vi "MainInterface.vi"() -> ()   [LabVIEW 2016]
uses:
  CurrentSwitchValues_GlobalVariable.vi
  TCPRead_Write_GlobalVariables.vi
panel:
  out "Progress #":i32
  in  "Refresh Fraction [%]":dbl=30.0 min=0.0 max=100.0 step=1.0
  in  "DNA  High RR":dbl=0.25 min=0.0 max=1.0 step=0.001
  in  "Number of Dilution Cycles":dbl=120.0
  in  "Number of Mixing Cycles Initialisation":dbl=4.0
  in  "Time between Mixing Cycles Initialisation":dbl
  in  "FB RR":dbl=0.75 min=0.0 max=1.0 step=0.001
  in  "FB":dbl=8.0 min=1.0 max=9.0 step=1.0
  in  "DNA Channel":dbl=5.0 min=1.0 max=9.0 step=1.0
  in  "Fluorophore RR":dbl min=0.0 max=1.0 step=0.001
  in  "Elution Buffer RR":dbl=0.25 min=0.0 max=1.0 step=0.001
  in  "Fluorophore":dbl=1.0 min=1.0 max=9.0 step=1.0
  in  "Elution Buffer":dbl=2.0 min=1.0 max=9.0 step=1.0
  out "Running Experiments":bool
  in  "Number of Inflow Steps":dbl=15.0
  out "Chamber 7":dbl
  out "Chamber 6":dbl
  out "Chamber 5":dbl
  out "Chamber 4":dbl
  out "Chamber 3":dbl
  out "Chamber 2":dbl
  out "Chamber 1":dbl
  out "Chamber 8":dbl
  out "Running Calibration":bool=TRUE
  out "Duration (min)":i32
  out "Refresh Ratio":dbl format="%#_13g"
  in  "Number of Mixing Cycles":dbl=4.0
  in  "Fluorophore Channel":dbl=1.0 min=1.0 max=9.0 step=1.0
  in  "Elution Buffer Channel":dbl=2.0 min=1.0 max=9.0 step=1.0
  in  "Number of Dilution Steps":dbl=10.0
  in  "Time between Mixing Cycles":dbl
  in  "Perform Initial Calibration":bool
  out "Time since \nstart (sec)":dbl format="%#_4g"
  in  "Perform \nExperiments":bool
  out "Progress":i32(slide) max=6 scale=0.0..200.0
  out "Progress":i32(slide) max=25 scale=0.0..200.0
  in  "Ring 8":bool
  in  "Ring 7":bool
  in  "Ring 6":bool
  in  "Ring 5":bool
  in  "Ring 4":bool
  in  "Ring 3":bool
  in  "Ring 2":bool
  in  "Ring 1":bool
  in  "Load 20%":bool
  in  "Fully Load Chambers":bool
  in  "Load \nChannel":dbl=1.0 min=1.0 max=9.0
  out "Time Stamp":timestamp
  out "TCP Error Out":errorcluster
  out "TCP Output":string
  in  "Flush Slow":bool
  in  "Flush \nChannel":dbl=1.0 min=1.0 max=9.0
  in  "Flush Fast":bool
  out "Time since start (sec)":dbl format="%#_4g"
  out "Cycles completed":i32(slide) max=6 scale=0.0..1.0
  in  "Interval (min)":dbl=1.0
  in  "Number Of \nMix Cycles":dbl=1.0
  in  "Mix Chambers":bool
  out "Units 7/8":u8 format="%x"
  out "Units 5/6":u8 format="%x"
  out "Units 3/4":u8 format="%x"
  out "Units 1/2":u8 format="%x"
  out "Bytes Written (Total)":i32
  out "Bytes Written (Per Command)":i32
  in  "stop":bool
  in  "30":bool
  in  "24":bool
  in  "18":bool
  in  "12":bool
  in  "29":bool
  in  "23":bool
  in  "17":bool
  in  "10":bool
  in  "27":bool
  in  "20":bool
  in  "15":bool
  in  "25":bool
  in  "19":bool
  in  "13":bool
  in  "28":bool
  in  "22":bool
  in  "16":bool
  in  "11":bool
  in  "26":bool
  in  "21":bool
  in  "14":bool
  in  "9":bool
  in  "8":bool
  in  "6":bool
  in  "4":bool
  in  "2":bool
  in  "7":bool
  in  "5":bool
  in  "3":bool
  in  "1":bool
  in  "Timeout (ms)":u16=25
  in  "Port":u16=502
  in  "Address":string="192.168.1.100"
  # "Experimental Sequence"
  # "Air Filled Control Lines"
  # "Multiplexer"
  # "Inflow Speed Regulators"
  # "Ring Control"
  # "Misc."
  # "Channel Selection"
  # "Set Desired RR"
  # "Low Pressure Control \nchalles 4-8 Should Remain \nUnused. If Additional Air \nLines Are Required, The \nValves Can Be Found Under \nThis Tile."
  # "A Total Of 30 Valves (And \nThus Switches) Exist.\nCurrent Microfluidic Devices\nOnly Require 24 Control \nLines. As Such Valve 30 Has \nBeen Relegated."
  # "RRs for Multiple DNA Concentrations"
  # "Hexadceimal Values for WAGO Units 1-2, 3-4, 5-6, 7-8"
  # "Mixing Processes"
  # "Flushing"
  # "Loading"
  # "Perform Initial Calibration"
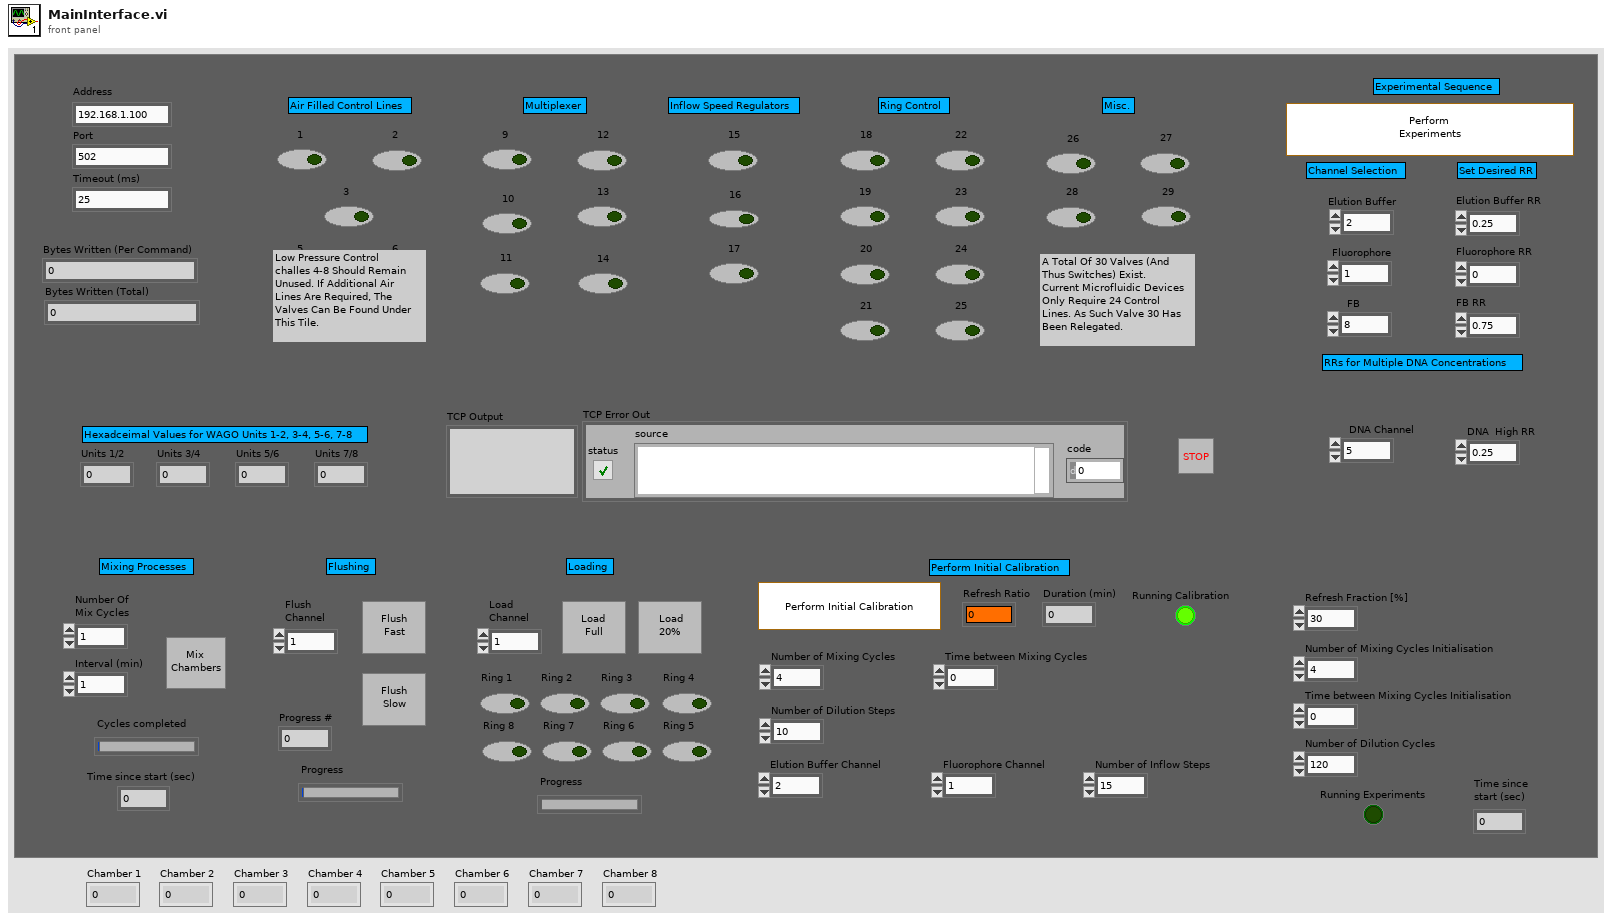
[diagram p1: front panel]
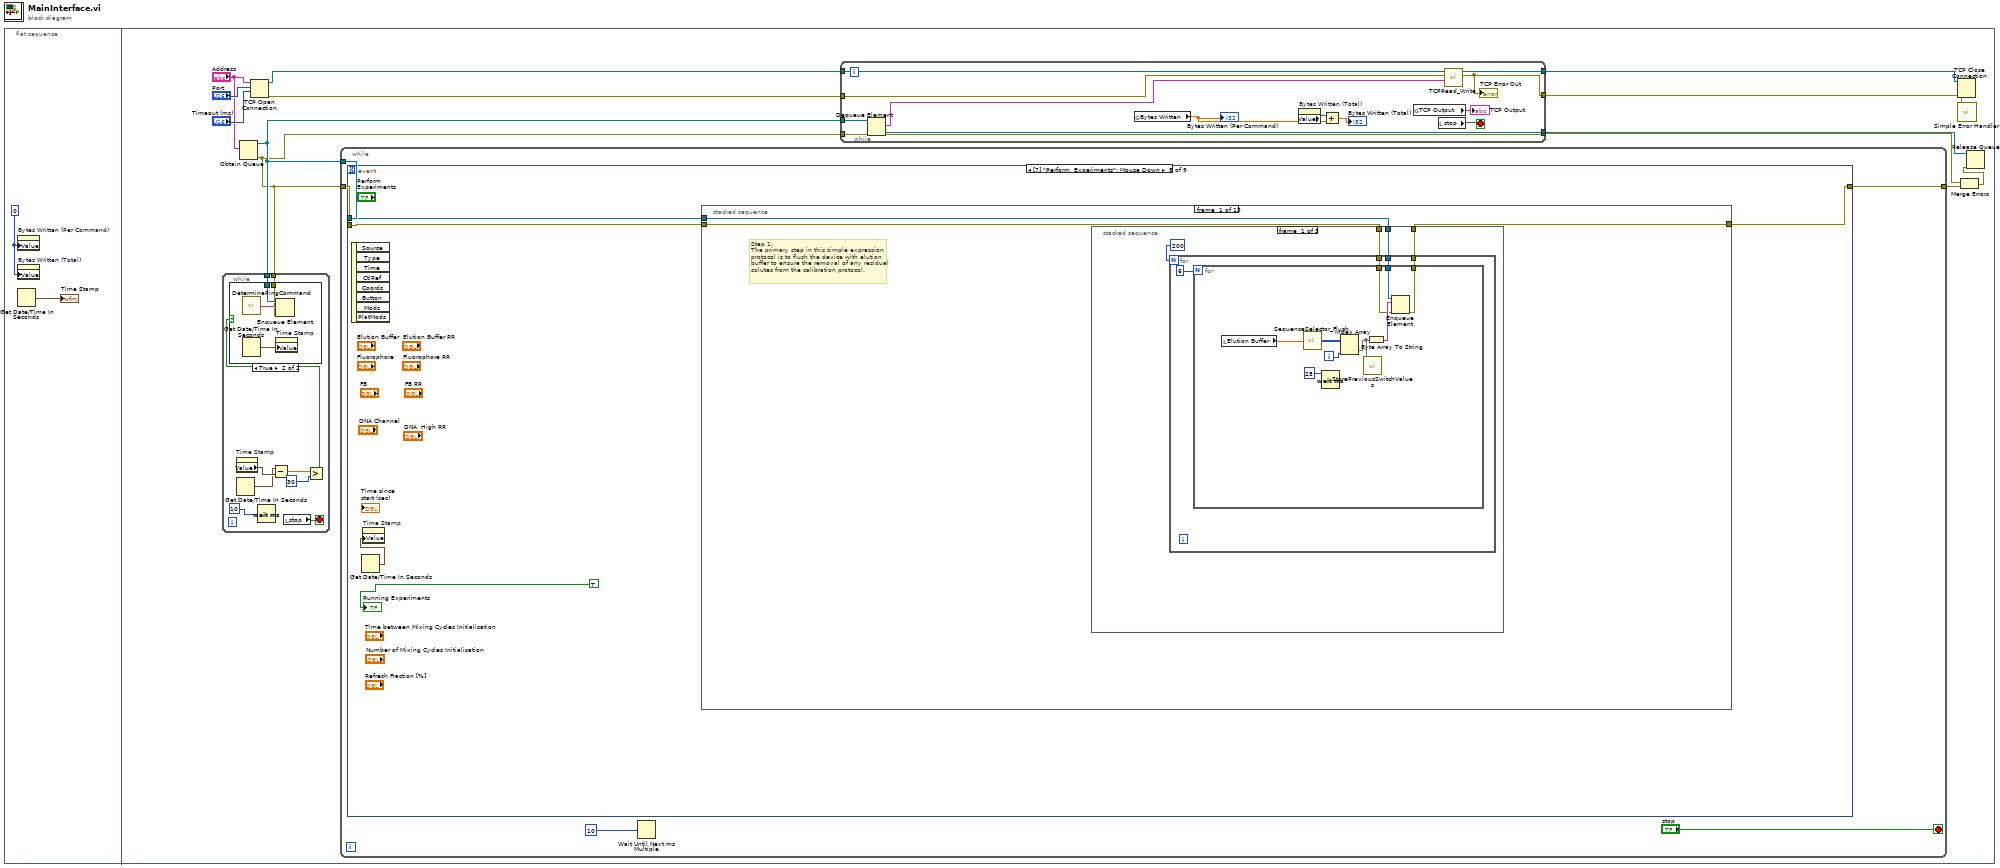
[diagram p0: block diagram]
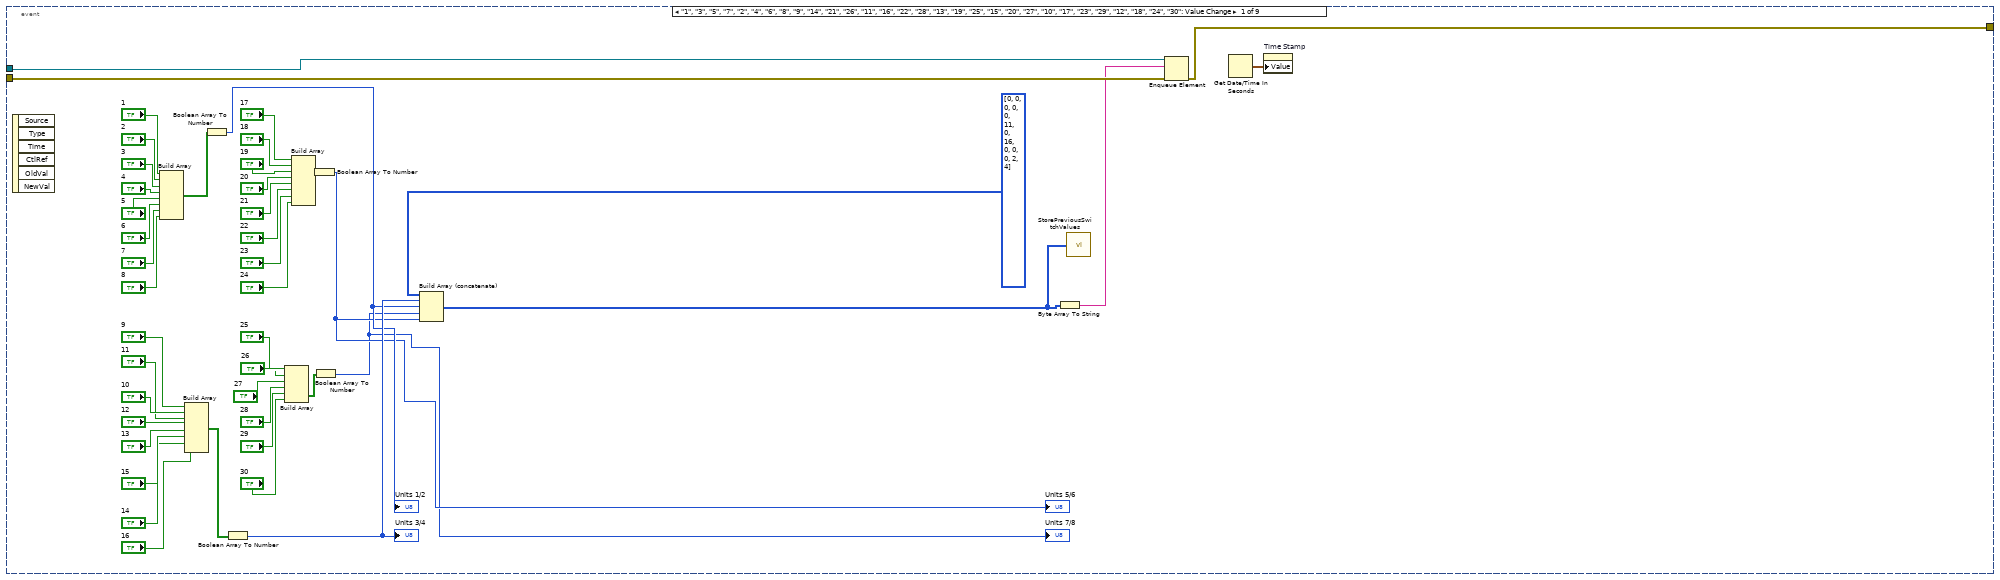
[diagram p3: hidden frame]
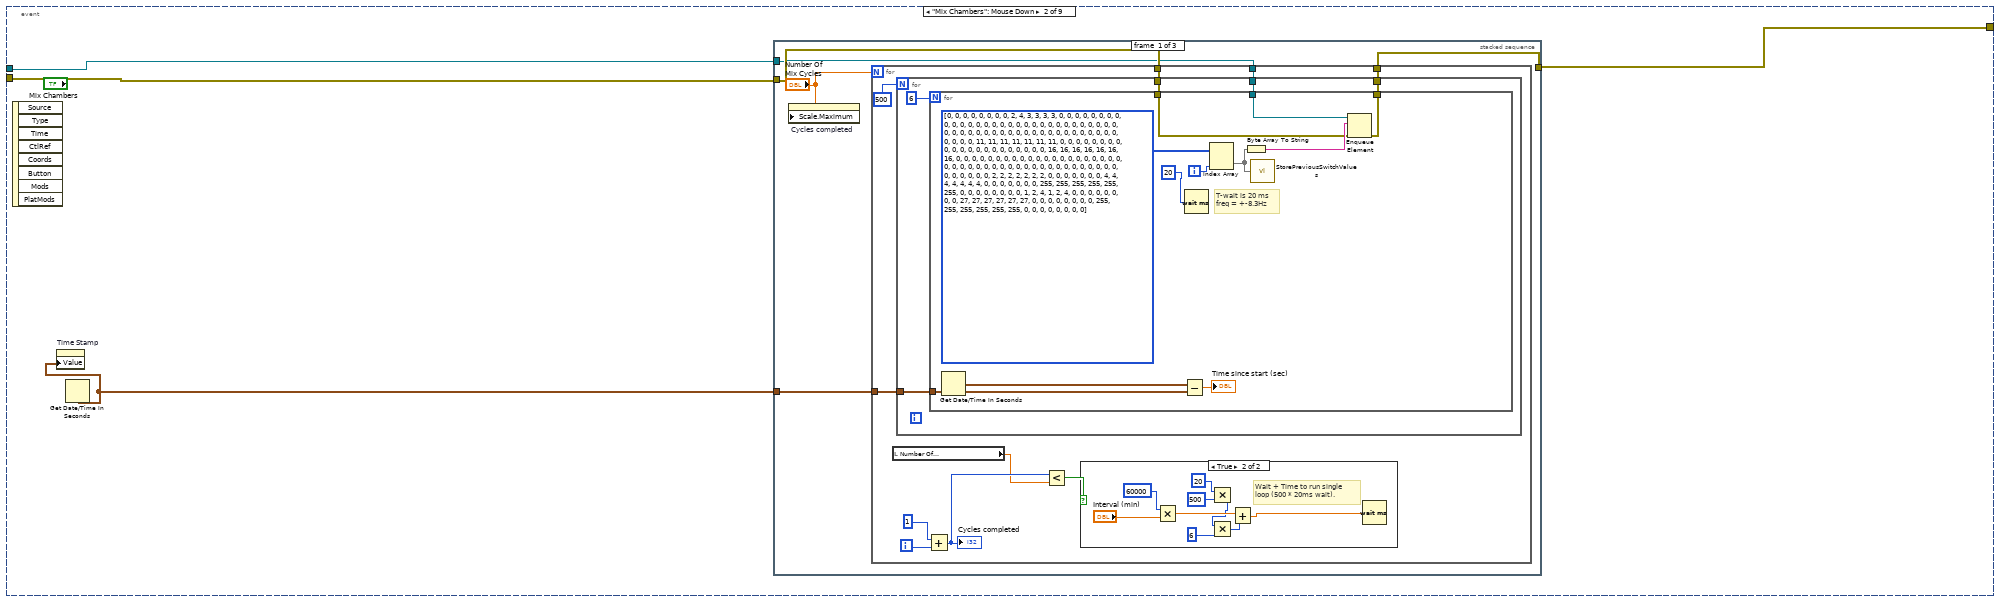
[diagram p4: hidden frame]
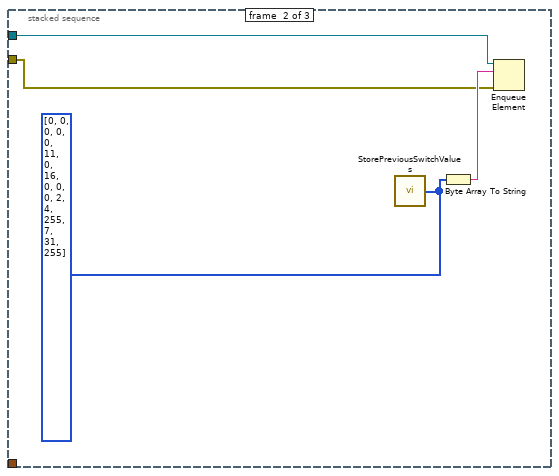
[diagram p6: hidden frame]
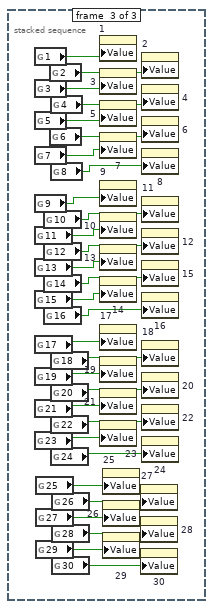
[diagram p7: hidden frame]
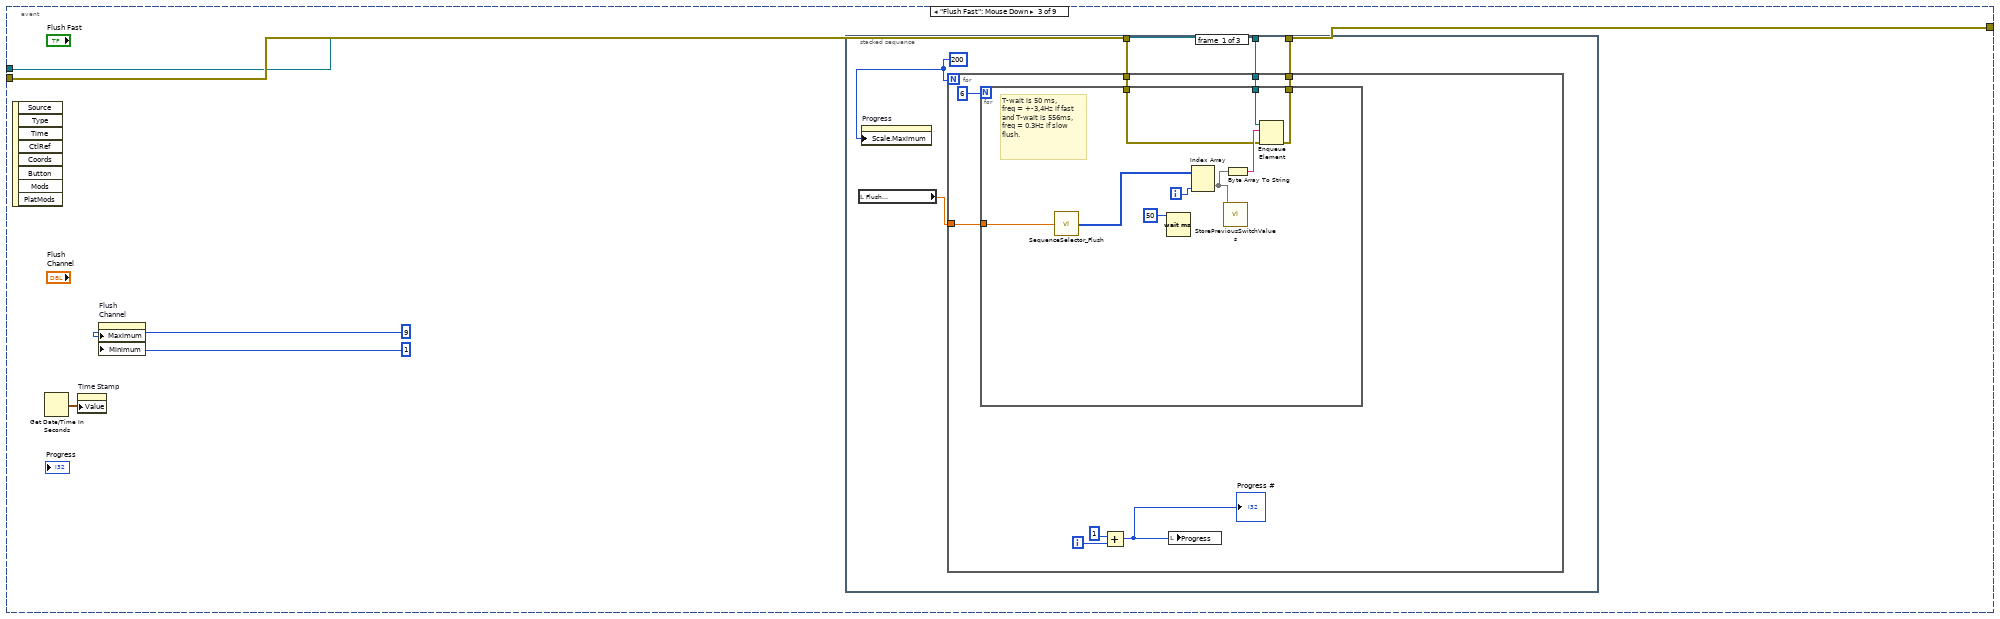
[diagram p8: hidden frame]
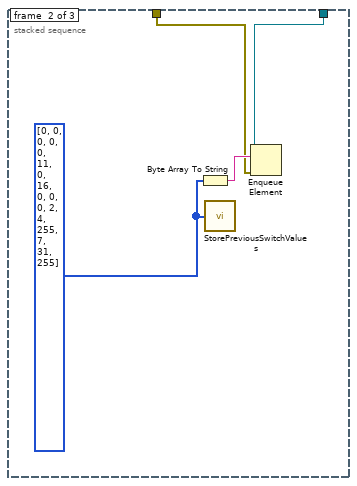
[diagram p9: hidden frame]
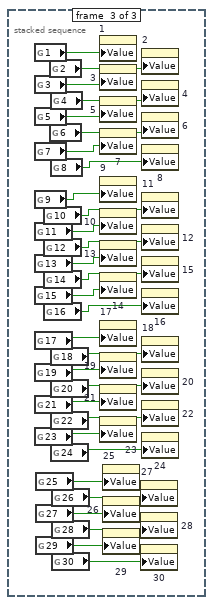
[diagram p10: hidden frame]
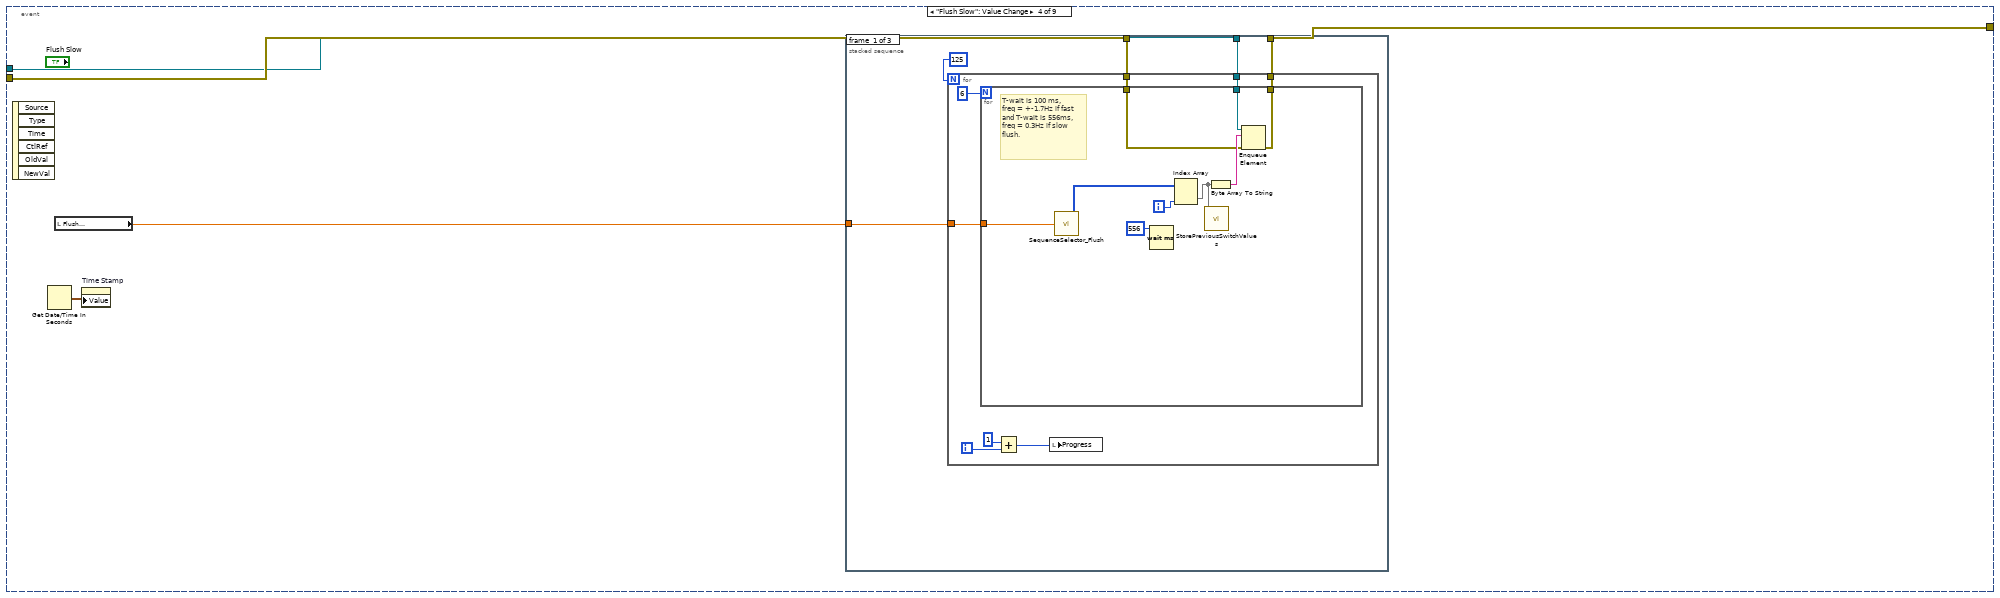
[diagram p11: hidden frame]
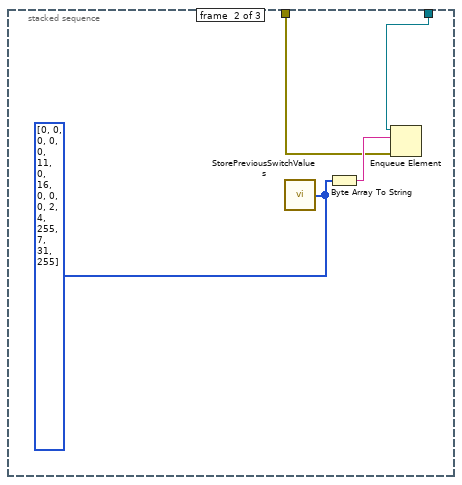
[diagram p12: hidden frame]
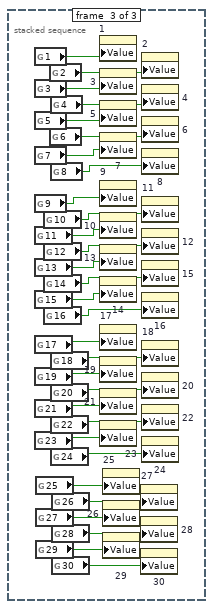
[diagram p13: hidden frame]
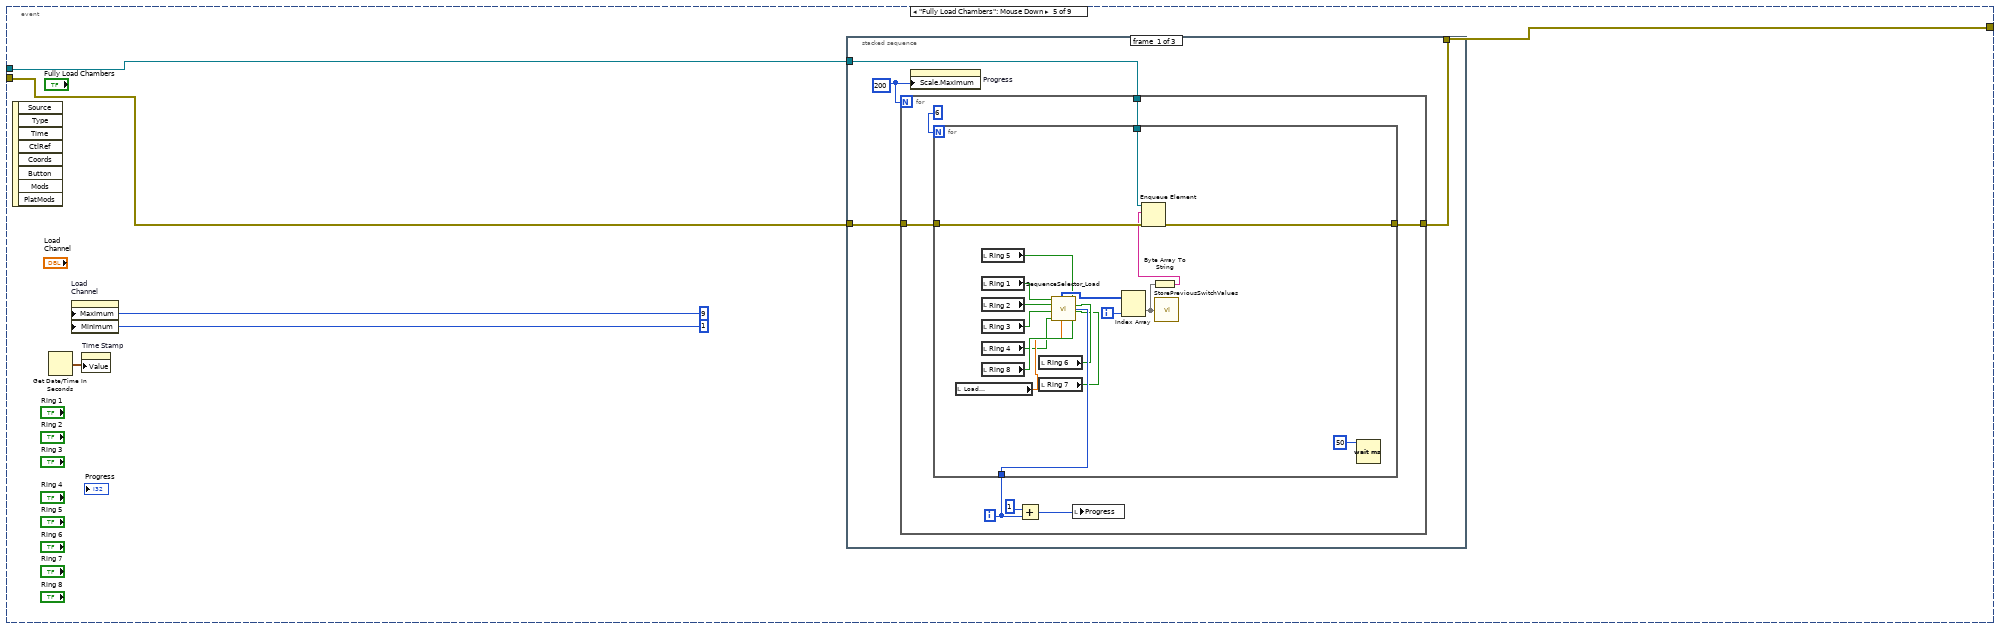
[diagram p14: hidden frame]
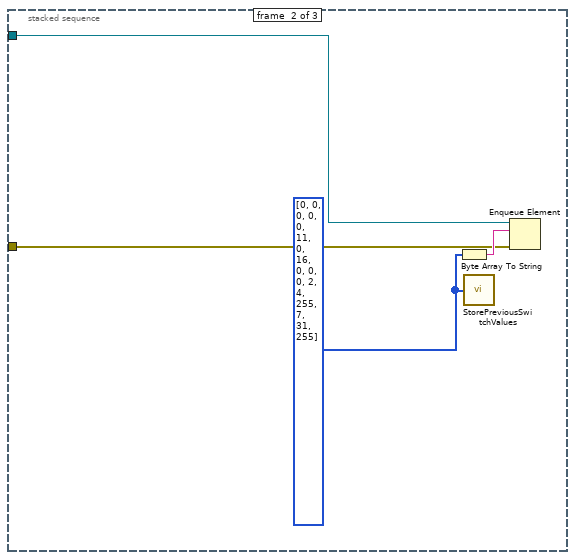
[diagram p15: hidden frame]
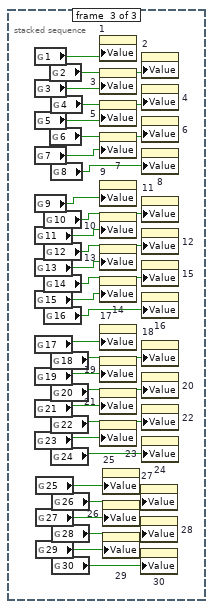
[diagram p16: hidden frame]
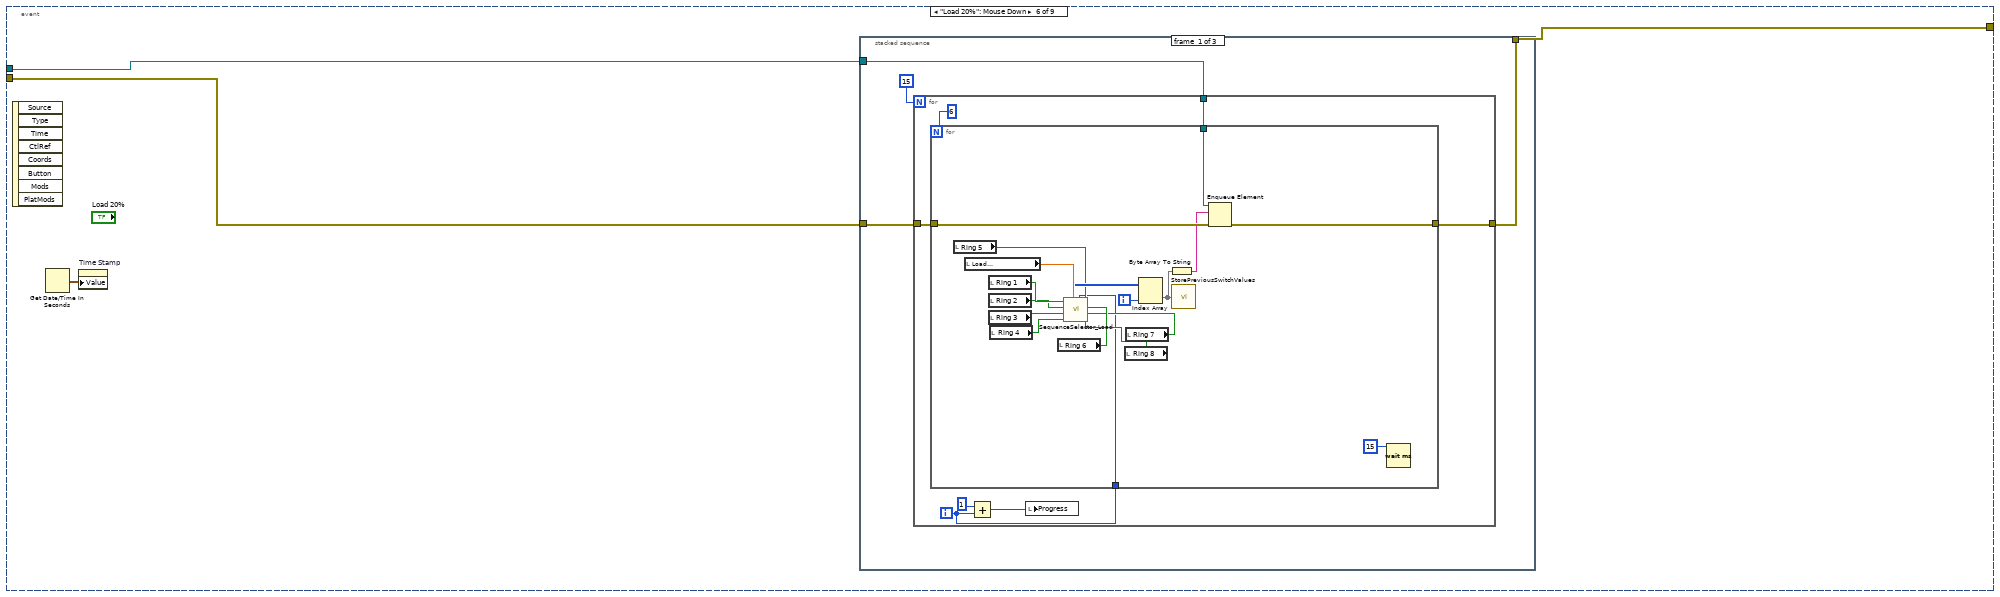
[diagram p17: hidden frame]
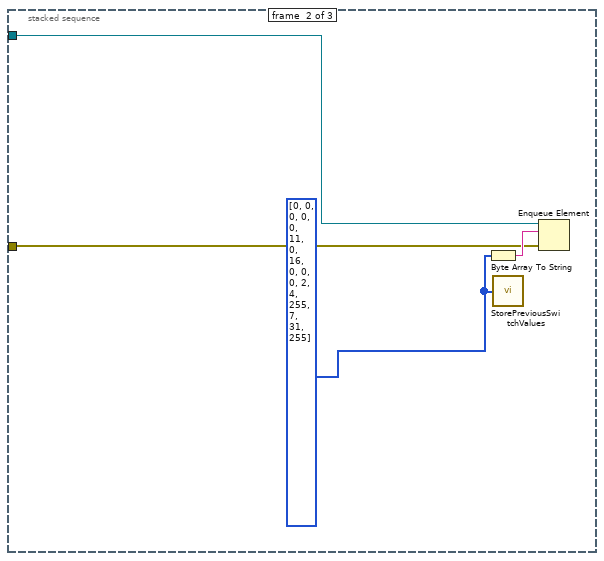
[diagram p18: hidden frame]
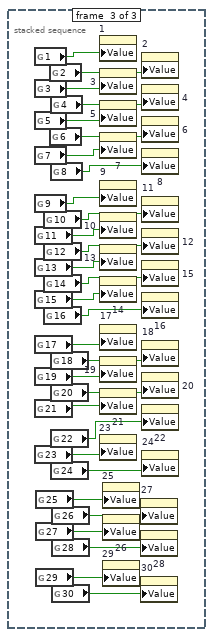
[diagram p19: hidden frame]
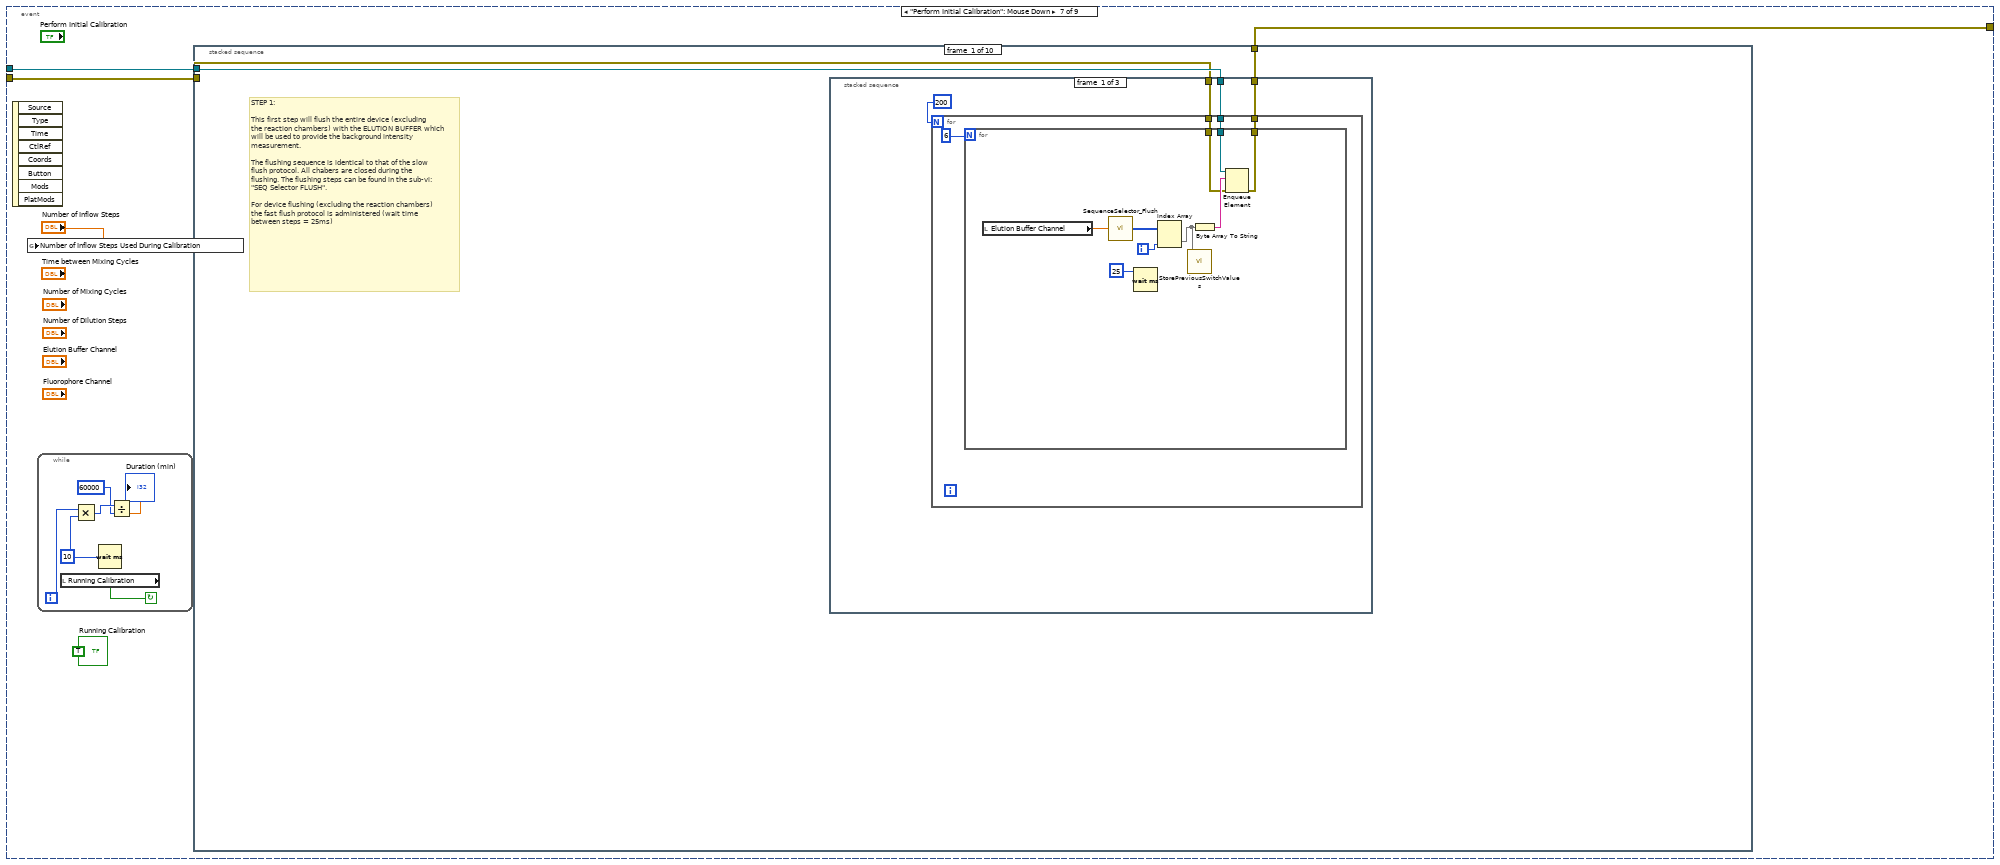
[diagram p20: hidden frame]
diagram:
  n1 = flat-sequence {
    frame #0 {
      w2 = 0
      n2 = property on="Bytes Written (Per Command)" class="DigNum (strict)"("Value"=w2) -> ()  [unwired: 2 in, 2 out]
      n3 = property on="Bytes Written (Total)" class="DigNum (strict)"("Value"=w2) -> ()  [unwired: 2 in, 2 out]
      n4 = Get Date/Time In Seconds() -> (seconds since 1Jan1904=→"Time Stamp":timestamp)
    }
    frame #1 {
      n5 = Obtain Queue(element data type="Address") -> (queue out=w4:refnum<queue>, error out=w3:errorcluster)  [unwired: 4 in, 1 out]
      n6 = while {
        tunnel: w4 -> [w22]
        tunnel: w3 -> [w21]
        stop <- w20 stop-if-true
        n7 = property on="Time Stamp" class="AbsTime (strict)"() -> ("Value"=w25:timestamp)  [unwired: 2 in, 2 out]
        n8 = Get Date/Time In Seconds() -> (seconds since 1Jan1904=w17:timestamp)
        n9 = Wait (ms)(milliseconds to wait=10) -> ()  [unwired: 1 out]
        n10 = Subtract(x=w17, y=w25) -> (x-y=w18:dbl)
        n11 = local read "stop"() -> (w20:bool)
        n12 = Greater?(x=w18, y=30) -> (0:w23:bool)
        n13 = case shown="True" w23 {
          tunnel: w22 -> [_ w28]
          tunnel: w21 -> [_ w27]
          frame False {
          }
          frame True {
            n14 = call "DeterminePingCommand.vi"() -> ("String"=w29:string)
            n15 = Get Date/Time In Seconds() -> (seconds since 1Jan1904=w26:timestamp)
            n16 = Enqueue Element(queue=w28, element=w29, error in (no error)=w27) -> ()  [unwired: 1 in, 3 out]
            n17 = property on="Time Stamp" class="AbsTime (strict)"("Value"=w26) -> ()  [unwired: 2 in, 2 out]
          }
        }
      }
      n18 = TCP Open Connection(address="Address", remote port or service name="Port", timeout ms (60000)="Timeout (ms)") -> (connection ID=w10:refnum<k5>, error out=w9:errorcluster)  [unwired: 2 in]
      n19 = while {
        tunnel: w4 -> [w47]
        tunnel: w3 -> [w46]
        tunnel: [w45] -> w13
        stop <- "stop" stop-if-true
        n20 = event shown="[7] \"Perform  Experiments\": Mouse Down" {
          selector: _ -> [_ _ _ _ _ _ _ _ _]
          dyn-events: _ -> [_ _ _ _ _ _ _ _ _]
          timeout: _ -> [_ _ _ _ _ _ _ _ _]
          tunnel: w47 -> [w57 w96 w174 w236 w298 w366 w434 w923 w2194]
          tunnel: w46 -> [w58 w97 w175 w237 w297 w365 w435 w924 w2192]
          tunnel: [w59 w95 w173 w235 w296 w364 w433 w922 w2191] -> w45
          event "1", "3", "5", "7", "2", "4", "6", "8", "9", "14", "21", "26", "11", "16", "22", "28", "13", "19", "25", "15", "20", "27", "10", "17", "23", "29", "12", "18", "24", "30": Value Change {
            n21 = event-data() -> ()  [unwired: 1 in, 6 out]
            n22 = Build Array "Build Array"("1", "2", "3", "4", "5", "6", "7", "8") -> (w92:bool[])
            n23 = Build Array "Build Array"("9", "10", "11", "12", "13", "14", "15", "16") -> (w93:bool[])
            n24 = Boolean Array To Number(Boolean array=w92) -> (number=w63:u32)
            "Units 1/2" <- w63
            n25 = Boolean Array To Number(Boolean array=w93) -> (number=w64:u32)
            "Units 3/4" <- w64
            n26 = Build Array "Build Array"("25", "26", "27", "28", "29", "30") -> (w90:bool[])
            n27 = Build Array "Build Array"("17", "18", "19", "20", "21", "22", "23", "24") -> (w91:bool[])
            n28 = Boolean Array To Number(Boolean array=w91) -> (number=w62:u32)
            "Units 5/6" <- w62
            n29 = Boolean Array To Number(Boolean array=w90) -> (number=w61:u32)
            "Units 7/8" <- w61
            n30 = Build Array (concatenate)(u8[] [0, 0, 0, 0, 0, 11, 0, 16, 0, 0, 0, 2, 4], w64, w63, w61, w62) -> (w65:u32[])
            n31 = Byte Array To String(unsigned byte array=w65) -> (string=w56:string)
            n32 = call "StorePreviousSwitchValues.vi"("Array"=w65) -> ()  [unwired: 3 in]
            n33 = Enqueue Element(queue=w57, element=w56, error in (no error)=w58) -> (error out=w59:errorcluster)  [unwired: 1 in, 2 out]
            n34 = Get Date/Time In Seconds() -> (seconds since 1Jan1904=w55:timestamp)
            n35 = property on="Time Stamp" class="AbsTime (strict)"("Value"=w55) -> ()  [unwired: 2 in, 2 out]
          }
          event "Mix Chambers": Mouse Down {
            n36 = event-data() -> ()  [unwired: 1 in, 8 out]
            n37 = Get Date/Time In Seconds() -> (seconds since 1Jan1904=w94:timestamp)
            n38 = property on="Time Stamp" class="AbsTime (strict)"("Value"=w94) -> ()  [unwired: 2 in, 2 out]
            n39 = stacked-sequence {
              tunnel: w94 -> [w101 _ _]
              tunnel: w97 -> [w100 w139 _]
              tunnel: w96 -> [w99 w138 _]
              tunnel: [w98 _ _] -> w95
              frame #0 {
                n40 = property on="Cycles completed" class="Slide (strict)"("Scale.Maximum"="Number Of \nMix Cycles") -> ()  [unwired: 2 in, 2 out]
                n41 = for {
                  N: "Number Of \nMix Cycles" -> [_]
                  tunnel: w101 -> [w109]
                  tunnel: w100 -> [w105]
                  tunnel: w99 -> [w104]
                  tunnel: [w103] -> w98
                  i -> [w112]
                  n42 = local read "Number Of \nMix Cycles"() -> (w106:dbl)
                  n43 = for {
                    N: 500 -> [_]
                    tunnel: w109 -> [w125]
                    tunnel: w105 -> [w124]
                    tunnel: w104 -> [w123]
                    tunnel: [w122] -> w103
                    n44 = for {
                      N: 6 -> [_]
                      tunnel: w125 -> [w132]
                      tunnel: w124 -> [w130]
                      tunnel: w123 -> [w129]
                      tunnel: [w128] -> w122
                      i -> [w135]
                      # "T-wait is 20 ms\nfreq = +-8.3Hz"
                      n45 = Get Date/Time In Seconds() -> (seconds since 1Jan1904=w133:timestamp)
                      n46 = Subtract(x=w133, y=w132) -> (x-y=→"Time since start (sec)":dbl)
                      n47 = Wait (ms)(milliseconds to wait=20) -> ()  [unwired: 1 out]
                      n48 = Index Array(array=u8[][] [[0, 0, 0, 0, 0, 0, 0, 0, 2, 4, 3, 3, 3, 3], [0, 0, 0, 0, 0, 0, 0, 0, 0, 0, 0, 0, 0, 0], [0, 0, 0, 0, 0, 0, 0, 0, 0, 0, 0, 0, 0, 0], [0, 0, 0, 0, 0, 0, 0, 0, 0, 0, 0, 0, 0, 0], [0, 0, 0, 0, 0, 0, 0, 0, 0, 0, 0, 0, 0, 0], [11, 11, 11, 11, 11, 11, 11, 0, 0, 0, 0, 0, 0, 0], [0, 0, 0, 0, 0, 0, 0, 0, 0, 0, 0, 0, 0, 0], [16, 16, 16, 16, 16, 16, 16, 0, 0, 0, 0, 0, 0, 0], [0, 0, 0, 0, 0, 0, 0, 0, 0, 0, 0, 0, 0, 0], [0, 0, 0, 0, 0, 0, 0, 0, 0, 0, 0, 0, 0, 0], [0, 0, 0, 0, 0, 0, 0, 0, 0, 0, 0, 0, 0, 0], [2, 2, 2, 2, 2, 2, 2, 0, 0, 0, 0, 0, 0, 0], [4, 4, 4, 4, 4, 4, 4, 0, 0, 0, 0, 0, 0, 0], [255, 255, 255, 255, 255, 255, 0, 0, 0, 0, 0, 0, 0, 0], [1, 2, 4, 1, 2, 4, 0, 0, 0, 0, 0, 0, 0, 0], [27, 27, 27, 27, 27, 27, 0, 0, 0, 0, 0, 0, 0, 0], [255, 255, 255, 255, 255, 255, 0, 0, 0, 0, 0, 0, 0, 0]], index (col)=w135) -> (element=w136:u8[])  [unwired: 1 in]
                      n49 = Byte Array To String(unsigned byte array=w136) -> (string=w131:string)
                      n50 = call "StorePreviousSwitchValues.vi"("Array"=w136) -> ()  [unwired: 3 in]
                      n51 = Enqueue Element(queue=w129, element=w131, error in (no error)=w130) -> (error out=w128:errorcluster)  [unwired: 1 in, 2 out]
                    }
                  }
                  n52 = Add(x=1, y=w112) -> (x+y=w107:i32)
                  "Cycles completed" <- w107
                  n53 = Less?(x=w107, y=w106) -> (x < y?=w108:bool)
                  n54 = case shown="True" w108 {
                    frame False {
                    }
                    frame True {
                      # "Wait + Time to run single\nloop (500 * 20ms wait)."
                      n55 = Multiply(x=60000, y="Interval (min)") -> (x*y=w119:dbl)
                      n56 = Multiply(x=20, y=500) -> (x*y=w115:i32)
                      n57 = Multiply(x=w115, y=6) -> (x*y=w114:i32)
                      n58 = Add(x=w119, y=w114) -> (x+y=w118:dbl)
                      n59 = Wait (ms)(milliseconds to wait=w118) -> ()  [unwired: 1 out]
                    }
                  }
                }
              }
              frame #1 {
                w141 = u8[] [0, 0, 0, 0, 0, 11, 0, 16, 0, 0, 0, 2, 4, 255, 7, 31, 255]
                n60 = call "StorePreviousSwitchValues.vi"("Array"=w141) -> ()  [unwired: 3 in]
                n61 = Byte Array To String(unsigned byte array=w141) -> (string=w140:string)
                n62 = Enqueue Element(queue=w138, element=w140, error in (no error)=w139) -> ()  [unwired: 1 in, 3 out]
              }
              frame #2 {
                n63 = global read "CurrentSwitchValues_GlobalVariable.vi" "1"() -> (w171:bool)
                n64 = global read "CurrentSwitchValues_GlobalVariable.vi" "3"() -> (w164:bool)
                n65 = global read "CurrentSwitchValues_GlobalVariable.vi" "5"() -> (w166:bool)
                n66 = global read "CurrentSwitchValues_GlobalVariable.vi" "7"() -> (w168:bool)
                n67 = global read "CurrentSwitchValues_GlobalVariable.vi" "9"() -> (w156:bool)
                n68 = global read "CurrentSwitchValues_GlobalVariable.vi" "11"() -> (w158:bool)
                n69 = global read "CurrentSwitchValues_GlobalVariable.vi" "13"() -> (w160:bool)
                n70 = global read "CurrentSwitchValues_GlobalVariable.vi" "15"() -> (w162:bool)
                n71 = global read "CurrentSwitchValues_GlobalVariable.vi" "17"() -> (w148:bool)
                n72 = global read "CurrentSwitchValues_GlobalVariable.vi" "19"() -> (w150:bool)
                n73 = global read "CurrentSwitchValues_GlobalVariable.vi" "21"() -> (w152:bool)
                n74 = global read "CurrentSwitchValues_GlobalVariable.vi" "23"() -> (w154:bool)
                n75 = global read "CurrentSwitchValues_GlobalVariable.vi" "25"() -> (w147:bool)
                n76 = global read "CurrentSwitchValues_GlobalVariable.vi" "27"() -> (w145:bool)
                n77 = global read "CurrentSwitchValues_GlobalVariable.vi" "29"() -> (w143:bool)
                n78 = global read "CurrentSwitchValues_GlobalVariable.vi" "10"() -> (w157:bool)
                n79 = global read "CurrentSwitchValues_GlobalVariable.vi" "12"() -> (w159:bool)
                n80 = global read "CurrentSwitchValues_GlobalVariable.vi" "14"() -> (w161:bool)
                n81 = global read "CurrentSwitchValues_GlobalVariable.vi" "16"() -> (w163:bool)
                n82 = global read "CurrentSwitchValues_GlobalVariable.vi" "2"() -> (w170:bool)
                n83 = global read "CurrentSwitchValues_GlobalVariable.vi" "6"() -> (w167:bool)
                n84 = global read "CurrentSwitchValues_GlobalVariable.vi" "4"() -> (w165:bool)
                n85 = global read "CurrentSwitchValues_GlobalVariable.vi" "8"() -> (w169:bool)
                n86 = global read "CurrentSwitchValues_GlobalVariable.vi" "18"() -> (w149:bool)
                n87 = global read "CurrentSwitchValues_GlobalVariable.vi" "20"() -> (w151:bool)
                n88 = global read "CurrentSwitchValues_GlobalVariable.vi" "22"() -> (w153:bool)
                n89 = global read "CurrentSwitchValues_GlobalVariable.vi" "24"() -> (w155:bool)
                n90 = global read "CurrentSwitchValues_GlobalVariable.vi" "26"() -> (w146:bool)
                n91 = global read "CurrentSwitchValues_GlobalVariable.vi" "28"() -> (w144:bool)
                n92 = global read "CurrentSwitchValues_GlobalVariable.vi" "30"() -> (w142:bool)
                n93 = property on="1" class="Bool (strict)"("Value"=w171) -> ()  [unwired: 2 in, 2 out]
                n94 = property on="3" class="Bool (strict)"("Value"=w164) -> ()  [unwired: 2 in, 2 out]
                n95 = property on="5" class="Bool (strict)"("Value"=w166) -> ()  [unwired: 2 in, 2 out]
                n96 = property on="7" class="Bool (strict)"("Value"=w168) -> ()  [unwired: 2 in, 2 out]
                n97 = property on="9" class="Bool (strict)"("Value"=w156) -> ()  [unwired: 2 in, 2 out]
                n98 = property on="10" class="Bool (strict)"("Value"=w158) -> ()  [unwired: 2 in, 2 out]
                n99 = property on="13" class="Bool (strict)"("Value"=w160) -> ()  [unwired: 2 in, 2 out]
                n100 = property on="14" class="Bool (strict)"("Value"=w162) -> ()  [unwired: 2 in, 2 out]
                n101 = property on="17" class="Bool (strict)"("Value"=w148) -> ()  [unwired: 2 in, 2 out]
                n102 = property on="19" class="Bool (strict)"("Value"=w150) -> ()  [unwired: 2 in, 2 out]
                n103 = property on="21" class="Bool (strict)"("Value"=w152) -> ()  [unwired: 2 in, 2 out]
                n104 = property on="23" class="Bool (strict)"("Value"=w154) -> ()  [unwired: 2 in, 2 out]
                n105 = property on="25" class="Bool (strict)"("Value"=w147) -> ()  [unwired: 2 in, 2 out]
                n106 = property on="26" class="Bool (strict)"("Value"=w145) -> ()  [unwired: 2 in, 2 out]
                n107 = property on="29" class="Bool (strict)"("Value"=w143) -> ()  [unwired: 2 in, 2 out]
                n108 = property on="27" class="Bool (strict)"("Value"=w146) -> ()  [unwired: 2 in, 2 out]
                n109 = property on="28" class="Bool (strict)"("Value"=w144) -> ()  [unwired: 2 in, 2 out]
                n110 = property on="30" class="Bool (strict)"("Value"=w142) -> ()  [unwired: 2 in, 2 out]
                n111 = property on="2" class="Bool (strict)"("Value"=w170) -> ()  [unwired: 2 in, 2 out]
                n112 = property on="4" class="Bool (strict)"("Value"=w165) -> ()  [unwired: 2 in, 2 out]
                n113 = property on="6" class="Bool (strict)"("Value"=w167) -> ()  [unwired: 2 in, 2 out]
                n114 = property on="8" class="Bool (strict)"("Value"=w169) -> ()  [unwired: 2 in, 2 out]
                n115 = property on="11" class="Bool (strict)"("Value"=w157) -> ()  [unwired: 2 in, 2 out]
                n116 = property on="12" class="Bool (strict)"("Value"=w159) -> ()  [unwired: 2 in, 2 out]
                n117 = property on="15" class="Bool (strict)"("Value"=w161) -> ()  [unwired: 2 in, 2 out]
                n118 = property on="16" class="Bool (strict)"("Value"=w163) -> ()  [unwired: 2 in, 2 out]
                n119 = property on="18" class="Bool (strict)"("Value"=w149) -> ()  [unwired: 2 in, 2 out]
                n120 = property on="20" class="Bool (strict)"("Value"=w151) -> ()  [unwired: 2 in, 2 out]
                n121 = property on="22" class="Bool (strict)"("Value"=w153) -> ()  [unwired: 2 in, 2 out]
                n122 = property on="24" class="Bool (strict)"("Value"=w155) -> ()  [unwired: 2 in, 2 out]
              }
            }
          }
          event "Flush Fast": Mouse Down {
            n123 = event-data() -> ()  [unwired: 1 in, 8 out]
            n124 = Get Date/Time In Seconds() -> (seconds since 1Jan1904=w172:timestamp)
            n125 = property on="Time Stamp" class="AbsTime (strict)"("Value"=w172) -> ()  [unwired: 2 in, 2 out]
            n126 = property on="Flush \nChannel" class="DigNum (strict)"("Maximum"=9, "Minimum"=1) -> ()  [unwired: 2 in, 2 out]
            n127 = stacked-sequence {
              tunnel: w175 -> [w181 w201 _]
              tunnel: w174 -> [w180 w200 _]
              tunnel: [w179 _ _] -> w173
              frame #0 {
                w178 = 200
                n128 = local read "Flush \nChannel"() -> (w182:dbl)
                n129 = property on="Progress" class="Slide (strict)"("Scale.Maximum"=w178) -> ()  [unwired: 2 in, 2 out]
                n130 = for {
                  N: w178 -> [_]
                  tunnel: w182 -> [w189]
                  tunnel: w181 -> [w188]
                  tunnel: w180 -> [w187]
                  tunnel: [w186] -> w179
                  i -> [w184]
                  n131 = for {
                    N: 6 -> [_]
                    tunnel: w189 -> [w197]
                    tunnel: w188 -> [w193]
                    tunnel: w187 -> [w192]
                    tunnel: [w191] -> w186
                    i -> [w198]
                    # "T-wait is 50 ms,\nfreq = +-3,4Hz if fast and T-wait is 556ms, freq = 0.3Hz if slow flush."
                    n132 = call "SequenceSelector_Flush.vi"("Inflow Channel Selector"=w197) -> ("Array"=w196:u8[][])
                    n133 = Wait (ms)(milliseconds to wait=50) -> ()  [unwired: 1 out]
                    n134 = Index Array(array=w196, index (col)=w198) -> (element=w199:u8[])  [unwired: 1 in]
                    n135 = call "StorePreviousSwitchValues.vi"("Array"=w199) -> ()  [unwired: 3 in]
                    n136 = Byte Array To String(unsigned byte array=w199) -> (string=w194:string)
                    n137 = Enqueue Element(queue=w192, element=w194, error in (no error)=w193) -> (error out=w191:errorcluster)  [unwired: 1 in, 2 out]
                  }
                  n138 = Add(x=1, y=w184) -> (x+y=w183:i32)
                  "Progress #" <- w183
                  n139 = local write "Progress"(w183) -> ()
                }
              }
              frame #1 {
                w203 = u8[] [0, 0, 0, 0, 0, 11, 0, 16, 0, 0, 0, 2, 4, 255, 7, 31, 255]
                n140 = Byte Array To String(unsigned byte array=w203) -> (string=w202:string)
                n141 = call "StorePreviousSwitchValues.vi"("Array"=w203) -> ()  [unwired: 3 in]
                n142 = Enqueue Element(queue=w200, element=w202, error in (no error)=w201) -> ()  [unwired: 1 in, 3 out]
              }
              frame #2 {
                n143 = global read "CurrentSwitchValues_GlobalVariable.vi" "1"() -> (w233:bool)
                n144 = global read "CurrentSwitchValues_GlobalVariable.vi" "3"() -> (w226:bool)
                n145 = global read "CurrentSwitchValues_GlobalVariable.vi" "5"() -> (w228:bool)
                n146 = global read "CurrentSwitchValues_GlobalVariable.vi" "7"() -> (w230:bool)
                n147 = global read "CurrentSwitchValues_GlobalVariable.vi" "9"() -> (w218:bool)
                n148 = global read "CurrentSwitchValues_GlobalVariable.vi" "11"() -> (w220:bool)
                n149 = global read "CurrentSwitchValues_GlobalVariable.vi" "13"() -> (w222:bool)
                n150 = global read "CurrentSwitchValues_GlobalVariable.vi" "15"() -> (w224:bool)
                n151 = global read "CurrentSwitchValues_GlobalVariable.vi" "17"() -> (w210:bool)
                n152 = global read "CurrentSwitchValues_GlobalVariable.vi" "19"() -> (w212:bool)
                n153 = global read "CurrentSwitchValues_GlobalVariable.vi" "21"() -> (w214:bool)
                n154 = global read "CurrentSwitchValues_GlobalVariable.vi" "23"() -> (w216:bool)
                n155 = global read "CurrentSwitchValues_GlobalVariable.vi" "25"() -> (w209:bool)
                n156 = global read "CurrentSwitchValues_GlobalVariable.vi" "27"() -> (w207:bool)
                n157 = global read "CurrentSwitchValues_GlobalVariable.vi" "29"() -> (w205:bool)
                n158 = global read "CurrentSwitchValues_GlobalVariable.vi" "10"() -> (w219:bool)
                n159 = global read "CurrentSwitchValues_GlobalVariable.vi" "12"() -> (w221:bool)
                n160 = global read "CurrentSwitchValues_GlobalVariable.vi" "14"() -> (w223:bool)
                n161 = global read "CurrentSwitchValues_GlobalVariable.vi" "16"() -> (w225:bool)
                n162 = global read "CurrentSwitchValues_GlobalVariable.vi" "2"() -> (w232:bool)
                n163 = global read "CurrentSwitchValues_GlobalVariable.vi" "6"() -> (w229:bool)
                n164 = global read "CurrentSwitchValues_GlobalVariable.vi" "4"() -> (w227:bool)
                n165 = global read "CurrentSwitchValues_GlobalVariable.vi" "8"() -> (w231:bool)
                n166 = global read "CurrentSwitchValues_GlobalVariable.vi" "18"() -> (w211:bool)
                n167 = global read "CurrentSwitchValues_GlobalVariable.vi" "20"() -> (w213:bool)
                n168 = global read "CurrentSwitchValues_GlobalVariable.vi" "22"() -> (w215:bool)
                n169 = global read "CurrentSwitchValues_GlobalVariable.vi" "24"() -> (w217:bool)
                n170 = global read "CurrentSwitchValues_GlobalVariable.vi" "26"() -> (w208:bool)
                n171 = global read "CurrentSwitchValues_GlobalVariable.vi" "28"() -> (w206:bool)
                n172 = global read "CurrentSwitchValues_GlobalVariable.vi" "30"() -> (w204:bool)
                n173 = property on="1" class="Bool (strict)"("Value"=w233) -> ()  [unwired: 2 in, 2 out]
                n174 = property on="3" class="Bool (strict)"("Value"=w226) -> ()  [unwired: 2 in, 2 out]
                n175 = property on="5" class="Bool (strict)"("Value"=w228) -> ()  [unwired: 2 in, 2 out]
                n176 = property on="7" class="Bool (strict)"("Value"=w230) -> ()  [unwired: 2 in, 2 out]
                n177 = property on="9" class="Bool (strict)"("Value"=w218) -> ()  [unwired: 2 in, 2 out]
                n178 = property on="10" class="Bool (strict)"("Value"=w220) -> ()  [unwired: 2 in, 2 out]
                n179 = property on="13" class="Bool (strict)"("Value"=w222) -> ()  [unwired: 2 in, 2 out]
                n180 = property on="14" class="Bool (strict)"("Value"=w224) -> ()  [unwired: 2 in, 2 out]
                n181 = property on="17" class="Bool (strict)"("Value"=w210) -> ()  [unwired: 2 in, 2 out]
                n182 = property on="19" class="Bool (strict)"("Value"=w212) -> ()  [unwired: 2 in, 2 out]
                n183 = property on="21" class="Bool (strict)"("Value"=w214) -> ()  [unwired: 2 in, 2 out]
                n184 = property on="23" class="Bool (strict)"("Value"=w216) -> ()  [unwired: 2 in, 2 out]
                n185 = property on="25" class="Bool (strict)"("Value"=w209) -> ()  [unwired: 2 in, 2 out]
                n186 = property on="26" class="Bool (strict)"("Value"=w207) -> ()  [unwired: 2 in, 2 out]
                n187 = property on="29" class="Bool (strict)"("Value"=w205) -> ()  [unwired: 2 in, 2 out]
                n188 = property on="27" class="Bool (strict)"("Value"=w208) -> ()  [unwired: 2 in, 2 out]
                n189 = property on="28" class="Bool (strict)"("Value"=w206) -> ()  [unwired: 2 in, 2 out]
                n190 = property on="30" class="Bool (strict)"("Value"=w204) -> ()  [unwired: 2 in, 2 out]
                n191 = property on="2" class="Bool (strict)"("Value"=w232) -> ()  [unwired: 2 in, 2 out]
                n192 = property on="4" class="Bool (strict)"("Value"=w227) -> ()  [unwired: 2 in, 2 out]
                n193 = property on="6" class="Bool (strict)"("Value"=w229) -> ()  [unwired: 2 in, 2 out]
                n194 = property on="8" class="Bool (strict)"("Value"=w231) -> ()  [unwired: 2 in, 2 out]
                n195 = property on="11" class="Bool (strict)"("Value"=w219) -> ()  [unwired: 2 in, 2 out]
                n196 = property on="12" class="Bool (strict)"("Value"=w221) -> ()  [unwired: 2 in, 2 out]
                n197 = property on="15" class="Bool (strict)"("Value"=w223) -> ()  [unwired: 2 in, 2 out]
                n198 = property on="16" class="Bool (strict)"("Value"=w225) -> ()  [unwired: 2 in, 2 out]
                n199 = property on="18" class="Bool (strict)"("Value"=w211) -> ()  [unwired: 2 in, 2 out]
                n200 = property on="20" class="Bool (strict)"("Value"=w213) -> ()  [unwired: 2 in, 2 out]
                n201 = property on="22" class="Bool (strict)"("Value"=w215) -> ()  [unwired: 2 in, 2 out]
                n202 = property on="24" class="Bool (strict)"("Value"=w217) -> ()  [unwired: 2 in, 2 out]
              }
            }
          }
          event "Flush Slow": Value Change {
            n203 = event-data() -> ()  [unwired: 1 in, 6 out]
            n204 = Get Date/Time In Seconds() -> (seconds since 1Jan1904=w234:timestamp)
            n205 = local read "Flush \nChannel"() -> (w238:dbl)
            n206 = property on="Time Stamp" class="AbsTime (strict)"("Value"=w234) -> ()  [unwired: 2 in, 2 out]
            n207 = stacked-sequence {
              tunnel: w238 -> [w242 _ _]
              tunnel: w237 -> [w241 w261 _]
              tunnel: w236 -> [w240 w262 _]
              tunnel: [w239 _ _] -> w235
              frame #0 {
                n208 = for {
                  N: 125 -> [_]
                  tunnel: w242 -> [w250]
                  tunnel: w241 -> [w249]
                  tunnel: w240 -> [w248]
                  tunnel: [w247] -> w239
                  i -> [w245]
                  n209 = for {
                    N: 6 -> [_]
                    tunnel: w250 -> [w256]
                    tunnel: w249 -> [w254]
                    tunnel: w248 -> [w253]
                    tunnel: [w252] -> w247
                    i -> [w259]
                    # "T-wait is 100 ms,\nfreq = +-1.7Hz if fast and T-wait is 556ms, freq = 0.3Hz if slow flush."
                    n210 = call "SequenceSelector_Flush.vi"("Inflow Channel Selector"=w256) -> ("Array"=w258:u8[][])
                    n211 = Wait (ms)(milliseconds to wait=556) -> ()  [unwired: 1 out]
                    n212 = Index Array(array=w258, index (col)=w259) -> (element=w260:u8[])  [unwired: 1 in]
                    n213 = call "StorePreviousSwitchValues.vi"("Array"=w260) -> ()  [unwired: 3 in]
                    n214 = Byte Array To String(unsigned byte array=w260) -> (string=w255:string)
                    n215 = Enqueue Element(queue=w253, element=w255, error in (no error)=w254) -> (error out=w252:errorcluster)  [unwired: 1 in, 2 out]
                  }
                  n216 = Add(x=1, y=w245) -> (x+y=w244:i32)
                  n217 = local write "Progress"(w244) -> ()
                }
              }
              frame #1 {
                w264 = u8[] [0, 0, 0, 0, 0, 11, 0, 16, 0, 0, 0, 2, 4, 255, 7, 31, 255]
                n218 = call "StorePreviousSwitchValues.vi"("Array"=w264) -> ()  [unwired: 3 in]
                n219 = Byte Array To String(unsigned byte array=w264) -> (string=w263:string)
                n220 = Enqueue Element(queue=w262, element=w263, error in (no error)=w261) -> ()  [unwired: 1 in, 3 out]
              }
              frame #2 {
                n221 = global read "CurrentSwitchValues_GlobalVariable.vi" "1"() -> (w294:bool)
                n222 = global read "CurrentSwitchValues_GlobalVariable.vi" "3"() -> (w287:bool)
                n223 = global read "CurrentSwitchValues_GlobalVariable.vi" "5"() -> (w289:bool)
                n224 = global read "CurrentSwitchValues_GlobalVariable.vi" "7"() -> (w291:bool)
                n225 = global read "CurrentSwitchValues_GlobalVariable.vi" "9"() -> (w279:bool)
                n226 = global read "CurrentSwitchValues_GlobalVariable.vi" "11"() -> (w281:bool)
                n227 = global read "CurrentSwitchValues_GlobalVariable.vi" "13"() -> (w283:bool)
                n228 = global read "CurrentSwitchValues_GlobalVariable.vi" "15"() -> (w285:bool)
                n229 = global read "CurrentSwitchValues_GlobalVariable.vi" "17"() -> (w271:bool)
                n230 = global read "CurrentSwitchValues_GlobalVariable.vi" "19"() -> (w273:bool)
                n231 = global read "CurrentSwitchValues_GlobalVariable.vi" "21"() -> (w275:bool)
                n232 = global read "CurrentSwitchValues_GlobalVariable.vi" "23"() -> (w277:bool)
                n233 = global read "CurrentSwitchValues_GlobalVariable.vi" "25"() -> (w270:bool)
                n234 = global read "CurrentSwitchValues_GlobalVariable.vi" "27"() -> (w268:bool)
                n235 = global read "CurrentSwitchValues_GlobalVariable.vi" "29"() -> (w266:bool)
                n236 = global read "CurrentSwitchValues_GlobalVariable.vi" "10"() -> (w280:bool)
                n237 = global read "CurrentSwitchValues_GlobalVariable.vi" "12"() -> (w282:bool)
                n238 = global read "CurrentSwitchValues_GlobalVariable.vi" "14"() -> (w284:bool)
                n239 = global read "CurrentSwitchValues_GlobalVariable.vi" "16"() -> (w286:bool)
                n240 = global read "CurrentSwitchValues_GlobalVariable.vi" "2"() -> (w293:bool)
                n241 = global read "CurrentSwitchValues_GlobalVariable.vi" "6"() -> (w290:bool)
                n242 = global read "CurrentSwitchValues_GlobalVariable.vi" "4"() -> (w288:bool)
                n243 = global read "CurrentSwitchValues_GlobalVariable.vi" "8"() -> (w292:bool)
                n244 = global read "CurrentSwitchValues_GlobalVariable.vi" "18"() -> (w272:bool)
                n245 = global read "CurrentSwitchValues_GlobalVariable.vi" "20"() -> (w274:bool)
                n246 = global read "CurrentSwitchValues_GlobalVariable.vi" "22"() -> (w276:bool)
                n247 = global read "CurrentSwitchValues_GlobalVariable.vi" "24"() -> (w278:bool)
                n248 = global read "CurrentSwitchValues_GlobalVariable.vi" "26"() -> (w269:bool)
                n249 = global read "CurrentSwitchValues_GlobalVariable.vi" "28"() -> (w267:bool)
                n250 = global read "CurrentSwitchValues_GlobalVariable.vi" "30"() -> (w265:bool)
                n251 = property on="1" class="Bool (strict)"("Value"=w294) -> ()  [unwired: 2 in, 2 out]
                n252 = property on="3" class="Bool (strict)"("Value"=w287) -> ()  [unwired: 2 in, 2 out]
                n253 = property on="5" class="Bool (strict)"("Value"=w289) -> ()  [unwired: 2 in, 2 out]
                n254 = property on="7" class="Bool (strict)"("Value"=w291) -> ()  [unwired: 2 in, 2 out]
                n255 = property on="9" class="Bool (strict)"("Value"=w279) -> ()  [unwired: 2 in, 2 out]
                n256 = property on="10" class="Bool (strict)"("Value"=w281) -> ()  [unwired: 2 in, 2 out]
                n257 = property on="13" class="Bool (strict)"("Value"=w283) -> ()  [unwired: 2 in, 2 out]
                n258 = property on="14" class="Bool (strict)"("Value"=w285) -> ()  [unwired: 2 in, 2 out]
                n259 = property on="17" class="Bool (strict)"("Value"=w271) -> ()  [unwired: 2 in, 2 out]
                n260 = property on="19" class="Bool (strict)"("Value"=w273) -> ()  [unwired: 2 in, 2 out]
                n261 = property on="21" class="Bool (strict)"("Value"=w275) -> ()  [unwired: 2 in, 2 out]
                n262 = property on="23" class="Bool (strict)"("Value"=w277) -> ()  [unwired: 2 in, 2 out]
                n263 = property on="25" class="Bool (strict)"("Value"=w270) -> ()  [unwired: 2 in, 2 out]
                n264 = property on="26" class="Bool (strict)"("Value"=w268) -> ()  [unwired: 2 in, 2 out]
                n265 = property on="29" class="Bool (strict)"("Value"=w266) -> ()  [unwired: 2 in, 2 out]
                n266 = property on="27" class="Bool (strict)"("Value"=w269) -> ()  [unwired: 2 in, 2 out]
                n267 = property on="28" class="Bool (strict)"("Value"=w267) -> ()  [unwired: 2 in, 2 out]
                n268 = property on="30" class="Bool (strict)"("Value"=w265) -> ()  [unwired: 2 in, 2 out]
                n269 = property on="2" class="Bool (strict)"("Value"=w293) -> ()  [unwired: 2 in, 2 out]
                n270 = property on="4" class="Bool (strict)"("Value"=w288) -> ()  [unwired: 2 in, 2 out]
                n271 = property on="6" class="Bool (strict)"("Value"=w290) -> ()  [unwired: 2 in, 2 out]
                n272 = property on="8" class="Bool (strict)"("Value"=w292) -> ()  [unwired: 2 in, 2 out]
                n273 = property on="11" class="Bool (strict)"("Value"=w280) -> ()  [unwired: 2 in, 2 out]
                n274 = property on="12" class="Bool (strict)"("Value"=w282) -> ()  [unwired: 2 in, 2 out]
                n275 = property on="15" class="Bool (strict)"("Value"=w284) -> ()  [unwired: 2 in, 2 out]
                n276 = property on="16" class="Bool (strict)"("Value"=w286) -> ()  [unwired: 2 in, 2 out]
                n277 = property on="18" class="Bool (strict)"("Value"=w272) -> ()  [unwired: 2 in, 2 out]
                n278 = property on="20" class="Bool (strict)"("Value"=w274) -> ()  [unwired: 2 in, 2 out]
                n279 = property on="22" class="Bool (strict)"("Value"=w276) -> ()  [unwired: 2 in, 2 out]
                n280 = property on="24" class="Bool (strict)"("Value"=w278) -> ()  [unwired: 2 in, 2 out]
              }
            }
          }
          event "Fully Load Chambers": Mouse Down {
            n281 = event-data() -> ()  [unwired: 1 in, 8 out]
            n282 = Get Date/Time In Seconds() -> (seconds since 1Jan1904=w295:timestamp)
            n283 = property on="Load \nChannel" class="DigNum (strict)"("Maximum"=9, "Minimum"=1) -> ()  [unwired: 2 in, 2 out]
            n284 = property on="Time Stamp" class="AbsTime (strict)"("Value"=w295) -> ()  [unwired: 2 in, 2 out]
            n285 = stacked-sequence {
              tunnel: w298 -> [w304 w330 _]
              tunnel: w297 -> [w303 w331 _]
              tunnel: [w302 _ _] -> w296
              frame #0 {
                w301 = 200
                n286 = for {
                  N: w301 -> [_]
                  tunnel: w304 -> [w311]
                  tunnel: w303 -> [w310]
                  tunnel: [w309] -> w302
                  i -> [w305]
                  n287 = for {
                    N: 6 -> [_]
                    tunnel: w311 -> [w329]
                    tunnel: w310 -> [w328]
                    tunnel: [w327] -> w309
                    tunnel: w305 -> [w321]
                    i -> [w324]
                    n288 = local read "Load \nChannel"() -> (w316:dbl)
                    n289 = local read "Ring 5"() -> (w320:bool)
                    n290 = local read "Ring 1"() -> (w312:bool)
                    n291 = local read "Ring 2"() -> (w313:bool)
                    n292 = local read "Ring 3"() -> (w314:bool)
                    n293 = local read "Ring 4"() -> (w315:bool)
                    n294 = local read "Ring 8"() -> (w317:bool)
                    n295 = local read "Ring 6"() -> (w319:bool)
                    n296 = local read "Ring 7"() -> (w318:bool)
                    n297 = call "SequenceSelector_Load.vi"("Ring 8"=w317, "Ring 7"=w318, "Ring 6"=w319, "Ring 5"=w320, "Loop Iteration"=w321, "Inflow Channel Selector"=w316, "Ring 4"=w315, "Ring 3"=w314, "Ring 2"=w313, "Ring 1"=w312) -> ("Array"=w322:u8[][])
                    n298 = Index Array(array=w322, index (col)=w324) -> (element=w323:u8[])  [unwired: 1 in]
                    n299 = Byte Array To String(unsigned byte array=w323) -> (string=w325:string)
                    n300 = Enqueue Element(queue=w329, element=w325, error in (no error)=w328) -> (error out=w327:errorcluster)  [unwired: 1 in, 2 out]
                    n301 = call "StorePreviousSwitchValues.vi"("Array"=w323) -> ()  [unwired: 3 in]
                    n302 = Wait (ms)(milliseconds to wait=50) -> ()  [unwired: 1 out]
                  }
                  n303 = Add(x=1, y=w305) -> (x+y=w306:i32)
                  n304 = local write "Progress"(w306) -> ()
                }
                n305 = property on="Progress" class="Slide (strict)"("Scale.Maximum"=w301) -> ()  [unwired: 2 in, 2 out]
              }
              frame #1 {
                w333 = u8[] [0, 0, 0, 0, 0, 11, 0, 16, 0, 0, 0, 2, 4, 255, 7, 31, 255]
                n306 = Byte Array To String(unsigned byte array=w333) -> (string=w332:string)
                n307 = call "StorePreviousSwitchValues.vi"("Array"=w333) -> ()  [unwired: 3 in]
                n308 = Enqueue Element(queue=w330, element=w332, error in (no error)=w331) -> ()  [unwired: 1 in, 3 out]
              }
              frame #2 {
                n309 = global read "CurrentSwitchValues_GlobalVariable.vi" "1"() -> (w363:bool)
                n310 = global read "CurrentSwitchValues_GlobalVariable.vi" "3"() -> (w356:bool)
                n311 = global read "CurrentSwitchValues_GlobalVariable.vi" "5"() -> (w358:bool)
                n312 = global read "CurrentSwitchValues_GlobalVariable.vi" "7"() -> (w360:bool)
                n313 = global read "CurrentSwitchValues_GlobalVariable.vi" "9"() -> (w348:bool)
                n314 = global read "CurrentSwitchValues_GlobalVariable.vi" "11"() -> (w350:bool)
                n315 = global read "CurrentSwitchValues_GlobalVariable.vi" "13"() -> (w352:bool)
                n316 = global read "CurrentSwitchValues_GlobalVariable.vi" "15"() -> (w354:bool)
                n317 = global read "CurrentSwitchValues_GlobalVariable.vi" "17"() -> (w340:bool)
                n318 = global read "CurrentSwitchValues_GlobalVariable.vi" "19"() -> (w342:bool)
                n319 = global read "CurrentSwitchValues_GlobalVariable.vi" "21"() -> (w344:bool)
                n320 = global read "CurrentSwitchValues_GlobalVariable.vi" "23"() -> (w346:bool)
                n321 = global read "CurrentSwitchValues_GlobalVariable.vi" "25"() -> (w339:bool)
                n322 = global read "CurrentSwitchValues_GlobalVariable.vi" "27"() -> (w337:bool)
                n323 = global read "CurrentSwitchValues_GlobalVariable.vi" "29"() -> (w335:bool)
                n324 = global read "CurrentSwitchValues_GlobalVariable.vi" "10"() -> (w349:bool)
                n325 = global read "CurrentSwitchValues_GlobalVariable.vi" "12"() -> (w351:bool)
                n326 = global read "CurrentSwitchValues_GlobalVariable.vi" "14"() -> (w353:bool)
                n327 = global read "CurrentSwitchValues_GlobalVariable.vi" "16"() -> (w355:bool)
                n328 = global read "CurrentSwitchValues_GlobalVariable.vi" "2"() -> (w362:bool)
                n329 = global read "CurrentSwitchValues_GlobalVariable.vi" "6"() -> (w359:bool)
                n330 = global read "CurrentSwitchValues_GlobalVariable.vi" "4"() -> (w357:bool)
                n331 = global read "CurrentSwitchValues_GlobalVariable.vi" "8"() -> (w361:bool)
                n332 = global read "CurrentSwitchValues_GlobalVariable.vi" "18"() -> (w341:bool)
                n333 = global read "CurrentSwitchValues_GlobalVariable.vi" "20"() -> (w343:bool)
                n334 = global read "CurrentSwitchValues_GlobalVariable.vi" "22"() -> (w345:bool)
                n335 = global read "CurrentSwitchValues_GlobalVariable.vi" "24"() -> (w347:bool)
                n336 = global read "CurrentSwitchValues_GlobalVariable.vi" "26"() -> (w338:bool)
                n337 = global read "CurrentSwitchValues_GlobalVariable.vi" "28"() -> (w336:bool)
                n338 = global read "CurrentSwitchValues_GlobalVariable.vi" "30"() -> (w334:bool)
                n339 = property on="1" class="Bool (strict)"("Value"=w363) -> ()  [unwired: 2 in, 2 out]
                n340 = property on="3" class="Bool (strict)"("Value"=w356) -> ()  [unwired: 2 in, 2 out]
                n341 = property on="5" class="Bool (strict)"("Value"=w358) -> ()  [unwired: 2 in, 2 out]
                n342 = property on="7" class="Bool (strict)"("Value"=w360) -> ()  [unwired: 2 in, 2 out]
                n343 = property on="9" class="Bool (strict)"("Value"=w348) -> ()  [unwired: 2 in, 2 out]
                n344 = property on="10" class="Bool (strict)"("Value"=w350) -> ()  [unwired: 2 in, 2 out]
                n345 = property on="13" class="Bool (strict)"("Value"=w352) -> ()  [unwired: 2 in, 2 out]
                n346 = property on="14" class="Bool (strict)"("Value"=w354) -> ()  [unwired: 2 in, 2 out]
                n347 = property on="17" class="Bool (strict)"("Value"=w340) -> ()  [unwired: 2 in, 2 out]
                n348 = property on="19" class="Bool (strict)"("Value"=w342) -> ()  [unwired: 2 in, 2 out]
                n349 = property on="21" class="Bool (strict)"("Value"=w344) -> ()  [unwired: 2 in, 2 out]
                n350 = property on="23" class="Bool (strict)"("Value"=w346) -> ()  [unwired: 2 in, 2 out]
                n351 = property on="25" class="Bool (strict)"("Value"=w339) -> ()  [unwired: 2 in, 2 out]
                n352 = property on="26" class="Bool (strict)"("Value"=w337) -> ()  [unwired: 2 in, 2 out]
                n353 = property on="29" class="Bool (strict)"("Value"=w335) -> ()  [unwired: 2 in, 2 out]
                n354 = property on="27" class="Bool (strict)"("Value"=w338) -> ()  [unwired: 2 in, 2 out]
                n355 = property on="28" class="Bool (strict)"("Value"=w336) -> ()  [unwired: 2 in, 2 out]
                n356 = property on="30" class="Bool (strict)"("Value"=w334) -> ()  [unwired: 2 in, 2 out]
                n357 = property on="2" class="Bool (strict)"("Value"=w362) -> ()  [unwired: 2 in, 2 out]
                n358 = property on="4" class="Bool (strict)"("Value"=w357) -> ()  [unwired: 2 in, 2 out]
                n359 = property on="6" class="Bool (strict)"("Value"=w359) -> ()  [unwired: 2 in, 2 out]
                n360 = property on="8" class="Bool (strict)"("Value"=w361) -> ()  [unwired: 2 in, 2 out]
                n361 = property on="11" class="Bool (strict)"("Value"=w349) -> ()  [unwired: 2 in, 2 out]
                n362 = property on="12" class="Bool (strict)"("Value"=w351) -> ()  [unwired: 2 in, 2 out]
                n363 = property on="15" class="Bool (strict)"("Value"=w353) -> ()  [unwired: 2 in, 2 out]
                n364 = property on="16" class="Bool (strict)"("Value"=w355) -> ()  [unwired: 2 in, 2 out]
                n365 = property on="18" class="Bool (strict)"("Value"=w341) -> ()  [unwired: 2 in, 2 out]
                n366 = property on="20" class="Bool (strict)"("Value"=w343) -> ()  [unwired: 2 in, 2 out]
                n367 = property on="22" class="Bool (strict)"("Value"=w345) -> ()  [unwired: 2 in, 2 out]
                n368 = property on="24" class="Bool (strict)"("Value"=w347) -> ()  [unwired: 2 in, 2 out]
              }
            }
          }
          event "Load 20%": Mouse Down {
            n369 = event-data() -> ()  [unwired: 1 in, 8 out]
            n370 = Get Date/Time In Seconds() -> (seconds since 1Jan1904=w367:timestamp)
            n371 = property on="Time Stamp" class="AbsTime (strict)"("Value"=w367) -> ()  [unwired: 2 in, 2 out]
            n372 = stacked-sequence {
              tunnel: w366 -> [w371 w397 _]
              tunnel: w365 -> [w370 w398 _]
              tunnel: [w369 _ _] -> w364
              frame #0 {
                n373 = for {
                  N: 15 -> [_]
                  tunnel: w371 -> [w378]
                  tunnel: w370 -> [w377]
                  tunnel: [w376] -> w369
                  i -> [w372]
                  n374 = for {
                    N: 6 -> [_]
                    tunnel: w378 -> [w396]
                    tunnel: w377 -> [w395]
                    tunnel: [w394] -> w376
                    tunnel: w372 -> [w379]
                    i -> [w390]
                    n375 = local read "Ring 5"() -> (w387:bool)
                    n376 = local read "Load \nChannel"() -> (w389:dbl)
                    n377 = local read "Ring 1"() -> (w386:bool)
                    n378 = local read "Ring 2"() -> (w385:bool)
                    n379 = local read "Ring 3"() -> (w383:bool)
                    n380 = local read "Ring 4"() -> (w384:bool)
                    n381 = local read "Ring 6"() -> (w382:bool)
                    n382 = local read "Ring 8"() -> (w380:bool)
                    n383 = local read "Ring 7"() -> (w381:bool)
                    n384 = call "SequenceSelector_Load.vi"("Ring 8"=w380, "Ring 7"=w381, "Ring 6"=w382, "Ring 5"=w387, "Loop Iteration"=w379, "Inflow Channel Selector"=w389, "Ring 4"=w384, "Ring 3"=w383, "Ring 2"=w385, "Ring 1"=w386) -> ("Array"=w388:u8[][])
                    n385 = Index Array(array=w388, index (col)=w390) -> (element=w393:u8[])  [unwired: 1 in]
                    n386 = Byte Array To String(unsigned byte array=w393) -> (string=w391:string)
                    n387 = call "StorePreviousSwitchValues.vi"("Array"=w393) -> ()  [unwired: 3 in]
                    n388 = Enqueue Element(queue=w396, element=w391, error in (no error)=w395) -> (error out=w394:errorcluster)  [unwired: 1 in, 2 out]
                    n389 = Wait (ms)(milliseconds to wait=15) -> ()  [unwired: 1 out]
                  }
                  n390 = Add(x=1, y=w372) -> (x+y=w373:i32)
                  n391 = local write "Progress"(w373) -> ()
                }
              }
              frame #1 {
                w400 = u8[] [0, 0, 0, 0, 0, 11, 0, 16, 0, 0, 0, 2, 4, 255, 7, 31, 255]
                n392 = Byte Array To String(unsigned byte array=w400) -> (string=w399:string)
                n393 = call "StorePreviousSwitchValues.vi"("Array"=w400) -> ()  [unwired: 3 in]
                n394 = Enqueue Element(queue=w397, element=w399, error in (no error)=w398) -> ()  [unwired: 1 in, 3 out]
              }
              frame #2 {
                n395 = global read "CurrentSwitchValues_GlobalVariable.vi" "1"() -> (w430:bool)
                n396 = global read "CurrentSwitchValues_GlobalVariable.vi" "3"() -> (w423:bool)
                n397 = global read "CurrentSwitchValues_GlobalVariable.vi" "5"() -> (w425:bool)
                n398 = global read "CurrentSwitchValues_GlobalVariable.vi" "7"() -> (w427:bool)
                n399 = global read "CurrentSwitchValues_GlobalVariable.vi" "9"() -> (w415:bool)
                n400 = global read "CurrentSwitchValues_GlobalVariable.vi" "11"() -> (w417:bool)
                n401 = global read "CurrentSwitchValues_GlobalVariable.vi" "13"() -> (w419:bool)
                n402 = global read "CurrentSwitchValues_GlobalVariable.vi" "15"() -> (w421:bool)
                n403 = global read "CurrentSwitchValues_GlobalVariable.vi" "17"() -> (w407:bool)
                n404 = global read "CurrentSwitchValues_GlobalVariable.vi" "19"() -> (w409:bool)
                n405 = global read "CurrentSwitchValues_GlobalVariable.vi" "21"() -> (w411:bool)
                n406 = global read "CurrentSwitchValues_GlobalVariable.vi" "23"() -> (w413:bool)
                n407 = global read "CurrentSwitchValues_GlobalVariable.vi" "25"() -> (w406:bool)
                n408 = global read "CurrentSwitchValues_GlobalVariable.vi" "27"() -> (w404:bool)
                n409 = global read "CurrentSwitchValues_GlobalVariable.vi" "29"() -> (w402:bool)
                n410 = global read "CurrentSwitchValues_GlobalVariable.vi" "10"() -> (w416:bool)
                n411 = global read "CurrentSwitchValues_GlobalVariable.vi" "12"() -> (w418:bool)
                n412 = global read "CurrentSwitchValues_GlobalVariable.vi" "14"() -> (w420:bool)
                n413 = global read "CurrentSwitchValues_GlobalVariable.vi" "16"() -> (w422:bool)
                n414 = global read "CurrentSwitchValues_GlobalVariable.vi" "2"() -> (w429:bool)
                n415 = global read "CurrentSwitchValues_GlobalVariable.vi" "6"() -> (w426:bool)
                n416 = global read "CurrentSwitchValues_GlobalVariable.vi" "4"() -> (w424:bool)
                n417 = global read "CurrentSwitchValues_GlobalVariable.vi" "8"() -> (w428:bool)
                n418 = global read "CurrentSwitchValues_GlobalVariable.vi" "18"() -> (w408:bool)
                n419 = global read "CurrentSwitchValues_GlobalVariable.vi" "20"() -> (w410:bool)
                n420 = global read "CurrentSwitchValues_GlobalVariable.vi" "22"() -> (w412:bool)
                n421 = global read "CurrentSwitchValues_GlobalVariable.vi" "24"() -> (w414:bool)
                n422 = global read "CurrentSwitchValues_GlobalVariable.vi" "26"() -> (w405:bool)
                n423 = global read "CurrentSwitchValues_GlobalVariable.vi" "28"() -> (w403:bool)
                n424 = global read "CurrentSwitchValues_GlobalVariable.vi" "30"() -> (w401:bool)
                n425 = property on="1" class="Bool (strict)"("Value"=w430) -> ()  [unwired: 2 in, 2 out]
                n426 = property on="3" class="Bool (strict)"("Value"=w423) -> ()  [unwired: 2 in, 2 out]
                n427 = property on="5" class="Bool (strict)"("Value"=w425) -> ()  [unwired: 2 in, 2 out]
                n428 = property on="7" class="Bool (strict)"("Value"=w427) -> ()  [unwired: 2 in, 2 out]
                n429 = property on="9" class="Bool (strict)"("Value"=w415) -> ()  [unwired: 2 in, 2 out]
                n430 = property on="10" class="Bool (strict)"("Value"=w417) -> ()  [unwired: 2 in, 2 out]
                n431 = property on="13" class="Bool (strict)"("Value"=w419) -> ()  [unwired: 2 in, 2 out]
                n432 = property on="14" class="Bool (strict)"("Value"=w421) -> ()  [unwired: 2 in, 2 out]
                n433 = property on="17" class="Bool (strict)"("Value"=w407) -> ()  [unwired: 2 in, 2 out]
                n434 = property on="19" class="Bool (strict)"("Value"=w409) -> ()  [unwired: 2 in, 2 out]
                n435 = property on="21" class="Bool (strict)"("Value"=w411) -> ()  [unwired: 2 in, 2 out]
                n436 = property on="23" class="Bool (strict)"("Value"=w413) -> ()  [unwired: 2 in, 2 out]
                n437 = property on="25" class="Bool (strict)"("Value"=w406) -> ()  [unwired: 2 in, 2 out]
                n438 = property on="26" class="Bool (strict)"("Value"=w404) -> ()  [unwired: 2 in, 2 out]
                n439 = property on="29" class="Bool (strict)"("Value"=w402) -> ()  [unwired: 2 in, 2 out]
                n440 = property on="27" class="Bool (strict)"("Value"=w405) -> ()  [unwired: 2 in, 2 out]
                n441 = property on="28" class="Bool (strict)"("Value"=w403) -> ()  [unwired: 2 in, 2 out]
                n442 = property on="30" class="Bool (strict)"("Value"=w401) -> ()  [unwired: 2 in, 2 out]
                n443 = property on="2" class="Bool (strict)"("Value"=w429) -> ()  [unwired: 2 in, 2 out]
                n444 = property on="4" class="Bool (strict)"("Value"=w424) -> ()  [unwired: 2 in, 2 out]
                n445 = property on="6" class="Bool (strict)"("Value"=w426) -> ()  [unwired: 2 in, 2 out]
                n446 = property on="8" class="Bool (strict)"("Value"=w428) -> ()  [unwired: 2 in, 2 out]
                n447 = property on="11" class="Bool (strict)"("Value"=w416) -> ()  [unwired: 2 in, 2 out]
                n448 = property on="12" class="Bool (strict)"("Value"=w418) -> ()  [unwired: 2 in, 2 out]
                n449 = property on="15" class="Bool (strict)"("Value"=w420) -> ()  [unwired: 2 in, 2 out]
                n450 = property on="16" class="Bool (strict)"("Value"=w422) -> ()  [unwired: 2 in, 2 out]
                n451 = property on="18" class="Bool (strict)"("Value"=w408) -> ()  [unwired: 2 in, 2 out]
                n452 = property on="20" class="Bool (strict)"("Value"=w410) -> ()  [unwired: 2 in, 2 out]
                n453 = property on="22" class="Bool (strict)"("Value"=w412) -> ()  [unwired: 2 in, 2 out]
                n454 = property on="24" class="Bool (strict)"("Value"=w414) -> ()  [unwired: 2 in, 2 out]
              }
            }
          }
          event "Perform Initial Calibration": Mouse Down {
            n455 = event-data() -> ()  [unwired: 1 in, 8 out]
            n456 = global write "CurrentSwitchValues_GlobalVariable.vi" "Number of Inflow Steps Used During Calibration"("Number of Inflow Steps") -> ()
            n457 = while {
              i -> [w441]
              stop <- w439 continue-if-true
              w440 = 10
              n458 = local read "Running Calibration"() -> (w439:bool)
              n459 = Multiply(x=w441, y=w440) -> (x*y=w437:i32)
              n460 = Wait (ms)(milliseconds to wait=w440) -> ()  [unwired: 1 out]
              n461 = Divide(x=w437, y=60000) -> (x/y=→"Duration (min)":dbl)
            }
            n462 = stacked-sequence {
              tunnel: w435 -> [w443 w496 _ w555 w608 w673 w742 _ w796 _]
              tunnel: w434 -> [w444 w497 _ w556 w609 w672 w743 _ w797 _]
              tunnel: [w442 _ _ _ _ _ _ _ _ _] -> w433
              frame #0 {
                # "STEP 1:\n\nThis first step will flush the entire device (excluding\nthe reaction chambers) with the ELUTION BUFFER which will be used to provide the background intensity measurement.  \n\nThe flushing sequence is identical to that of the slow flush protocol. All chabers are closed during the flushing. The flushing steps can be found in the sub-vi: \"SEQ Selector FLUSH\".\n\nFor device flushing (excluding the reaction chambers) the fast flush protocol is administered (wait time between steps = 25ms)"
                n463 = stacked-sequence {
                  tunnel: w443 -> [w447 w462 _]
                  tunnel: w444 -> [w446 w463 _]
                  tunnel: [w445 _ _] -> w442
                  frame #0 {
                    n464 = for {
                      N: 200 -> [_]
                      tunnel: w447 -> [w451]
                      tunnel: w446 -> [w450]
                      tunnel: [w449] -> w445
                      n465 = for {
                        N: 6 -> [_]
                        tunnel: w451 -> [w456]
                        tunnel: w450 -> [w455]
                        tunnel: [w454] -> w449
                        i -> [w460]
                        n466 = local read "Elution Buffer Channel"() -> (w453:dbl)
                        n467 = call "SequenceSelector_Flush.vi"("Inflow Channel Selector"=w453) -> ("Array"=w459:u8[][])
                        n468 = Wait (ms)(milliseconds to wait=25) -> ()  [unwired: 1 out]
                        n469 = Index Array(array=w459, index (col)=w460) -> (element=w461:u8[])  [unwired: 1 in]
                        n470 = call "StorePreviousSwitchValues.vi"("Array"=w461) -> ()  [unwired: 3 in]
                        n471 = Byte Array To String(unsigned byte array=w461) -> (string=w457:string)
                        n472 = Enqueue Element(queue=w455, element=w457, error in (no error)=w456) -> (error out=w454:errorcluster)  [unwired: 1 in, 2 out]
                      }
                    }
                  }
                  frame #1 {
                    w465 = u8[] [0, 0, 0, 0, 0, 11, 0, 16, 0, 0, 0, 2, 4, 255, 7, 31, 255]
                    n473 = call "StorePreviousSwitchValues.vi"("Array"=w465) -> ()  [unwired: 3 in]
                    n474 = Byte Array To String(unsigned byte array=w465) -> (string=w464:string)
                    n475 = Enqueue Element(queue=w463, element=w464, error in (no error)=w462) -> ()  [unwired: 1 in, 3 out]
                  }
                  frame #2 {
                    n476 = global read "CurrentSwitchValues_GlobalVariable.vi" "1"() -> (w495:bool)
                    n477 = global read "CurrentSwitchValues_GlobalVariable.vi" "3"() -> (w488:bool)
                    n478 = global read "CurrentSwitchValues_GlobalVariable.vi" "5"() -> (w490:bool)
                    n479 = global read "CurrentSwitchValues_GlobalVariable.vi" "7"() -> (w492:bool)
                    n480 = global read "CurrentSwitchValues_GlobalVariable.vi" "9"() -> (w480:bool)
                    n481 = global read "CurrentSwitchValues_GlobalVariable.vi" "11"() -> (w482:bool)
                    n482 = global read "CurrentSwitchValues_GlobalVariable.vi" "13"() -> (w484:bool)
                    n483 = global read "CurrentSwitchValues_GlobalVariable.vi" "15"() -> (w486:bool)
                    n484 = global read "CurrentSwitchValues_GlobalVariable.vi" "17"() -> (w472:bool)
                    n485 = global read "CurrentSwitchValues_GlobalVariable.vi" "19"() -> (w474:bool)
                    n486 = global read "CurrentSwitchValues_GlobalVariable.vi" "21"() -> (w476:bool)
                    n487 = global read "CurrentSwitchValues_GlobalVariable.vi" "23"() -> (w478:bool)
                    n488 = global read "CurrentSwitchValues_GlobalVariable.vi" "25"() -> (w471:bool)
                    n489 = global read "CurrentSwitchValues_GlobalVariable.vi" "27"() -> (w469:bool)
                    n490 = global read "CurrentSwitchValues_GlobalVariable.vi" "29"() -> (w467:bool)
                    n491 = global read "CurrentSwitchValues_GlobalVariable.vi" "10"() -> (w481:bool)
                    n492 = global read "CurrentSwitchValues_GlobalVariable.vi" "12"() -> (w483:bool)
                    n493 = global read "CurrentSwitchValues_GlobalVariable.vi" "14"() -> (w485:bool)
                    n494 = global read "CurrentSwitchValues_GlobalVariable.vi" "16"() -> (w487:bool)
                    n495 = global read "CurrentSwitchValues_GlobalVariable.vi" "2"() -> (w494:bool)
                    n496 = global read "CurrentSwitchValues_GlobalVariable.vi" "6"() -> (w491:bool)
                    n497 = global read "CurrentSwitchValues_GlobalVariable.vi" "4"() -> (w489:bool)
                    n498 = global read "CurrentSwitchValues_GlobalVariable.vi" "8"() -> (w493:bool)
                    n499 = global read "CurrentSwitchValues_GlobalVariable.vi" "18"() -> (w473:bool)
                    n500 = global read "CurrentSwitchValues_GlobalVariable.vi" "20"() -> (w475:bool)
                    n501 = global read "CurrentSwitchValues_GlobalVariable.vi" "22"() -> (w477:bool)
                    n502 = global read "CurrentSwitchValues_GlobalVariable.vi" "24"() -> (w479:bool)
                    n503 = global read "CurrentSwitchValues_GlobalVariable.vi" "26"() -> (w470:bool)
                    n504 = global read "CurrentSwitchValues_GlobalVariable.vi" "28"() -> (w468:bool)
                    n505 = global read "CurrentSwitchValues_GlobalVariable.vi" "30"() -> (w466:bool)
                    n506 = property on="1" class="Bool (strict)"("Value"=w495) -> ()  [unwired: 2 in, 2 out]
                    n507 = property on="3" class="Bool (strict)"("Value"=w488) -> ()  [unwired: 2 in, 2 out]
                    n508 = property on="5" class="Bool (strict)"("Value"=w490) -> ()  [unwired: 2 in, 2 out]
                    n509 = property on="7" class="Bool (strict)"("Value"=w492) -> ()  [unwired: 2 in, 2 out]
                    n510 = property on="9" class="Bool (strict)"("Value"=w480) -> ()  [unwired: 2 in, 2 out]
                    n511 = property on="11" class="Bool (strict)"("Value"=w482) -> ()  [unwired: 2 in, 2 out]
                    n512 = property on="13" class="Bool (strict)"("Value"=w484) -> ()  [unwired: 2 in, 2 out]
                    n513 = property on="15" class="Bool (strict)"("Value"=w486) -> ()  [unwired: 2 in, 2 out]
                    n514 = property on="17" class="Bool (strict)"("Value"=w472) -> ()  [unwired: 2 in, 2 out]
                    n515 = property on="19" class="Bool (strict)"("Value"=w474) -> ()  [unwired: 2 in, 2 out]
                    n516 = property on="21" class="Bool (strict)"("Value"=w476) -> ()  [unwired: 2 in, 2 out]
                    n517 = property on="23" class="Bool (strict)"("Value"=w478) -> ()  [unwired: 2 in, 2 out]
                    n518 = property on="25" class="Bool (strict)"("Value"=w471) -> ()  [unwired: 2 in, 2 out]
                    n519 = property on="27" class="Bool (strict)"("Value"=w469) -> ()  [unwired: 2 in, 2 out]
                    n520 = property on="29" class="Bool (strict)"("Value"=w467) -> ()  [unwired: 2 in, 2 out]
                    n521 = property on="26" class="Bool (strict)"("Value"=w470) -> ()  [unwired: 2 in, 2 out]
                    n522 = property on="28" class="Bool (strict)"("Value"=w468) -> ()  [unwired: 2 in, 2 out]
                    n523 = property on="30" class="Bool (strict)"("Value"=w466) -> ()  [unwired: 2 in, 2 out]
                    n524 = property on="2" class="Bool (strict)"("Value"=w494) -> ()  [unwired: 2 in, 2 out]
                    n525 = property on="4" class="Bool (strict)"("Value"=w489) -> ()  [unwired: 2 in, 2 out]
                    n526 = property on="6" class="Bool (strict)"("Value"=w491) -> ()  [unwired: 2 in, 2 out]
                    n527 = property on="8" class="Bool (strict)"("Value"=w493) -> ()  [unwired: 2 in, 2 out]
                    n528 = property on="10" class="Bool (strict)"("Value"=w481) -> ()  [unwired: 2 in, 2 out]
                    n529 = property on="12" class="Bool (strict)"("Value"=w483) -> ()  [unwired: 2 in, 2 out]
                    n530 = property on="14" class="Bool (strict)"("Value"=w485) -> ()  [unwired: 2 in, 2 out]
                    n531 = property on="16" class="Bool (strict)"("Value"=w487) -> ()  [unwired: 2 in, 2 out]
                    n532 = property on="18" class="Bool (strict)"("Value"=w473) -> ()  [unwired: 2 in, 2 out]
                    n533 = property on="20" class="Bool (strict)"("Value"=w475) -> ()  [unwired: 2 in, 2 out]
                    n534 = property on="22" class="Bool (strict)"("Value"=w477) -> ()  [unwired: 2 in, 2 out]
                    n535 = property on="24" class="Bool (strict)"("Value"=w479) -> ()  [unwired: 2 in, 2 out]
                  }
                }
              }
              frame #1 {
                # "STEP 2: \n\nThe second step of this process is to completely fill each of the reaction chambers with the ELUTION BUFFER. This is achieved using a variation of the Load Full Process where the chamber selection has been omitted."
                n536 = stacked-sequence {
                  tunnel: w497 -> [w501 w517 _]
                  tunnel: w496 -> [w500 w518 _]
                  tunnel: [w499 _ _] -> _
                  frame #0 {
                    # "The number of cycle repeats is set to 300 to completly fill the chambers"
                    n537 = for {
                      N: 300 -> [_]
                      tunnel: w501 -> [w506]
                      tunnel: w500 -> [w505]
                      tunnel: [w504] -> w499
                      i -> [w502]
                      n538 = for {
                        N: 6 -> [_]
                        tunnel: w506 -> [w516]
                        tunnel: w505 -> [w515]
                        tunnel: [w514] -> w504
                        tunnel: w502 -> [w507]
                        i -> [w510]
                        n539 = local read "Elution Buffer Channel"() -> (w508:dbl)
                        n540 = call "SequenceSelector_LoadAllChambers.vi"("Inflow Channel Selector"=w508, "Loop Iteration"=w507) -> ("Array"=w509:u8[][])  [unwired: 7 in]
                        n541 = Index Array(array=w509, index (col)=w510) -> (element=w513:u8[])  [unwired: 1 in]
                        n542 = Byte Array To String(unsigned byte array=w513) -> (string=w511:string)
                        n543 = Enqueue Element(queue=w516, element=w511, error in (no error)=w515) -> (error out=w514:errorcluster)  [unwired: 1 in, 2 out]
                        n544 = call "StorePreviousSwitchValues.vi"("Array"=w513) -> ()  [unwired: 3 in]
                        n545 = Wait (ms)(milliseconds to wait=50) -> ()  [unwired: 1 out]
                      }
                    }
                  }
                  frame #1 {
                    w520 = u8[] [0, 0, 0, 0, 0, 11, 0, 16, 0, 0, 0, 2, 4, 255, 7, 31, 255]
                    n546 = Byte Array To String(unsigned byte array=w520) -> (string=w519:string)
                    n547 = call "StorePreviousSwitchValues.vi"("Array"=w520) -> ()  [unwired: 3 in]
                    n548 = Enqueue Element(queue=w517, element=w519, error in (no error)=w518) -> ()  [unwired: 1 in, 3 out]
                  }
                  frame #2 {
                    n549 = global read "CurrentSwitchValues_GlobalVariable.vi" "1"() -> (w550:bool)
                    n550 = global read "CurrentSwitchValues_GlobalVariable.vi" "3"() -> (w543:bool)
                    n551 = global read "CurrentSwitchValues_GlobalVariable.vi" "5"() -> (w545:bool)
                    n552 = global read "CurrentSwitchValues_GlobalVariable.vi" "7"() -> (w547:bool)
                    n553 = global read "CurrentSwitchValues_GlobalVariable.vi" "9"() -> (w535:bool)
                    n554 = global read "CurrentSwitchValues_GlobalVariable.vi" "11"() -> (w537:bool)
                    n555 = global read "CurrentSwitchValues_GlobalVariable.vi" "13"() -> (w539:bool)
                    n556 = global read "CurrentSwitchValues_GlobalVariable.vi" "15"() -> (w541:bool)
                    n557 = global read "CurrentSwitchValues_GlobalVariable.vi" "17"() -> (w527:bool)
                    n558 = global read "CurrentSwitchValues_GlobalVariable.vi" "19"() -> (w529:bool)
                    n559 = global read "CurrentSwitchValues_GlobalVariable.vi" "21"() -> (w531:bool)
                    n560 = global read "CurrentSwitchValues_GlobalVariable.vi" "23"() -> (w533:bool)
                    n561 = global read "CurrentSwitchValues_GlobalVariable.vi" "25"() -> (w526:bool)
                    n562 = global read "CurrentSwitchValues_GlobalVariable.vi" "27"() -> (w524:bool)
                    n563 = global read "CurrentSwitchValues_GlobalVariable.vi" "29"() -> (w522:bool)
                    n564 = global read "CurrentSwitchValues_GlobalVariable.vi" "10"() -> (w536:bool)
                    n565 = global read "CurrentSwitchValues_GlobalVariable.vi" "12"() -> (w538:bool)
                    n566 = global read "CurrentSwitchValues_GlobalVariable.vi" "14"() -> (w540:bool)
                    n567 = global read "CurrentSwitchValues_GlobalVariable.vi" "16"() -> (w542:bool)
                    n568 = global read "CurrentSwitchValues_GlobalVariable.vi" "2"() -> (w549:bool)
                    n569 = global read "CurrentSwitchValues_GlobalVariable.vi" "6"() -> (w546:bool)
                    n570 = global read "CurrentSwitchValues_GlobalVariable.vi" "4"() -> (w544:bool)
                    n571 = global read "CurrentSwitchValues_GlobalVariable.vi" "8"() -> (w548:bool)
                    n572 = global read "CurrentSwitchValues_GlobalVariable.vi" "18"() -> (w528:bool)
                    n573 = global read "CurrentSwitchValues_GlobalVariable.vi" "20"() -> (w530:bool)
                    n574 = global read "CurrentSwitchValues_GlobalVariable.vi" "22"() -> (w532:bool)
                    n575 = global read "CurrentSwitchValues_GlobalVariable.vi" "24"() -> (w534:bool)
                    n576 = global read "CurrentSwitchValues_GlobalVariable.vi" "26"() -> (w525:bool)
                    n577 = global read "CurrentSwitchValues_GlobalVariable.vi" "28"() -> (w523:bool)
                    n578 = global read "CurrentSwitchValues_GlobalVariable.vi" "30"() -> (w521:bool)
                    n579 = property on="3" class="Bool (strict)"("Value"=w543) -> ()  [unwired: 2 in, 2 out]
                    n580 = property on="5" class="Bool (strict)"("Value"=w545) -> ()  [unwired: 2 in, 2 out]
                    n581 = property on="7" class="Bool (strict)"("Value"=w547) -> ()  [unwired: 2 in, 2 out]
                    n582 = property on="9" class="Bool (strict)"("Value"=w535) -> ()  [unwired: 2 in, 2 out]
                    n583 = property on="11" class="Bool (strict)"("Value"=w537) -> ()  [unwired: 2 in, 2 out]
                    n584 = property on="13" class="Bool (strict)"("Value"=w539) -> ()  [unwired: 2 in, 2 out]
                    n585 = property on="15" class="Bool (strict)"("Value"=w541) -> ()  [unwired: 2 in, 2 out]
                    n586 = property on="17" class="Bool (strict)"("Value"=w527) -> ()  [unwired: 2 in, 2 out]
                    n587 = property on="19" class="Bool (strict)"("Value"=w529) -> ()  [unwired: 2 in, 2 out]
                    n588 = property on="21" class="Bool (strict)"("Value"=w531) -> ()  [unwired: 2 in, 2 out]
                    n589 = property on="23" class="Bool (strict)"("Value"=w533) -> ()  [unwired: 2 in, 2 out]
                    n590 = property on="25" class="Bool (strict)"("Value"=w526) -> ()  [unwired: 2 in, 2 out]
                    n591 = property on="27" class="Bool (strict)"("Value"=w524) -> ()  [unwired: 2 in, 2 out]
                    n592 = property on="29" class="Bool (strict)"("Value"=w522) -> ()  [unwired: 2 in, 2 out]
                    n593 = property on="1" class="Bool (strict)"("Value"=w550) -> ()  [unwired: 2 in, 2 out]
                    n594 = property on="26" class="Bool (strict)"("Value"=w525) -> ()  [unwired: 2 in, 2 out]
                    n595 = property on="28" class="Bool (strict)"("Value"=w523) -> ()  [unwired: 2 in, 2 out]
                    n596 = property on="30" class="Bool (strict)"("Value"=w521) -> ()  [unwired: 2 in, 2 out]
                    n597 = property on="2" class="Bool (strict)"("Value"=w549) -> ()  [unwired: 2 in, 2 out]
                    n598 = property on="4" class="Bool (strict)"("Value"=w544) -> ()  [unwired: 2 in, 2 out]
                    n599 = property on="6" class="Bool (strict)"("Value"=w546) -> ()  [unwired: 2 in, 2 out]
                    n600 = property on="8" class="Bool (strict)"("Value"=w548) -> ()  [unwired: 2 in, 2 out]
                    n601 = property on="10" class="Bool (strict)"("Value"=w536) -> ()  [unwired: 2 in, 2 out]
                    n602 = property on="12" class="Bool (strict)"("Value"=w538) -> ()  [unwired: 2 in, 2 out]
                    n603 = property on="14" class="Bool (strict)"("Value"=w540) -> ()  [unwired: 2 in, 2 out]
                    n604 = property on="16" class="Bool (strict)"("Value"=w542) -> ()  [unwired: 2 in, 2 out]
                    n605 = property on="18" class="Bool (strict)"("Value"=w528) -> ()  [unwired: 2 in, 2 out]
                    n606 = property on="20" class="Bool (strict)"("Value"=w530) -> ()  [unwired: 2 in, 2 out]
                    n607 = property on="22" class="Bool (strict)"("Value"=w532) -> ()  [unwired: 2 in, 2 out]
                    n608 = property on="24" class="Bool (strict)"("Value"=w534) -> ()  [unwired: 2 in, 2 out]
                  }
                }
              }
              frame #2 {
                # "STEP 3: \n\nBefore performing the dilution sequence, the current state of the reaction chambers - completely filled with the ELUTION BUFFER- should be imaged to acquire a background value for the intensity measurements. This is achieved via the calling upon an executable file."
                n609 = flat-sequence {
                  frame #0 {
                    n610 = call <vilib>:"System Exec.vi"("command line"="C:\\Users\\avdlinde\\Desktop\\Labview Interface for Jove Paper\\dummy_sender.exe") -> ()  [unwired: 7 in, 4 out]
                  }
                  frame #1 {
                    n611 = call <vilib>:"System Exec.vi"("wait until completion? (T)"=TRUE, "command line"="Replace with Reciever Excecutable") -> ()  [unwired: 6 in, 4 out]
                  }
                  frame #2 {
                    # "Waiting step will ensure that \nthe program does not record \ntwo sets of images at one time\npoint due errors regarding the \nsending of messages."
                    n612 = Wait (ms)(milliseconds to wait=30000) -> ()  [unwired: 1 out]
                  }
                }
              }
              frame #3 {
                # "STEP 4:\n\nThis third  step will flush the entire device (excluding the reaction chambers) with the fluorophore which will be used to calibrate the devices. \n\nThe flushing sequence is identical to that of the slow flush protocol. All chabers are closed during the flushing. The flushing steps can be found in the sub-vi: \"SEQ Selector FLUSH\".\n\nFor device flushing (excluding the reaction chambers) the fast flush protocol is administered (wait time between steps = 100ms)"
                n613 = stacked-sequence {
                  tunnel: w555 -> [w559 w574 _]
                  tunnel: w556 -> [w558 w575 _]
                  tunnel: [w557 _ _] -> _
                  frame #0 {
                    n614 = for {
                      N: 200 -> [_]
                      tunnel: w559 -> [w563]
                      tunnel: w558 -> [w562]
                      tunnel: [w561] -> w557
                      n615 = for {
                        N: 6 -> [_]
                        tunnel: w563 -> [w568]
                        tunnel: w562 -> [w567]
                        tunnel: [w566] -> w561
                        i -> [w572]
                        # "T-wait is 100 ms,\nfreq = +-1.7Hz if fast and T-wait is 556ms, freq = 0.3Hz if slow flush."
                        n616 = local read "Fluorophore Channel"() -> (w565:dbl)
                        n617 = call "SequenceSelector_Flush.vi"("Inflow Channel Selector"=w565) -> ("Array"=w571:u8[][])
                        n618 = Wait (ms)(milliseconds to wait=100) -> ()  [unwired: 1 out]
                        n619 = Index Array(array=w571, index (col)=w572) -> (element=w573:u8[])  [unwired: 1 in]
                        n620 = call "StorePreviousSwitchValues.vi"("Array"=w573) -> ()  [unwired: 3 in]
                        n621 = Byte Array To String(unsigned byte array=w573) -> (string=w569:string)
                        n622 = Enqueue Element(queue=w567, element=w569, error in (no error)=w568) -> (error out=w566:errorcluster)  [unwired: 1 in, 2 out]
                      }
                    }
                  }
                  frame #1 {
                    w577 = u8[] [0, 0, 0, 0, 0, 11, 0, 16, 0, 0, 0, 2, 4, 255, 7, 31, 255]
                    n623 = call "StorePreviousSwitchValues.vi"("Array"=w577) -> ()  [unwired: 3 in]
                    n624 = Byte Array To String(unsigned byte array=w577) -> (string=w576:string)
                    n625 = Enqueue Element(queue=w575, element=w576, error in (no error)=w574) -> ()  [unwired: 1 in, 3 out]
                  }
                  frame #2 {
                    n626 = global read "CurrentSwitchValues_GlobalVariable.vi" "1"() -> (w607:bool)
                    n627 = global read "CurrentSwitchValues_GlobalVariable.vi" "3"() -> (w600:bool)
                    n628 = global read "CurrentSwitchValues_GlobalVariable.vi" "5"() -> (w602:bool)
                    n629 = global read "CurrentSwitchValues_GlobalVariable.vi" "7"() -> (w604:bool)
                    n630 = global read "CurrentSwitchValues_GlobalVariable.vi" "9"() -> (w592:bool)
                    n631 = global read "CurrentSwitchValues_GlobalVariable.vi" "11"() -> (w594:bool)
                    n632 = global read "CurrentSwitchValues_GlobalVariable.vi" "13"() -> (w596:bool)
                    n633 = global read "CurrentSwitchValues_GlobalVariable.vi" "15"() -> (w598:bool)
                    n634 = global read "CurrentSwitchValues_GlobalVariable.vi" "17"() -> (w584:bool)
                    n635 = global read "CurrentSwitchValues_GlobalVariable.vi" "19"() -> (w586:bool)
                    n636 = global read "CurrentSwitchValues_GlobalVariable.vi" "21"() -> (w588:bool)
                    n637 = global read "CurrentSwitchValues_GlobalVariable.vi" "23"() -> (w590:bool)
                    n638 = global read "CurrentSwitchValues_GlobalVariable.vi" "25"() -> (w583:bool)
                    n639 = global read "CurrentSwitchValues_GlobalVariable.vi" "27"() -> (w581:bool)
                    n640 = global read "CurrentSwitchValues_GlobalVariable.vi" "29"() -> (w579:bool)
                    n641 = global read "CurrentSwitchValues_GlobalVariable.vi" "10"() -> (w593:bool)
                    n642 = global read "CurrentSwitchValues_GlobalVariable.vi" "12"() -> (w595:bool)
                    n643 = global read "CurrentSwitchValues_GlobalVariable.vi" "14"() -> (w597:bool)
                    n644 = global read "CurrentSwitchValues_GlobalVariable.vi" "16"() -> (w599:bool)
                    n645 = global read "CurrentSwitchValues_GlobalVariable.vi" "2"() -> (w606:bool)
                    n646 = global read "CurrentSwitchValues_GlobalVariable.vi" "6"() -> (w603:bool)
                    n647 = global read "CurrentSwitchValues_GlobalVariable.vi" "4"() -> (w601:bool)
                    n648 = global read "CurrentSwitchValues_GlobalVariable.vi" "8"() -> (w605:bool)
                    n649 = global read "CurrentSwitchValues_GlobalVariable.vi" "18"() -> (w585:bool)
                    n650 = global read "CurrentSwitchValues_GlobalVariable.vi" "20"() -> (w587:bool)
                    n651 = global read "CurrentSwitchValues_GlobalVariable.vi" "22"() -> (w589:bool)
                    n652 = global read "CurrentSwitchValues_GlobalVariable.vi" "24"() -> (w591:bool)
                    n653 = global read "CurrentSwitchValues_GlobalVariable.vi" "26"() -> (w582:bool)
                    n654 = global read "CurrentSwitchValues_GlobalVariable.vi" "28"() -> (w580:bool)
                    n655 = global read "CurrentSwitchValues_GlobalVariable.vi" "30"() -> (w578:bool)
                    n656 = property on="1" class="Bool (strict)"("Value"=w607) -> ()  [unwired: 2 in, 2 out]
                    n657 = property on="3" class="Bool (strict)"("Value"=w600) -> ()  [unwired: 2 in, 2 out]
                    n658 = property on="5" class="Bool (strict)"("Value"=w602) -> ()  [unwired: 2 in, 2 out]
                    n659 = property on="7" class="Bool (strict)"("Value"=w604) -> ()  [unwired: 2 in, 2 out]
                    n660 = property on="9" class="Bool (strict)"("Value"=w592) -> ()  [unwired: 2 in, 2 out]
                    n661 = property on="11" class="Bool (strict)"("Value"=w594) -> ()  [unwired: 2 in, 2 out]
                    n662 = property on="13" class="Bool (strict)"("Value"=w596) -> ()  [unwired: 2 in, 2 out]
                    n663 = property on="15" class="Bool (strict)"("Value"=w598) -> ()  [unwired: 2 in, 2 out]
                    n664 = property on="17" class="Bool (strict)"("Value"=w584) -> ()  [unwired: 2 in, 2 out]
                    n665 = property on="19" class="Bool (strict)"("Value"=w586) -> ()  [unwired: 2 in, 2 out]
                    n666 = property on="21" class="Bool (strict)"("Value"=w588) -> ()  [unwired: 2 in, 2 out]
                    n667 = property on="23" class="Bool (strict)"("Value"=w590) -> ()  [unwired: 2 in, 2 out]
                    n668 = property on="25" class="Bool (strict)"("Value"=w583) -> ()  [unwired: 2 in, 2 out]
                    n669 = property on="27" class="Bool (strict)"("Value"=w581) -> ()  [unwired: 2 in, 2 out]
                    n670 = property on="29" class="Bool (strict)"("Value"=w579) -> ()  [unwired: 2 in, 2 out]
                    n671 = property on="26" class="Bool (strict)"("Value"=w582) -> ()  [unwired: 2 in, 2 out]
                    n672 = property on="28" class="Bool (strict)"("Value"=w580) -> ()  [unwired: 2 in, 2 out]
                    n673 = property on="30" class="Bool (strict)"("Value"=w578) -> ()  [unwired: 2 in, 2 out]
                    n674 = property on="2" class="Bool (strict)"("Value"=w606) -> ()  [unwired: 2 in, 2 out]
                    n675 = property on="4" class="Bool (strict)"("Value"=w601) -> ()  [unwired: 2 in, 2 out]
                    n676 = property on="6" class="Bool (strict)"("Value"=w603) -> ()  [unwired: 2 in, 2 out]
                    n677 = property on="8" class="Bool (strict)"("Value"=w605) -> ()  [unwired: 2 in, 2 out]
                    n678 = property on="10" class="Bool (strict)"("Value"=w593) -> ()  [unwired: 2 in, 2 out]
                    n679 = property on="12" class="Bool (strict)"("Value"=w595) -> ()  [unwired: 2 in, 2 out]
                    n680 = property on="14" class="Bool (strict)"("Value"=w597) -> ()  [unwired: 2 in, 2 out]
                    n681 = property on="16" class="Bool (strict)"("Value"=w599) -> ()  [unwired: 2 in, 2 out]
                    n682 = property on="18" class="Bool (strict)"("Value"=w585) -> ()  [unwired: 2 in, 2 out]
                    n683 = property on="20" class="Bool (strict)"("Value"=w587) -> ()  [unwired: 2 in, 2 out]
                    n684 = property on="22" class="Bool (strict)"("Value"=w589) -> ()  [unwired: 2 in, 2 out]
                    n685 = property on="24" class="Bool (strict)"("Value"=w591) -> ()  [unwired: 2 in, 2 out]
                  }
                }
              }
              frame #4 {
                # "STEP 5: \n\nThe fourth step of this process is to completely fill each of the reaction chambers with the fluorophore solution. This is achieved using a variation of the Load Full Process where the chamber selection has been omitted."
                n686 = stacked-sequence {
                  tunnel: w609 -> [w613 w638 _]
                  tunnel: w608 -> [w612 w639 _]
                  tunnel: [w611 _ _] -> _
                  frame #0 {
                    n687 = for {
                      N: 8 -> [_]
                      tunnel: w613 -> [w620]
                      shift-right: [w618] -> w611
                      shift-left: w612 -> [w619]
                      i -> [w616]
                      n688 = Add(x=w616, y=1) -> (x+y=w614:i32)
                      n689 = global write "CurrentSwitchValues_GlobalVariable.vi" "Current Reactor"(w614) -> ()
                      n690 = for {
                        N: 150 -> [_]
                        tunnel: w620 -> [w625]
                        tunnel: w619 -> [w624]
                        tunnel: [w623] -> w618
                        i -> [w621]
                        n691 = for {
                          N: 6 -> [_]
                          tunnel: w625 -> [w637]
                          tunnel: w624 -> [w636]
                          tunnel: [w635] -> w623
                          tunnel: w621 -> [w627]
                          i -> [w631]
                          w628 = TRUE
                          n692 = local read "Fluorophore Channel"() -> (w630:dbl)
                          n693 = global read "CurrentSwitchValues_GlobalVariable.vi" "Current Reactor"() -> (w626:dbl)
                          n694 = call "SequenceSelector_LoadPerReactor.vi"("Reactor 6"=w628, "Reactor 7"=w628, "Reactor 8"=w628, "Loop Iteration"=w627, "Reactor 5"=w628, "Reactor 4"=w628, "Current Reactor"=w626, "Reactor 3"=w628, "Reactor 2"=w628, "Reactor 1"=w628, "Inflow Channel Selector"=w630) -> ("Array"=w629:u8[][])
                          n695 = Index Array(array=w629, index (col)=w631) -> (element=w634:u8[])  [unwired: 1 in]
                          n696 = Byte Array To String(unsigned byte array=w634) -> (string=w632:string)
                          n697 = Enqueue Element(queue=w637, element=w632, error in (no error)=w636) -> (error out=w635:errorcluster)  [unwired: 1 in, 2 out]
                          n698 = call "StorePreviousSwitchValues.vi"("Array"=w634) -> ()  [unwired: 3 in]
                          n699 = Wait (ms)(milliseconds to wait=50) -> ()  [unwired: 1 out]
                        }
                      }
                    }
                  }
                  frame #1 {
                    w641 = u8[] [0, 0, 0, 0, 0, 11, 0, 16, 0, 0, 0, 2, 4, 255, 7, 31, 255]
                    n700 = Byte Array To String(unsigned byte array=w641) -> (string=w640:string)
                    n701 = call "StorePreviousSwitchValues.vi"("Array"=w641) -> ()  [unwired: 3 in]
                    n702 = Enqueue Element(queue=w638, element=w640, error in (no error)=w639) -> ()  [unwired: 1 in, 3 out]
                  }
                  frame #2 {
                    n703 = global read "CurrentSwitchValues_GlobalVariable.vi" "1"() -> (w671:bool)
                    n704 = global read "CurrentSwitchValues_GlobalVariable.vi" "3"() -> (w664:bool)
                    n705 = global read "CurrentSwitchValues_GlobalVariable.vi" "5"() -> (w666:bool)
                    n706 = global read "CurrentSwitchValues_GlobalVariable.vi" "7"() -> (w668:bool)
                    n707 = global read "CurrentSwitchValues_GlobalVariable.vi" "9"() -> (w656:bool)
                    n708 = global read "CurrentSwitchValues_GlobalVariable.vi" "11"() -> (w658:bool)
                    n709 = global read "CurrentSwitchValues_GlobalVariable.vi" "13"() -> (w660:bool)
                    n710 = global read "CurrentSwitchValues_GlobalVariable.vi" "15"() -> (w662:bool)
                    n711 = global read "CurrentSwitchValues_GlobalVariable.vi" "17"() -> (w648:bool)
                    n712 = global read "CurrentSwitchValues_GlobalVariable.vi" "19"() -> (w650:bool)
                    n713 = global read "CurrentSwitchValues_GlobalVariable.vi" "21"() -> (w652:bool)
                    n714 = global read "CurrentSwitchValues_GlobalVariable.vi" "23"() -> (w654:bool)
                    n715 = global read "CurrentSwitchValues_GlobalVariable.vi" "25"() -> (w647:bool)
                    n716 = global read "CurrentSwitchValues_GlobalVariable.vi" "27"() -> (w645:bool)
                    n717 = global read "CurrentSwitchValues_GlobalVariable.vi" "29"() -> (w643:bool)
                    n718 = global read "CurrentSwitchValues_GlobalVariable.vi" "10"() -> (w657:bool)
                    n719 = global read "CurrentSwitchValues_GlobalVariable.vi" "12"() -> (w659:bool)
                    n720 = global read "CurrentSwitchValues_GlobalVariable.vi" "14"() -> (w661:bool)
                    n721 = global read "CurrentSwitchValues_GlobalVariable.vi" "16"() -> (w663:bool)
                    n722 = global read "CurrentSwitchValues_GlobalVariable.vi" "2"() -> (w670:bool)
                    n723 = global read "CurrentSwitchValues_GlobalVariable.vi" "6"() -> (w667:bool)
                    n724 = global read "CurrentSwitchValues_GlobalVariable.vi" "4"() -> (w665:bool)
                    n725 = global read "CurrentSwitchValues_GlobalVariable.vi" "8"() -> (w669:bool)
                    n726 = global read "CurrentSwitchValues_GlobalVariable.vi" "18"() -> (w649:bool)
                    n727 = global read "CurrentSwitchValues_GlobalVariable.vi" "20"() -> (w651:bool)
                    n728 = global read "CurrentSwitchValues_GlobalVariable.vi" "22"() -> (w653:bool)
                    n729 = global read "CurrentSwitchValues_GlobalVariable.vi" "24"() -> (w655:bool)
                    n730 = global read "CurrentSwitchValues_GlobalVariable.vi" "26"() -> (w646:bool)
                    n731 = global read "CurrentSwitchValues_GlobalVariable.vi" "28"() -> (w644:bool)
                    n732 = global read "CurrentSwitchValues_GlobalVariable.vi" "30"() -> (w642:bool)
                    n733 = property on="3" class="Bool (strict)"("Value"=w664) -> ()  [unwired: 2 in, 2 out]
                    n734 = property on="5" class="Bool (strict)"("Value"=w666) -> ()  [unwired: 2 in, 2 out]
                    n735 = property on="7" class="Bool (strict)"("Value"=w668) -> ()  [unwired: 2 in, 2 out]
                    n736 = property on="9" class="Bool (strict)"("Value"=w656) -> ()  [unwired: 2 in, 2 out]
                    n737 = property on="11" class="Bool (strict)"("Value"=w658) -> ()  [unwired: 2 in, 2 out]
                    n738 = property on="13" class="Bool (strict)"("Value"=w660) -> ()  [unwired: 2 in, 2 out]
                    n739 = property on="15" class="Bool (strict)"("Value"=w662) -> ()  [unwired: 2 in, 2 out]
                    n740 = property on="17" class="Bool (strict)"("Value"=w648) -> ()  [unwired: 2 in, 2 out]
                    n741 = property on="19" class="Bool (strict)"("Value"=w650) -> ()  [unwired: 2 in, 2 out]
                    n742 = property on="21" class="Bool (strict)"("Value"=w652) -> ()  [unwired: 2 in, 2 out]
                    n743 = property on="23" class="Bool (strict)"("Value"=w654) -> ()  [unwired: 2 in, 2 out]
                    n744 = property on="25" class="Bool (strict)"("Value"=w647) -> ()  [unwired: 2 in, 2 out]
                    n745 = property on="27" class="Bool (strict)"("Value"=w645) -> ()  [unwired: 2 in, 2 out]
                    n746 = property on="29" class="Bool (strict)"("Value"=w643) -> ()  [unwired: 2 in, 2 out]
                    n747 = property on="1" class="Bool (strict)"("Value"=w671) -> ()  [unwired: 2 in, 2 out]
                    n748 = property on="26" class="Bool (strict)"("Value"=w646) -> ()  [unwired: 2 in, 2 out]
                    n749 = property on="28" class="Bool (strict)"("Value"=w644) -> ()  [unwired: 2 in, 2 out]
                    n750 = property on="30" class="Bool (strict)"("Value"=w642) -> ()  [unwired: 2 in, 2 out]
                    n751 = property on="2" class="Bool (strict)"("Value"=w670) -> ()  [unwired: 2 in, 2 out]
                    n752 = property on="4" class="Bool (strict)"("Value"=w665) -> ()  [unwired: 2 in, 2 out]
                    n753 = property on="6" class="Bool (strict)"("Value"=w667) -> ()  [unwired: 2 in, 2 out]
                    n754 = property on="8" class="Bool (strict)"("Value"=w669) -> ()  [unwired: 2 in, 2 out]
                    n755 = property on="10" class="Bool (strict)"("Value"=w657) -> ()  [unwired: 2 in, 2 out]
                    n756 = property on="12" class="Bool (strict)"("Value"=w659) -> ()  [unwired: 2 in, 2 out]
                    n757 = property on="14" class="Bool (strict)"("Value"=w661) -> ()  [unwired: 2 in, 2 out]
                    n758 = property on="16" class="Bool (strict)"("Value"=w663) -> ()  [unwired: 2 in, 2 out]
                    n759 = property on="18" class="Bool (strict)"("Value"=w649) -> ()  [unwired: 2 in, 2 out]
                    n760 = property on="20" class="Bool (strict)"("Value"=w651) -> ()  [unwired: 2 in, 2 out]
                    n761 = property on="22" class="Bool (strict)"("Value"=w653) -> ()  [unwired: 2 in, 2 out]
                    n762 = property on="24" class="Bool (strict)"("Value"=w655) -> ()  [unwired: 2 in, 2 out]
                  }
                }
              }
              frame #5 {
                # "STEP 6:\n\nIn this step the reaction chambers are mixed to ensure that there is a homogeneous distribution of the fluorophores within the chambers."
                n763 = stacked-sequence {
                  tunnel: w673 -> [w677 w709 _]
                  tunnel: w672 -> [w676 w708 _]
                  tunnel: [w675 _ _] -> _
                  frame #0 {
                    n764 = local read "Number of Mixing Cycles"() -> (w674:dbl)
                    n765 = for {
                      N: w674 -> [_]
                      tunnel: w677 -> [w681]
                      tunnel: w676 -> [w680]
                      tunnel: [w679] -> w675
                      i -> [w686]
                      # "250"
                      n766 = local read "Number of Mixing Cycles"() -> (w678:dbl)
                      n767 = for {
                        N: 500 -> [_]
                        tunnel: w681 -> [w698]
                        tunnel: w680 -> [w697]
                        tunnel: [w696] -> w679
                        n768 = for {
                          N: 6 -> [_]
                          tunnel: w698 -> [w702]
                          tunnel: w697 -> [w701]
                          tunnel: [w700] -> w696
                          i -> [w705]
                          # "T-wait is 20 ms\nfreq = +-8.3Hz"
                          n769 = Wait (ms)(milliseconds to wait=20) -> ()  [unwired: 1 out]
                          n770 = Index Array(array=u8[][] [[0, 0, 0, 0, 0, 0, 0, 0, 2, 4, 3, 3, 3, 3], [0, 0, 0, 0, 0, 0, 0, 0, 0, 0, 0, 0, 0, 0], [0, 0, 0, 0, 0, 0, 0, 0, 0, 0, 0, 0, 0, 0], [0, 0, 0, 0, 0, 0, 0, 0, 0, 0, 0, 0, 0, 0], [0, 0, 0, 0, 0, 0, 0, 0, 0, 0, 0, 0, 0, 0], [11, 11, 11, 11, 11, 11, 11, 0, 0, 0, 0, 0, 0, 0], [0, 0, 0, 0, 0, 0, 0, 0, 0, 0, 0, 0, 0, 0], [16, 16, 16, 16, 16, 16, 16, 0, 0, 0, 0, 0, 0, 0], [0, 0, 0, 0, 0, 0, 0, 0, 0, 0, 0, 0, 0, 0], [0, 0, 0, 0, 0, 0, 0, 0, 0, 0, 0, 0, 0, 0], [0, 0, 0, 0, 0, 0, 0, 0, 0, 0, 0, 0, 0, 0], [2, 2, 2, 2, 2, 2, 2, 0, 0, 0, 0, 0, 0, 0], [4, 4, 4, 4, 4, 4, 4, 0, 0, 0, 0, 0, 0, 0], [255, 255, 255, 255, 255, 255, 0, 0, 0, 0, 0, 0, 0, 0], [3, 2, 6, 4, 5, 1, 0, 0, 0, 0, 0, 0, 0, 0], [27, 27, 27, 27, 27, 27, 0, 0, 0, 0, 0, 0, 0, 0], [255, 255, 255, 255, 255, 255, 0, 0, 0, 0, 0, 0, 0, 0]], index (col)=w705) -> (element=w706:u8[])  [unwired: 1 in]
                          n771 = Byte Array To String(unsigned byte array=w706) -> (string=w703:string)
                          n772 = call "StorePreviousSwitchValues.vi"("Array"=w706) -> ()  [unwired: 3 in]
                          n773 = Enqueue Element(queue=w701, element=w703, error in (no error)=w702) -> (error out=w700:errorcluster)  [unwired: 1 in, 2 out]
                        }
                      }
                      n774 = Add(x=1, y=w686) -> (x+y=w682:i32)
                      n775 = Less?(x=w682, y=w678) -> (x < y?=w683:bool)
                      n776 = case shown="True" w683 {
                        frame False {
                        }
                        frame True {
                          n777 = local read "Time between Mixing Cycles"() -> (w694:dbl)
                          n778 = Multiply(x=60000, y=w694) -> (x*y=w688:dbl)
                          n779 = Multiply(x=20, y=500) -> (x*y=w691:i32)
                          n780 = Multiply(x=w691, y=6) -> (x*y=w690:i32)
                          n781 = Add(x=w688, y=w690) -> (x+y=w687:dbl)
                          n782 = Wait (ms)(milliseconds to wait=w687) -> ()  [unwired: 1 out]
                        }
                      }
                    }
                  }
                  frame #1 {
                    w711 = u8[] [0, 0, 0, 0, 0, 11, 0, 16, 0, 0, 0, 2, 4, 255, 7, 31, 255]
                    n783 = call "StorePreviousSwitchValues.vi"("Array"=w711) -> ()  [unwired: 3 in]
                    n784 = Byte Array To String(unsigned byte array=w711) -> (string=w710:string)
                    n785 = Enqueue Element(queue=w708, element=w710, error in (no error)=w709) -> ()  [unwired: 1 in, 3 out]
                  }
                  frame #2 {
                    n786 = global read "CurrentSwitchValues_GlobalVariable.vi" "1"() -> (w741:bool)
                    n787 = global read "CurrentSwitchValues_GlobalVariable.vi" "3"() -> (w734:bool)
                    n788 = global read "CurrentSwitchValues_GlobalVariable.vi" "5"() -> (w736:bool)
                    n789 = global read "CurrentSwitchValues_GlobalVariable.vi" "7"() -> (w738:bool)
                    n790 = global read "CurrentSwitchValues_GlobalVariable.vi" "9"() -> (w726:bool)
                    n791 = global read "CurrentSwitchValues_GlobalVariable.vi" "11"() -> (w728:bool)
                    n792 = global read "CurrentSwitchValues_GlobalVariable.vi" "13"() -> (w730:bool)
                    n793 = global read "CurrentSwitchValues_GlobalVariable.vi" "15"() -> (w732:bool)
                    n794 = global read "CurrentSwitchValues_GlobalVariable.vi" "17"() -> (w718:bool)
                    n795 = global read "CurrentSwitchValues_GlobalVariable.vi" "19"() -> (w720:bool)
                    n796 = global read "CurrentSwitchValues_GlobalVariable.vi" "21"() -> (w722:bool)
                    n797 = global read "CurrentSwitchValues_GlobalVariable.vi" "23"() -> (w724:bool)
                    n798 = global read "CurrentSwitchValues_GlobalVariable.vi" "25"() -> (w717:bool)
                    n799 = global read "CurrentSwitchValues_GlobalVariable.vi" "27"() -> (w715:bool)
                    n800 = global read "CurrentSwitchValues_GlobalVariable.vi" "29"() -> (w713:bool)
                    n801 = global read "CurrentSwitchValues_GlobalVariable.vi" "10"() -> (w727:bool)
                    n802 = global read "CurrentSwitchValues_GlobalVariable.vi" "12"() -> (w729:bool)
                    n803 = global read "CurrentSwitchValues_GlobalVariable.vi" "14"() -> (w731:bool)
                    n804 = global read "CurrentSwitchValues_GlobalVariable.vi" "16"() -> (w733:bool)
                    n805 = global read "CurrentSwitchValues_GlobalVariable.vi" "2"() -> (w740:bool)
                    n806 = global read "CurrentSwitchValues_GlobalVariable.vi" "6"() -> (w737:bool)
                    n807 = global read "CurrentSwitchValues_GlobalVariable.vi" "4"() -> (w735:bool)
                    n808 = global read "CurrentSwitchValues_GlobalVariable.vi" "8"() -> (w739:bool)
                    n809 = global read "CurrentSwitchValues_GlobalVariable.vi" "18"() -> (w719:bool)
                    n810 = global read "CurrentSwitchValues_GlobalVariable.vi" "20"() -> (w721:bool)
                    n811 = global read "CurrentSwitchValues_GlobalVariable.vi" "22"() -> (w723:bool)
                    n812 = global read "CurrentSwitchValues_GlobalVariable.vi" "24"() -> (w725:bool)
                    n813 = global read "CurrentSwitchValues_GlobalVariable.vi" "26"() -> (w716:bool)
                    n814 = global read "CurrentSwitchValues_GlobalVariable.vi" "28"() -> (w714:bool)
                    n815 = global read "CurrentSwitchValues_GlobalVariable.vi" "30"() -> (w712:bool)
                    n816 = property on="1" class="Bool (strict)"("Value"=w741) -> ()  [unwired: 2 in, 2 out]
                    n817 = property on="3" class="Bool (strict)"("Value"=w734) -> ()  [unwired: 2 in, 2 out]
                    n818 = property on="5" class="Bool (strict)"("Value"=w736) -> ()  [unwired: 2 in, 2 out]
                    n819 = property on="7" class="Bool (strict)"("Value"=w738) -> ()  [unwired: 2 in, 2 out]
                    n820 = property on="9" class="Bool (strict)"("Value"=w726) -> ()  [unwired: 2 in, 2 out]
                    n821 = property on="11" class="Bool (strict)"("Value"=w728) -> ()  [unwired: 2 in, 2 out]
                    n822 = property on="13" class="Bool (strict)"("Value"=w730) -> ()  [unwired: 2 in, 2 out]
                    n823 = property on="15" class="Bool (strict)"("Value"=w732) -> ()  [unwired: 2 in, 2 out]
                    n824 = property on="17" class="Bool (strict)"("Value"=w718) -> ()  [unwired: 2 in, 2 out]
                    n825 = property on="19" class="Bool (strict)"("Value"=w720) -> ()  [unwired: 2 in, 2 out]
                    n826 = property on="21" class="Bool (strict)"("Value"=w722) -> ()  [unwired: 2 in, 2 out]
                    n827 = property on="23" class="Bool (strict)"("Value"=w724) -> ()  [unwired: 2 in, 2 out]
                    n828 = property on="25" class="Bool (strict)"("Value"=w717) -> ()  [unwired: 2 in, 2 out]
                    n829 = property on="27" class="Bool (strict)"("Value"=w715) -> ()  [unwired: 2 in, 2 out]
                    n830 = property on="29" class="Bool (strict)"("Value"=w713) -> ()  [unwired: 2 in, 2 out]
                    n831 = property on="26" class="Bool (strict)"("Value"=w716) -> ()  [unwired: 2 in, 2 out]
                    n832 = property on="28" class="Bool (strict)"("Value"=w714) -> ()  [unwired: 2 in, 2 out]
                    n833 = property on="30" class="Bool (strict)"("Value"=w712) -> ()  [unwired: 2 in, 2 out]
                    n834 = property on="2" class="Bool (strict)"("Value"=w740) -> ()  [unwired: 2 in, 2 out]
                    n835 = property on="4" class="Bool (strict)"("Value"=w735) -> ()  [unwired: 2 in, 2 out]
                    n836 = property on="6" class="Bool (strict)"("Value"=w737) -> ()  [unwired: 2 in, 2 out]
                    n837 = property on="8" class="Bool (strict)"("Value"=w739) -> ()  [unwired: 2 in, 2 out]
                    n838 = property on="10" class="Bool (strict)"("Value"=w727) -> ()  [unwired: 2 in, 2 out]
                    n839 = property on="12" class="Bool (strict)"("Value"=w729) -> ()  [unwired: 2 in, 2 out]
                    n840 = property on="14" class="Bool (strict)"("Value"=w731) -> ()  [unwired: 2 in, 2 out]
                    n841 = property on="16" class="Bool (strict)"("Value"=w733) -> ()  [unwired: 2 in, 2 out]
                    n842 = property on="18" class="Bool (strict)"("Value"=w719) -> ()  [unwired: 2 in, 2 out]
                    n843 = property on="20" class="Bool (strict)"("Value"=w721) -> ()  [unwired: 2 in, 2 out]
                    n844 = property on="22" class="Bool (strict)"("Value"=w723) -> ()  [unwired: 2 in, 2 out]
                    n845 = property on="24" class="Bool (strict)"("Value"=w725) -> ()  [unwired: 2 in, 2 out]
                  }
                }
              }
              frame #6 {
                # "STEP 7: \n\nDuring step 7 of the calibration process the entire device (excluding the reaction chambers) is flushed with the elution buffer which will be used to perform the dilutions in the following steps of the process."
                n846 = stacked-sequence {
                  tunnel: w742 -> [w745 w758 _]
                  tunnel: w743 -> [w744 w759 _]
                  frame #0 {
                    n847 = for {
                      N: 300 -> [_]
                      tunnel: w745 -> [w748]
                      tunnel: w744 -> [w747]
                      n848 = for {
                        N: 6 -> [_]
                        tunnel: w748 -> [w752]
                        tunnel: w747 -> [w751]
                        i -> [w756]
                        # "T-wait is 100 ms,\nfreq = +-1.7Hz if fast and T-wait is 556ms, freq = 0.3Hz if slow flush."
                        n849 = local read "Elution Buffer Channel"() -> (w750:dbl)
                        n850 = call "SequenceSelector_Flush.vi"("Inflow Channel Selector"=w750) -> ("Array"=w755:u8[][])
                        n851 = Wait (ms)(milliseconds to wait=100) -> ()  [unwired: 1 out]
                        n852 = Index Array(array=w755, index (col)=w756) -> (element=w757:u8[])  [unwired: 1 in]
                        n853 = call "StorePreviousSwitchValues.vi"("Array"=w757) -> ()  [unwired: 3 in]
                        n854 = Byte Array To String(unsigned byte array=w757) -> (string=w753:string)
                        n855 = Enqueue Element(queue=w751, element=w753, error in (no error)=w752) -> ()  [unwired: 1 in, 3 out]
                      }
                    }
                  }
                  frame #1 {
                    w761 = u8[] [0, 0, 0, 0, 0, 11, 0, 16, 0, 0, 0, 2, 4, 255, 7, 31, 255]
                    n856 = call "StorePreviousSwitchValues.vi"("Array"=w761) -> ()  [unwired: 3 in]
                    n857 = Byte Array To String(unsigned byte array=w761) -> (string=w760:string)
                    n858 = Enqueue Element(queue=w759, element=w760, error in (no error)=w758) -> ()  [unwired: 1 in, 3 out]
                  }
                  frame #2 {
                    n859 = global read "CurrentSwitchValues_GlobalVariable.vi" "1"() -> (w791:bool)
                    n860 = global read "CurrentSwitchValues_GlobalVariable.vi" "3"() -> (w784:bool)
                    n861 = global read "CurrentSwitchValues_GlobalVariable.vi" "5"() -> (w786:bool)
                    n862 = global read "CurrentSwitchValues_GlobalVariable.vi" "7"() -> (w788:bool)
                    n863 = global read "CurrentSwitchValues_GlobalVariable.vi" "9"() -> (w776:bool)
                    n864 = global read "CurrentSwitchValues_GlobalVariable.vi" "11"() -> (w778:bool)
                    n865 = global read "CurrentSwitchValues_GlobalVariable.vi" "13"() -> (w780:bool)
                    n866 = global read "CurrentSwitchValues_GlobalVariable.vi" "15"() -> (w782:bool)
                    n867 = global read "CurrentSwitchValues_GlobalVariable.vi" "17"() -> (w768:bool)
                    n868 = global read "CurrentSwitchValues_GlobalVariable.vi" "19"() -> (w770:bool)
                    n869 = global read "CurrentSwitchValues_GlobalVariable.vi" "21"() -> (w772:bool)
                    n870 = global read "CurrentSwitchValues_GlobalVariable.vi" "23"() -> (w774:bool)
                    n871 = global read "CurrentSwitchValues_GlobalVariable.vi" "25"() -> (w767:bool)
                    n872 = global read "CurrentSwitchValues_GlobalVariable.vi" "27"() -> (w765:bool)
                    n873 = global read "CurrentSwitchValues_GlobalVariable.vi" "29"() -> (w763:bool)
                    n874 = global read "CurrentSwitchValues_GlobalVariable.vi" "10"() -> (w777:bool)
                    n875 = global read "CurrentSwitchValues_GlobalVariable.vi" "12"() -> (w779:bool)
                    n876 = global read "CurrentSwitchValues_GlobalVariable.vi" "14"() -> (w781:bool)
                    n877 = global read "CurrentSwitchValues_GlobalVariable.vi" "16"() -> (w783:bool)
                    n878 = global read "CurrentSwitchValues_GlobalVariable.vi" "2"() -> (w790:bool)
                    n879 = global read "CurrentSwitchValues_GlobalVariable.vi" "6"() -> (w787:bool)
                    n880 = global read "CurrentSwitchValues_GlobalVariable.vi" "4"() -> (w785:bool)
                    n881 = global read "CurrentSwitchValues_GlobalVariable.vi" "8"() -> (w789:bool)
                    n882 = global read "CurrentSwitchValues_GlobalVariable.vi" "18"() -> (w769:bool)
                    n883 = global read "CurrentSwitchValues_GlobalVariable.vi" "20"() -> (w771:bool)
                    n884 = global read "CurrentSwitchValues_GlobalVariable.vi" "22"() -> (w773:bool)
                    n885 = global read "CurrentSwitchValues_GlobalVariable.vi" "24"() -> (w775:bool)
                    n886 = global read "CurrentSwitchValues_GlobalVariable.vi" "26"() -> (w766:bool)
                    n887 = global read "CurrentSwitchValues_GlobalVariable.vi" "28"() -> (w764:bool)
                    n888 = global read "CurrentSwitchValues_GlobalVariable.vi" "30"() -> (w762:bool)
                    n889 = property on="1" class="Bool (strict)"("Value"=w791) -> ()  [unwired: 2 in, 2 out]
                    n890 = property on="3" class="Bool (strict)"("Value"=w784) -> ()  [unwired: 2 in, 2 out]
                    n891 = property on="5" class="Bool (strict)"("Value"=w786) -> ()  [unwired: 2 in, 2 out]
                    n892 = property on="7" class="Bool (strict)"("Value"=w788) -> ()  [unwired: 2 in, 2 out]
                    n893 = property on="9" class="Bool (strict)"("Value"=w776) -> ()  [unwired: 2 in, 2 out]
                    n894 = property on="11" class="Bool (strict)"("Value"=w778) -> ()  [unwired: 2 in, 2 out]
                    n895 = property on="13" class="Bool (strict)"("Value"=w780) -> ()  [unwired: 2 in, 2 out]
                    n896 = property on="15" class="Bool (strict)"("Value"=w782) -> ()  [unwired: 2 in, 2 out]
                    n897 = property on="17" class="Bool (strict)"("Value"=w768) -> ()  [unwired: 2 in, 2 out]
                    n898 = property on="19" class="Bool (strict)"("Value"=w770) -> ()  [unwired: 2 in, 2 out]
                    n899 = property on="21" class="Bool (strict)"("Value"=w772) -> ()  [unwired: 2 in, 2 out]
                    n900 = property on="23" class="Bool (strict)"("Value"=w774) -> ()  [unwired: 2 in, 2 out]
                    n901 = property on="25" class="Bool (strict)"("Value"=w767) -> ()  [unwired: 2 in, 2 out]
                    n902 = property on="27" class="Bool (strict)"("Value"=w765) -> ()  [unwired: 2 in, 2 out]
                    n903 = property on="29" class="Bool (strict)"("Value"=w763) -> ()  [unwired: 2 in, 2 out]
                    n904 = property on="26" class="Bool (strict)"("Value"=w766) -> ()  [unwired: 2 in, 2 out]
                    n905 = property on="28" class="Bool (strict)"("Value"=w764) -> ()  [unwired: 2 in, 2 out]
                    n906 = property on="30" class="Bool (strict)"("Value"=w762) -> ()  [unwired: 2 in, 2 out]
                    n907 = property on="2" class="Bool (strict)"("Value"=w790) -> ()  [unwired: 2 in, 2 out]
                    n908 = property on="4" class="Bool (strict)"("Value"=w785) -> ()  [unwired: 2 in, 2 out]
                    n909 = property on="6" class="Bool (strict)"("Value"=w787) -> ()  [unwired: 2 in, 2 out]
                    n910 = property on="8" class="Bool (strict)"("Value"=w789) -> ()  [unwired: 2 in, 2 out]
                    n911 = property on="10" class="Bool (strict)"("Value"=w777) -> ()  [unwired: 2 in, 2 out]
                    n912 = property on="12" class="Bool (strict)"("Value"=w779) -> ()  [unwired: 2 in, 2 out]
                    n913 = property on="14" class="Bool (strict)"("Value"=w781) -> ()  [unwired: 2 in, 2 out]
                    n914 = property on="16" class="Bool (strict)"("Value"=w783) -> ()  [unwired: 2 in, 2 out]
                    n915 = property on="18" class="Bool (strict)"("Value"=w769) -> ()  [unwired: 2 in, 2 out]
                    n916 = property on="20" class="Bool (strict)"("Value"=w771) -> ()  [unwired: 2 in, 2 out]
                    n917 = property on="22" class="Bool (strict)"("Value"=w773) -> ()  [unwired: 2 in, 2 out]
                    n918 = property on="24" class="Bool (strict)"("Value"=w775) -> ()  [unwired: 2 in, 2 out]
                  }
                }
              }
              frame #7 {
                # "STEP 8: \n\nBefore performing the dilution sequence, the current state of the reaction chambers - completely filled with the fluorophore - should be imaged to acquire a baseline for the intensity measurements. This is achieved via the calling upon an executable file."
                n919 = flat-sequence {
                  frame #0 {
                    n920 = call <vilib>:"System Exec.vi"("command line"="C:\\Users\\avdlinde\\Desktop\\Labview Interface for Jove Paper\\dummy_sender.exe") -> ()  [unwired: 7 in, 4 out]
                  }
                  frame #1 {
                    n921 = call <vilib>:"System Exec.vi"("wait until completion? (T)"=TRUE, "command line"="Replace with reciever executable") -> ()  [unwired: 6 in, 4 out]
                  }
                  frame #2 {
                    # "Waiting step will ensure that \nthe program does not record \ntwo sets of images at one time\npoint due errors regarding the \nsending of messages."
                    n922 = Wait (ms)(milliseconds to wait=30000) -> ()  [unwired: 1 out]
                  }
                }
              }
              frame #8 {
                # "STEP 9: \n\nA loop is created within which the three main steps of the dilution process are performed:\n\n1 - Inject a volume of the dilutant (elution buffer) in to each of the reaction chambers. \n\n2 - Mix the reaction chambers to acquire a homogeneous solution within the chambers.\n\n3 -  Image the chambers by activating the imaging software of the microscope. \n\nThese three steps are found within the stacked sequence structure of the For-loop. The For-loop is executed n times with n being the Number of Dilution Steps chosen on the Virtual Interface."
                n923 = local read "Number of Dilution Steps"() -> (w798:dbl)
                n924 = for {
                  N: w798 -> [_]
                  tunnel: w797 -> [w800]
                  tunnel: w796 -> [w799]
                  n925 = stacked-sequence {
                    tunnel: w800 -> [w803 w826 w856 _ _]
                    tunnel: w799 -> [w802 w825 w855 _ _]
                    frame #0 {
                      # "STEP 9.1: \n\nDuring the first step of the dilution process the reaction chambers are partially filled with the dilutant (elution buffer)."
                      n926 = for {
                        N: 8 -> [_]
                        tunnel: w803 -> [w809]
                        tunnel: w802 -> [w808]
                        i -> [w806]
                        n927 = local read "Number of Inflow Steps"() -> (w807:dbl)
                        n928 = Add(x=w806, y=1) -> (x+y=w805:i32)
                        n929 = global write "CurrentSwitchValues_GlobalVariable.vi" "Current Reactor"(w805) -> ()
                        n930 = for {
                          N: w807 -> [_]
                          tunnel: w809 -> [w812]
                          tunnel: w808 -> [w811]
                          i -> [w810]
                          n931 = for {
                            N: 6 -> [_]
                            tunnel: w812 -> [w820]
                            tunnel: w811 -> [w819]
                            tunnel: w810 -> [w815]
                            i -> [w821]
                            w814 = TRUE
                            n932 = local read "Elution Buffer Channel"() -> (w817:dbl)
                            n933 = global read "CurrentSwitchValues_GlobalVariable.vi" "Current Reactor"() -> (w818:dbl)
                            n934 = call "SequenceSelector_LoadPerReactor.vi"("Reactor 6"=w814, "Reactor 7"=w814, "Reactor 8"=w814, "Loop Iteration"=w815, "Reactor 5"=w814, "Reactor 4"=w814, "Current Reactor"=w818, "Reactor 3"=w814, "Reactor 2"=w814, "Reactor 1"=w814, "Inflow Channel Selector"=w817) -> ("Array"=w816:u8[][])
                            n935 = Index Array(array=w816, index (col)=w821) -> (element=w824:u8[])  [unwired: 1 in]
                            n936 = Byte Array To String(unsigned byte array=w824) -> (string=w822:string)
                            n937 = Enqueue Element(queue=w820, element=w822, error in (no error)=w819) -> ()  [unwired: 1 in, 3 out]
                            n938 = call "StorePreviousSwitchValues.vi"("Array"=w824) -> ()  [unwired: 3 in]
                            n939 = Wait (ms)(milliseconds to wait=15) -> ()  [unwired: 1 out]
                          }
                        }
                      }
                    }
                    frame #1 {
                      # "STEP 9.2: \n\nFollowing the dilution, the solutions within the reaction chambers require mixing to ensure that there is a homogeneous distribution of fluorophores within the reaction chambers."
                      n940 = local read "Number of Mixing Cycles"() -> (w827:dbl)
                      n941 = for {
                        N: w827 -> [_]
                        tunnel: w826 -> [w829]
                        tunnel: w825 -> [w828]
                        i -> [w835]
                        # "250"
                        n942 = for {
                          N: 500 -> [_]
                          tunnel: w829 -> [w846]
                          tunnel: w828 -> [w845]
                          n943 = for {
                            N: 6 -> [_]
                            tunnel: w846 -> [w849]
                            tunnel: w845 -> [w848]
                            i -> [w852]
                            # "T-wait is 20 ms\nfreq = +-8.3Hz"
                            n944 = Wait (ms)(milliseconds to wait=20) -> ()  [unwired: 1 out]
                            n945 = Index Array(array=u8[][] [[0, 0, 0, 0, 0, 0, 0, 0, 2, 4, 3, 3, 3, 3], [0, 0, 0, 0, 0, 0, 0, 0, 0, 0, 0, 0, 0, 0], [0, 0, 0, 0, 0, 0, 0, 0, 0, 0, 0, 0, 0, 0], [0, 0, 0, 0, 0, 0, 0, 0, 0, 0, 0, 0, 0, 0], [0, 0, 0, 0, 0, 0, 0, 0, 0, 0, 0, 0, 0, 0], [11, 11, 11, 11, 11, 11, 11, 0, 0, 0, 0, 0, 0, 0], [0, 0, 0, 0, 0, 0, 0, 0, 0, 0, 0, 0, 0, 0], [16, 16, 16, 16, 16, 16, 16, 0, 0, 0, 0, 0, 0, 0], [0, 0, 0, 0, 0, 0, 0, 0, 0, 0, 0, 0, 0, 0], [0, 0, 0, 0, 0, 0, 0, 0, 0, 0, 0, 0, 0, 0], [0, 0, 0, 0, 0, 0, 0, 0, 0, 0, 0, 0, 0, 0], [2, 2, 2, 2, 2, 2, 2, 0, 0, 0, 0, 0, 0, 0], [4, 4, 4, 4, 4, 4, 4, 0, 0, 0, 0, 0, 0, 0], [255, 255, 255, 255, 255, 255, 0, 0, 0, 0, 0, 0, 0, 0], [3, 2, 6, 4, 5, 1, 0, 0, 0, 0, 0, 0, 0, 0], [27, 27, 27, 27, 27, 27, 0, 0, 0, 0, 0, 0, 0, 0], [255, 255, 255, 255, 255, 255, 0, 0, 0, 0, 0, 0, 0, 0]], index (col)=w852) -> (element=w853:u8[])  [unwired: 1 in]
                            n946 = Byte Array To String(unsigned byte array=w853) -> (string=w850:string)
                            n947 = call "StorePreviousSwitchValues.vi"("Array"=w853) -> ()  [unwired: 3 in]
                            n948 = Enqueue Element(queue=w849, element=w850, error in (no error)=w848) -> ()  [unwired: 1 in, 3 out]
                          }
                        }
                        n949 = local read "Number of Mixing Cycles"() -> (w830:dbl)
                        n950 = Add(x=1, y=w835) -> (x+y=w831:i32)
                        n951 = Less?(x=w831, y=w830) -> (x < y?=w832:bool)
                        n952 = case shown="True" w832 {
                          frame False {
                          }
                          frame True {
                            n953 = local read "Time between Mixing Cycles"() -> (w843:dbl)
                            n954 = Multiply(x=60000, y=w843) -> (x*y=w837:dbl)
                            n955 = Multiply(x=20, y=500) -> (x*y=w840:i32)
                            n956 = Multiply(x=w840, y=6) -> (x*y=w839:i32)
                            n957 = Add(x=w837, y=w839) -> (x+y=w836:dbl)
                            n958 = Wait (ms)(milliseconds to wait=w836) -> ()  [unwired: 1 out]
                          }
                        }
                      }
                    }
                    frame #2 {
                      w858 = u8[] [0, 0, 0, 0, 0, 11, 0, 16, 0, 0, 0, 2, 4, 255, 7, 31, 255]
                      # "STEP 9.2.1: \n\nEnsure that the reaction chambers are sealed and all flow is halted. Store the current states of the pneumatic valves such that these values can be represented on the Virtual Interface."
                      n959 = Byte Array To String(unsigned byte array=w858) -> (string=w857:string)
                      n960 = call "StorePreviousSwitchValues.vi"("Array"=w858) -> ()  [unwired: 3 in]
                      n961 = Enqueue Element(queue=w856, element=w857, error in (no error)=w855) -> ()  [unwired: 1 in, 3 out]
                    }
                    frame #3 {
                      # "STEP 9.2.2: \n\nSave the current switch states to the global variables."
                      n962 = global read "CurrentSwitchValues_GlobalVariable.vi" "1"() -> (w888:bool)
                      n963 = global read "CurrentSwitchValues_GlobalVariable.vi" "3"() -> (w881:bool)
                      n964 = global read "CurrentSwitchValues_GlobalVariable.vi" "5"() -> (w883:bool)
                      n965 = global read "CurrentSwitchValues_GlobalVariable.vi" "7"() -> (w885:bool)
                      n966 = global read "CurrentSwitchValues_GlobalVariable.vi" "9"() -> (w873:bool)
                      n967 = global read "CurrentSwitchValues_GlobalVariable.vi" "11"() -> (w875:bool)
                      n968 = global read "CurrentSwitchValues_GlobalVariable.vi" "13"() -> (w877:bool)
                      n969 = global read "CurrentSwitchValues_GlobalVariable.vi" "15"() -> (w879:bool)
                      n970 = global read "CurrentSwitchValues_GlobalVariable.vi" "17"() -> (w865:bool)
                      n971 = global read "CurrentSwitchValues_GlobalVariable.vi" "19"() -> (w867:bool)
                      n972 = global read "CurrentSwitchValues_GlobalVariable.vi" "21"() -> (w869:bool)
                      n973 = global read "CurrentSwitchValues_GlobalVariable.vi" "23"() -> (w871:bool)
                      n974 = global read "CurrentSwitchValues_GlobalVariable.vi" "25"() -> (w864:bool)
                      n975 = global read "CurrentSwitchValues_GlobalVariable.vi" "27"() -> (w862:bool)
                      n976 = global read "CurrentSwitchValues_GlobalVariable.vi" "29"() -> (w860:bool)
                      n977 = global read "CurrentSwitchValues_GlobalVariable.vi" "10"() -> (w874:bool)
                      n978 = global read "CurrentSwitchValues_GlobalVariable.vi" "12"() -> (w876:bool)
                      n979 = global read "CurrentSwitchValues_GlobalVariable.vi" "14"() -> (w878:bool)
                      n980 = global read "CurrentSwitchValues_GlobalVariable.vi" "16"() -> (w880:bool)
                      n981 = global read "CurrentSwitchValues_GlobalVariable.vi" "2"() -> (w887:bool)
                      n982 = global read "CurrentSwitchValues_GlobalVariable.vi" "6"() -> (w884:bool)
                      n983 = global read "CurrentSwitchValues_GlobalVariable.vi" "4"() -> (w882:bool)
                      n984 = global read "CurrentSwitchValues_GlobalVariable.vi" "8"() -> (w886:bool)
                      n985 = global read "CurrentSwitchValues_GlobalVariable.vi" "18"() -> (w866:bool)
                      n986 = global read "CurrentSwitchValues_GlobalVariable.vi" "20"() -> (w868:bool)
                      n987 = global read "CurrentSwitchValues_GlobalVariable.vi" "22"() -> (w870:bool)
                      n988 = global read "CurrentSwitchValues_GlobalVariable.vi" "24"() -> (w872:bool)
                      n989 = global read "CurrentSwitchValues_GlobalVariable.vi" "26"() -> (w863:bool)
                      n990 = global read "CurrentSwitchValues_GlobalVariable.vi" "28"() -> (w861:bool)
                      n991 = global read "CurrentSwitchValues_GlobalVariable.vi" "30"() -> (w859:bool)
                      n992 = property on="3" class="Bool (strict)"("Value"=w881) -> ()  [unwired: 2 in, 2 out]
                      n993 = property on="5" class="Bool (strict)"("Value"=w883) -> ()  [unwired: 2 in, 2 out]
                      n994 = property on="7" class="Bool (strict)"("Value"=w885) -> ()  [unwired: 2 in, 2 out]
                      n995 = property on="9" class="Bool (strict)"("Value"=w873) -> ()  [unwired: 2 in, 2 out]
                      n996 = property on="11" class="Bool (strict)"("Value"=w875) -> ()  [unwired: 2 in, 2 out]
                      n997 = property on="13" class="Bool (strict)"("Value"=w877) -> ()  [unwired: 2 in, 2 out]
                      n998 = property on="15" class="Bool (strict)"("Value"=w879) -> ()  [unwired: 2 in, 2 out]
                      n999 = property on="17" class="Bool (strict)"("Value"=w865) -> ()  [unwired: 2 in, 2 out]
                      n1000 = property on="19" class="Bool (strict)"("Value"=w867) -> ()  [unwired: 2 in, 2 out]
                      n1001 = property on="21" class="Bool (strict)"("Value"=w869) -> ()  [unwired: 2 in, 2 out]
                      n1002 = property on="23" class="Bool (strict)"("Value"=w871) -> ()  [unwired: 2 in, 2 out]
                      n1003 = property on="25" class="Bool (strict)"("Value"=w864) -> ()  [unwired: 2 in, 2 out]
                      n1004 = property on="27" class="Bool (strict)"("Value"=w862) -> ()  [unwired: 2 in, 2 out]
                      n1005 = property on="29" class="Bool (strict)"("Value"=w860) -> ()  [unwired: 2 in, 2 out]
                      n1006 = property on="1" class="Bool (strict)"("Value"=w888) -> ()  [unwired: 2 in, 2 out]
                      n1007 = property on="26" class="Bool (strict)"("Value"=w863) -> ()  [unwired: 2 in, 2 out]
                      n1008 = property on="28" class="Bool (strict)"("Value"=w861) -> ()  [unwired: 2 in, 2 out]
                      n1009 = property on="30" class="Bool (strict)"("Value"=w859) -> ()  [unwired: 2 in, 2 out]
                      n1010 = property on="2" class="Bool (strict)"("Value"=w887) -> ()  [unwired: 2 in, 2 out]
                      n1011 = property on="4" class="Bool (strict)"("Value"=w882) -> ()  [unwired: 2 in, 2 out]
                      n1012 = property on="6" class="Bool (strict)"("Value"=w884) -> ()  [unwired: 2 in, 2 out]
                      n1013 = property on="8" class="Bool (strict)"("Value"=w886) -> ()  [unwired: 2 in, 2 out]
                      n1014 = property on="10" class="Bool (strict)"("Value"=w874) -> ()  [unwired: 2 in, 2 out]
                      n1015 = property on="12" class="Bool (strict)"("Value"=w876) -> ()  [unwired: 2 in, 2 out]
                      n1016 = property on="14" class="Bool (strict)"("Value"=w878) -> ()  [unwired: 2 in, 2 out]
                      n1017 = property on="16" class="Bool (strict)"("Value"=w880) -> ()  [unwired: 2 in, 2 out]
                      n1018 = property on="18" class="Bool (strict)"("Value"=w866) -> ()  [unwired: 2 in, 2 out]
                      n1019 = property on="20" class="Bool (strict)"("Value"=w868) -> ()  [unwired: 2 in, 2 out]
                      n1020 = property on="22" class="Bool (strict)"("Value"=w870) -> ()  [unwired: 2 in, 2 out]
                      n1021 = property on="24" class="Bool (strict)"("Value"=w872) -> ()  [unwired: 2 in, 2 out]
                    }
                    frame #4 {
                      # "STEP 9.3: \n\nThe final step is to ensure that images are recorded of the reaction chambers. These images measure the fluorescence intensity of a small portion of the reaction chambers (with the \nsolution within the chambers being homogeneous) such that the volume of dilutant injected into the reaction chamber can be calculated.\n\nThe recording of the images is performed by calling a executable file which activates the NIS-elements software, triggering an automated program which captures the images. Upon \nreceiving a completion signal, the entire dilution process is repeated until the number of desired dilution steps (Number of Dilution Steps) is reached."
                      n1022 = flat-sequence {
                        frame #0 {
                          n1023 = call <vilib>:"System Exec.vi"("command line"="C:\\Users\\avdlinde\\Desktop\\Labview Interface for Jove Paper\\dummy_sender.exe") -> ()  [unwired: 7 in, 4 out]
                        }
                        frame #1 {
                          n1024 = call <vilib>:"System Exec.vi"("wait until completion? (T)"=TRUE, "command line"="Replace with reciever executable") -> ()  [unwired: 6 in, 4 out]
                        }
                        frame #2 {
                          # "Waiting step will ensure that \nthe program does not record \ntwo sets of images at one time\npoint due errors regarding the \nsending of messages."
                          n1025 = Wait (ms)(milliseconds to wait=30000) -> ()  [unwired: 1 out]
                        }
                      }
                    }
                  }
                }
              }
              frame #9 {
                # "STEP10: \n\nAfter each of the dilution steps has been performed, the microscope should be instructed to stop waiting for another command. \nThe refresh ratios are detmined via the Matlab Script. The determined values are subsequently stored as global variables for access throughout the Labview VI."
                n1026 = flat-sequence {
                  frame #0 {
                    # "Let the Microscope know that the sequence has ended and\nstop waiting for new commands."
                    n1027 = local write "Running Calibration"(FALSE) -> ()
                    n1028 = call <vilib>:"System Exec.vi"("command line"="C:\\Users\\avdlinde\\Desktop\\Labview Interface for Jove Paper\\dummy_stopper.exe") -> ()  [unwired: 7 in, 4 out]
                  }
                  frame #1 {
                    # "Run the Matlab calibration script."
                    n1029 = script code="%% The aim of this script is to perform the calibration of the labview\n%  software with regards to the dilution volume as efficiently as possible\n%  requiring minimal input from the user. \n\n%% Set paths for Scripts and Functions\naddpath C:\\Users\\Nikon\\Documents\\MATLAB\\bfmatlab\naddpath C:\\Users\\Nikon\\Desktop\\Matlab_Calibration_Script\\20170421_CalibrationScript_V2\n\n\n%% Selecting the correct .ND2 file:\n[fileName,pathName,filterIndex] = uigetfile('.nd2');\nnd2 = bfopen(char(join({pathName,fileName},'')));\n\n%% Provide the Initial Concentration of Fluorophore\ncellConcentration = inputdlg({'Input Initial Fluorophore Concentration:'});\ninitialConcentration = str2double(cellConcentration{1,1});\n\n%% Set the intensity range with which to view all images during ROI selection\ndesiredIntensity = selectIntensity(nd2{1,1}{2,1});\nintensityRange = [0, desiredIntensity];\n\n%% ROI selection for all chambers\n[xCoordinates, yCoordinates] = regionOfInterestDetermination(nd2, intensityRange);\n\n%% Determine the intensities of the ROI within all images\nintensities = intensityDetermination(nd2, xCoordinates, yCoordinates);\n\n%% Plot the intensity curves and view the refresh ratio\n[finalRefreshRatio, refreshPerRing] = plotIntensityCurvesCorrect(intensities, initialConcentration);\n\n\nRR1 = refreshPerRing(1,1);\nRR2 = refreshPerRing(2,1);\nRR3 = refreshPerRing(3,1);\nRR4 = refreshPerRing(4,1);\nRR5 = refreshPerRing(5,1);\nRR6 = refreshPerRing(6,1);\nRR7 = refreshPerRing(7,1);\nRR8 = refreshPerRing(8,1);\n\n%% This is the end of the script."() -> ("finalRefreshRatio"=w921:dbl, "RR1"=w911:dbl, "RR2"=w910:dbl, "RR3"=w909:dbl, "RR4"=w908:dbl, "RR5"=w907:dbl, "RR6"=w906:dbl, "RR7"=w905:dbl, "RR8"=w904:dbl)  [unwired: 1 in, 1 out]
                    "Refresh Ratio" <- w921
                    "Chamber 1" <- w911
                    "Chamber 2" <- w910
                    "Chamber 3" <- w909
                    "Chamber 4" <- w908
                    "Chamber 5" <- w907
                    "Chamber 6" <- w906
                    "Chamber 7" <- w905
                    "Chamber 8" <- w904
                    n1030 = global write "CurrentSwitchValues_GlobalVariable.vi" "Refresh Ratio Average"(w921) -> ()
                    n1031 = global write "CurrentSwitchValues_GlobalVariable.vi" "Refresh Ratio Reactor 8"(w904) -> ()
                    n1032 = global write "CurrentSwitchValues_GlobalVariable.vi" "Refresh Ratio Reactor 1"(w911) -> ()
                    n1033 = global write "CurrentSwitchValues_GlobalVariable.vi" "Refresh Ratio Reactor 2"(w910) -> ()
                    n1034 = global write "CurrentSwitchValues_GlobalVariable.vi" "Refresh Ratio Reactor 3"(w909) -> ()
                    n1035 = global write "CurrentSwitchValues_GlobalVariable.vi" "Refresh Ratio Reactor 4"(w908) -> ()
                    n1036 = global write "CurrentSwitchValues_GlobalVariable.vi" "Refresh Ratio Reactor 5"(w907) -> ()
                    n1037 = global write "CurrentSwitchValues_GlobalVariable.vi" "Refresh Ratio Reactor 6"(w906) -> ()
                    n1038 = global write "CurrentSwitchValues_GlobalVariable.vi" "Refresh Ratio Reactor 7"(w905) -> ()
                    n1039 = Initialize Array(w911, 8) -> (w903:dbl[])
                    n1040 = Replace Array Subset(array=w903, new element=w911, index=0) -> (w902:dbl[])
                    n1041 = Replace Array Subset(array=w902, new element=w910, index=1) -> (w901:dbl[])
                    n1042 = Replace Array Subset(array=w901, new element=w909, index=2) -> (w900:dbl[])
                    n1043 = Replace Array Subset(array=w900, new element=w908, index=3) -> (w899:dbl[])
                    n1044 = Replace Array Subset(array=w899, new element=w907, index=4) -> (w898:dbl[])
                    n1045 = Replace Array Subset(array=w898, new element=w906, index=5) -> (w897:dbl[])
                    n1046 = Replace Array Subset(array=w897, new element=w905, index=6) -> (w896:dbl[])
                    n1047 = Replace Array Subset(array=w896, new element=w904, index=7) -> (w895:dbl[])
                    n1048 = global write "CurrentSwitchValues_GlobalVariable.vi" "Reactor RR Array"(w895) -> ()
                  }
                }
              }
            }
            "Running Calibration" <- TRUE
          }
          event "Perform \nExperiments": Mouse Down {
            n1049 = event-data() -> ()  [unwired: 1 in, 8 out]
            n1050 = Get Date/Time In Seconds() -> (seconds since 1Jan1904=w926:timestamp)
            n1051 = property on="Time Stamp" class="AbsTime (strict)"("Value"=w926) -> ()  [unwired: 2 in, 2 out]
            n1052 = stacked-sequence {
              tunnel: w924 -> [w929 w981 w1038 w1091 w1148 w1200 w1267 w1338 w1959 w2011 w2067 w2138 _]
              tunnel: w923 -> [w928 w982 w1037 w1092 w1147 w1201 w1268 w1337 w1958 w2012 w2068 w2137 _]
              tunnel: [w927 _ _ _ _ _ _ _ _ _ _ _ _] -> w922
              frame #0 {
                # "Step 1:\nThe primary step in this simple expression\nprotocol is to flush the device with elution \nbuffer to ensure the removal of any residual\nsolutes from the calibration protocol."
                n1053 = stacked-sequence {
                  tunnel: w929 -> [w932 w947 _]
                  tunnel: w928 -> [w931 w948 _]
                  tunnel: [w930 _ _] -> w927
                  frame #0 {
                    n1054 = for {
                      N: 200 -> [_]
                      tunnel: w932 -> [w936]
                      tunnel: w931 -> [w935]
                      tunnel: [w934] -> w930
                      n1055 = for {
                        N: 6 -> [_]
                        tunnel: w936 -> [w941]
                        tunnel: w935 -> [w940]
                        tunnel: [w939] -> w934
                        i -> [w945]
                        n1056 = local read "Elution Buffer"() -> (w938:dbl)
                        n1057 = call "SequenceSelector_Flush.vi"("Inflow Channel Selector"=w938) -> ("Array"=w944:u8[][])
                        n1058 = Wait (ms)(milliseconds to wait=25) -> ()  [unwired: 1 out]
                        n1059 = Index Array(array=w944, index (col)=w945) -> (element=w946:u8[])  [unwired: 1 in]
                        n1060 = call "StorePreviousSwitchValues.vi"("Array"=w946) -> ()  [unwired: 3 in]
                        n1061 = Byte Array To String(unsigned byte array=w946) -> (string=w942:string)
                        n1062 = Enqueue Element(queue=w940, element=w942, error in (no error)=w941) -> (error out=w939:errorcluster)  [unwired: 1 in, 2 out]
                      }
                    }
                  }
                  frame #1 {
                    w950 = u8[] [0, 0, 0, 0, 0, 11, 0, 16, 0, 0, 0, 2, 4, 255, 7, 31, 255]
                    n1063 = call "StorePreviousSwitchValues.vi"("Array"=w950) -> ()  [unwired: 3 in]
                    n1064 = Byte Array To String(unsigned byte array=w950) -> (string=w949:string)
                    n1065 = Enqueue Element(queue=w948, element=w949, error in (no error)=w947) -> ()  [unwired: 1 in, 3 out]
                  }
                  frame #2 {
                    n1066 = global read "CurrentSwitchValues_GlobalVariable.vi" "1"() -> (w980:bool)
                    n1067 = global read "CurrentSwitchValues_GlobalVariable.vi" "3"() -> (w973:bool)
                    n1068 = global read "CurrentSwitchValues_GlobalVariable.vi" "5"() -> (w975:bool)
                    n1069 = global read "CurrentSwitchValues_GlobalVariable.vi" "7"() -> (w977:bool)
                    n1070 = global read "CurrentSwitchValues_GlobalVariable.vi" "9"() -> (w965:bool)
                    n1071 = global read "CurrentSwitchValues_GlobalVariable.vi" "11"() -> (w967:bool)
                    n1072 = global read "CurrentSwitchValues_GlobalVariable.vi" "13"() -> (w969:bool)
                    n1073 = global read "CurrentSwitchValues_GlobalVariable.vi" "15"() -> (w971:bool)
                    n1074 = global read "CurrentSwitchValues_GlobalVariable.vi" "17"() -> (w957:bool)
                    n1075 = global read "CurrentSwitchValues_GlobalVariable.vi" "19"() -> (w959:bool)
                    n1076 = global read "CurrentSwitchValues_GlobalVariable.vi" "21"() -> (w961:bool)
                    n1077 = global read "CurrentSwitchValues_GlobalVariable.vi" "23"() -> (w963:bool)
                    n1078 = global read "CurrentSwitchValues_GlobalVariable.vi" "25"() -> (w956:bool)
                    n1079 = global read "CurrentSwitchValues_GlobalVariable.vi" "27"() -> (w954:bool)
                    n1080 = global read "CurrentSwitchValues_GlobalVariable.vi" "29"() -> (w952:bool)
                    n1081 = global read "CurrentSwitchValues_GlobalVariable.vi" "10"() -> (w966:bool)
                    n1082 = global read "CurrentSwitchValues_GlobalVariable.vi" "12"() -> (w968:bool)
                    n1083 = global read "CurrentSwitchValues_GlobalVariable.vi" "14"() -> (w970:bool)
                    n1084 = global read "CurrentSwitchValues_GlobalVariable.vi" "16"() -> (w972:bool)
                    n1085 = global read "CurrentSwitchValues_GlobalVariable.vi" "2"() -> (w979:bool)
                    n1086 = global read "CurrentSwitchValues_GlobalVariable.vi" "6"() -> (w976:bool)
                    n1087 = global read "CurrentSwitchValues_GlobalVariable.vi" "4"() -> (w974:bool)
                    n1088 = global read "CurrentSwitchValues_GlobalVariable.vi" "8"() -> (w978:bool)
                    n1089 = global read "CurrentSwitchValues_GlobalVariable.vi" "18"() -> (w958:bool)
                    n1090 = global read "CurrentSwitchValues_GlobalVariable.vi" "20"() -> (w960:bool)
                    n1091 = global read "CurrentSwitchValues_GlobalVariable.vi" "22"() -> (w962:bool)
                    n1092 = global read "CurrentSwitchValues_GlobalVariable.vi" "24"() -> (w964:bool)
                    n1093 = global read "CurrentSwitchValues_GlobalVariable.vi" "26"() -> (w955:bool)
                    n1094 = global read "CurrentSwitchValues_GlobalVariable.vi" "28"() -> (w953:bool)
                    n1095 = global read "CurrentSwitchValues_GlobalVariable.vi" "30"() -> (w951:bool)
                    n1096 = property on="1" class="Bool (strict)"("Value"=w980) -> ()  [unwired: 2 in, 2 out]
                    n1097 = property on="3" class="Bool (strict)"("Value"=w973) -> ()  [unwired: 2 in, 2 out]
                    n1098 = property on="5" class="Bool (strict)"("Value"=w975) -> ()  [unwired: 2 in, 2 out]
                    n1099 = property on="7" class="Bool (strict)"("Value"=w977) -> ()  [unwired: 2 in, 2 out]
                    n1100 = property on="9" class="Bool (strict)"("Value"=w965) -> ()  [unwired: 2 in, 2 out]
                    n1101 = property on="11" class="Bool (strict)"("Value"=w967) -> ()  [unwired: 2 in, 2 out]
                    n1102 = property on="13" class="Bool (strict)"("Value"=w969) -> ()  [unwired: 2 in, 2 out]
                    n1103 = property on="15" class="Bool (strict)"("Value"=w971) -> ()  [unwired: 2 in, 2 out]
                    n1104 = property on="17" class="Bool (strict)"("Value"=w957) -> ()  [unwired: 2 in, 2 out]
                    n1105 = property on="19" class="Bool (strict)"("Value"=w959) -> ()  [unwired: 2 in, 2 out]
                    n1106 = property on="21" class="Bool (strict)"("Value"=w961) -> ()  [unwired: 2 in, 2 out]
                    n1107 = property on="23" class="Bool (strict)"("Value"=w963) -> ()  [unwired: 2 in, 2 out]
                    n1108 = property on="25" class="Bool (strict)"("Value"=w956) -> ()  [unwired: 2 in, 2 out]
                    n1109 = property on="27" class="Bool (strict)"("Value"=w954) -> ()  [unwired: 2 in, 2 out]
                    n1110 = property on="29" class="Bool (strict)"("Value"=w952) -> ()  [unwired: 2 in, 2 out]
                    n1111 = property on="26" class="Bool (strict)"("Value"=w955) -> ()  [unwired: 2 in, 2 out]
                    n1112 = property on="28" class="Bool (strict)"("Value"=w953) -> ()  [unwired: 2 in, 2 out]
                    n1113 = property on="30" class="Bool (strict)"("Value"=w951) -> ()  [unwired: 2 in, 2 out]
                    n1114 = property on="2" class="Bool (strict)"("Value"=w979) -> ()  [unwired: 2 in, 2 out]
                    n1115 = property on="4" class="Bool (strict)"("Value"=w974) -> ()  [unwired: 2 in, 2 out]
                    n1116 = property on="6" class="Bool (strict)"("Value"=w976) -> ()  [unwired: 2 in, 2 out]
                    n1117 = property on="8" class="Bool (strict)"("Value"=w978) -> ()  [unwired: 2 in, 2 out]
                    n1118 = property on="10" class="Bool (strict)"("Value"=w966) -> ()  [unwired: 2 in, 2 out]
                    n1119 = property on="12" class="Bool (strict)"("Value"=w968) -> ()  [unwired: 2 in, 2 out]
                    n1120 = property on="14" class="Bool (strict)"("Value"=w970) -> ()  [unwired: 2 in, 2 out]
                    n1121 = property on="16" class="Bool (strict)"("Value"=w972) -> ()  [unwired: 2 in, 2 out]
                    n1122 = property on="18" class="Bool (strict)"("Value"=w958) -> ()  [unwired: 2 in, 2 out]
                    n1123 = property on="20" class="Bool (strict)"("Value"=w960) -> ()  [unwired: 2 in, 2 out]
                    n1124 = property on="22" class="Bool (strict)"("Value"=w962) -> ()  [unwired: 2 in, 2 out]
                    n1125 = property on="24" class="Bool (strict)"("Value"=w964) -> ()  [unwired: 2 in, 2 out]
                  }
                }
              }
              frame #1 {
                # "Step 2:\nThe second part of the initialisation is to fill all of\nthe reaction chambers with the elution buffer."
                n1126 = stacked-sequence {
                  tunnel: w982 -> [w986 w1003 _]
                  tunnel: w981 -> [w985 w1004 _]
                  tunnel: [w983 _ _] -> _
                  tunnel: [_ w1002 _] -> _
                  frame #0 {
                    n1127 = for {
                      N: 200 -> [_]
                      tunnel: w986 -> [w991]
                      tunnel: w985 -> [w990]
                      tunnel: [w989] -> w983
                      i -> [w987]
                      n1128 = for {
                        N: 6 -> [_]
                        tunnel: w991 -> [w1001]
                        tunnel: w990 -> [w1000]
                        tunnel: [w999] -> w989
                        tunnel: w987 -> [w992]
                        i -> [w995]
                        n1129 = local read "Elution Buffer"() -> (w993:dbl)
                        n1130 = call "SequenceSelector_LoadAllChambers.vi"("Inflow Channel Selector"=w993, "Loop Iteration"=w992) -> ("Array"=w994:u8[][])  [unwired: 7 in]
                        n1131 = Index Array(array=w994, index (col)=w995) -> (element=w998:u8[])  [unwired: 1 in]
                        n1132 = Byte Array To String(unsigned byte array=w998) -> (string=w996:string)
                        n1133 = Enqueue Element(queue=w1001, element=w996, error in (no error)=w1000) -> (error out=w999:errorcluster)  [unwired: 1 in, 2 out]
                        n1134 = call "StorePreviousSwitchValues.vi"("Array"=w998) -> ()  [unwired: 3 in]
                        n1135 = Wait (ms)(milliseconds to wait=25) -> ()  [unwired: 1 out]
                      }
                    }
                  }
                  frame #1 {
                    w1006 = u8[] [0, 0, 0, 0, 0, 11, 0, 16, 0, 0, 0, 2, 4, 255, 7, 31, 255]
                    n1136 = Byte Array To String(unsigned byte array=w1006) -> (string=w1005:string)
                    n1137 = call "StorePreviousSwitchValues.vi"("Array"=w1006) -> ()  [unwired: 3 in]
                    n1138 = Enqueue Element(queue=w1003, element=w1005, error in (no error)=w1004) -> (error out=w1002:errorcluster)  [unwired: 1 in, 2 out]
                  }
                  frame #2 {
                    n1139 = global read "CurrentSwitchValues_GlobalVariable.vi" "1"() -> (w1036:bool)
                    n1140 = global read "CurrentSwitchValues_GlobalVariable.vi" "3"() -> (w1029:bool)
                    n1141 = global read "CurrentSwitchValues_GlobalVariable.vi" "5"() -> (w1031:bool)
                    n1142 = global read "CurrentSwitchValues_GlobalVariable.vi" "7"() -> (w1033:bool)
                    n1143 = global read "CurrentSwitchValues_GlobalVariable.vi" "9"() -> (w1021:bool)
                    n1144 = global read "CurrentSwitchValues_GlobalVariable.vi" "11"() -> (w1023:bool)
                    n1145 = global read "CurrentSwitchValues_GlobalVariable.vi" "13"() -> (w1025:bool)
                    n1146 = global read "CurrentSwitchValues_GlobalVariable.vi" "15"() -> (w1027:bool)
                    n1147 = global read "CurrentSwitchValues_GlobalVariable.vi" "17"() -> (w1013:bool)
                    n1148 = global read "CurrentSwitchValues_GlobalVariable.vi" "19"() -> (w1015:bool)
                    n1149 = global read "CurrentSwitchValues_GlobalVariable.vi" "21"() -> (w1017:bool)
                    n1150 = global read "CurrentSwitchValues_GlobalVariable.vi" "23"() -> (w1019:bool)
                    n1151 = global read "CurrentSwitchValues_GlobalVariable.vi" "25"() -> (w1012:bool)
                    n1152 = global read "CurrentSwitchValues_GlobalVariable.vi" "27"() -> (w1010:bool)
                    n1153 = global read "CurrentSwitchValues_GlobalVariable.vi" "29"() -> (w1008:bool)
                    n1154 = global read "CurrentSwitchValues_GlobalVariable.vi" "10"() -> (w1022:bool)
                    n1155 = global read "CurrentSwitchValues_GlobalVariable.vi" "12"() -> (w1024:bool)
                    n1156 = global read "CurrentSwitchValues_GlobalVariable.vi" "14"() -> (w1026:bool)
                    n1157 = global read "CurrentSwitchValues_GlobalVariable.vi" "16"() -> (w1028:bool)
                    n1158 = global read "CurrentSwitchValues_GlobalVariable.vi" "2"() -> (w1035:bool)
                    n1159 = global read "CurrentSwitchValues_GlobalVariable.vi" "6"() -> (w1032:bool)
                    n1160 = global read "CurrentSwitchValues_GlobalVariable.vi" "4"() -> (w1030:bool)
                    n1161 = global read "CurrentSwitchValues_GlobalVariable.vi" "8"() -> (w1034:bool)
                    n1162 = global read "CurrentSwitchValues_GlobalVariable.vi" "18"() -> (w1014:bool)
                    n1163 = global read "CurrentSwitchValues_GlobalVariable.vi" "20"() -> (w1016:bool)
                    n1164 = global read "CurrentSwitchValues_GlobalVariable.vi" "22"() -> (w1018:bool)
                    n1165 = global read "CurrentSwitchValues_GlobalVariable.vi" "24"() -> (w1020:bool)
                    n1166 = global read "CurrentSwitchValues_GlobalVariable.vi" "26"() -> (w1011:bool)
                    n1167 = global read "CurrentSwitchValues_GlobalVariable.vi" "28"() -> (w1009:bool)
                    n1168 = global read "CurrentSwitchValues_GlobalVariable.vi" "30"() -> (w1007:bool)
                    n1169 = property on="3" class="Bool (strict)"("Value"=w1029) -> ()  [unwired: 2 in, 2 out]
                    n1170 = property on="5" class="Bool (strict)"("Value"=w1031) -> ()  [unwired: 2 in, 2 out]
                    n1171 = property on="7" class="Bool (strict)"("Value"=w1033) -> ()  [unwired: 2 in, 2 out]
                    n1172 = property on="9" class="Bool (strict)"("Value"=w1021) -> ()  [unwired: 2 in, 2 out]
                    n1173 = property on="11" class="Bool (strict)"("Value"=w1023) -> ()  [unwired: 2 in, 2 out]
                    n1174 = property on="13" class="Bool (strict)"("Value"=w1025) -> ()  [unwired: 2 in, 2 out]
                    n1175 = property on="15" class="Bool (strict)"("Value"=w1027) -> ()  [unwired: 2 in, 2 out]
                    n1176 = property on="17" class="Bool (strict)"("Value"=w1013) -> ()  [unwired: 2 in, 2 out]
                    n1177 = property on="19" class="Bool (strict)"("Value"=w1015) -> ()  [unwired: 2 in, 2 out]
                    n1178 = property on="21" class="Bool (strict)"("Value"=w1017) -> ()  [unwired: 2 in, 2 out]
                    n1179 = property on="23" class="Bool (strict)"("Value"=w1019) -> ()  [unwired: 2 in, 2 out]
                    n1180 = property on="25" class="Bool (strict)"("Value"=w1012) -> ()  [unwired: 2 in, 2 out]
                    n1181 = property on="27" class="Bool (strict)"("Value"=w1010) -> ()  [unwired: 2 in, 2 out]
                    n1182 = property on="29" class="Bool (strict)"("Value"=w1008) -> ()  [unwired: 2 in, 2 out]
                    n1183 = property on="1" class="Bool (strict)"("Value"=w1036) -> ()  [unwired: 2 in, 2 out]
                    n1184 = property on="26" class="Bool (strict)"("Value"=w1011) -> ()  [unwired: 2 in, 2 out]
                    n1185 = property on="28" class="Bool (strict)"("Value"=w1009) -> ()  [unwired: 2 in, 2 out]
                    n1186 = property on="30" class="Bool (strict)"("Value"=w1007) -> ()  [unwired: 2 in, 2 out]
                    n1187 = property on="2" class="Bool (strict)"("Value"=w1035) -> ()  [unwired: 2 in, 2 out]
                    n1188 = property on="4" class="Bool (strict)"("Value"=w1030) -> ()  [unwired: 2 in, 2 out]
                    n1189 = property on="6" class="Bool (strict)"("Value"=w1032) -> ()  [unwired: 2 in, 2 out]
                    n1190 = property on="8" class="Bool (strict)"("Value"=w1034) -> ()  [unwired: 2 in, 2 out]
                    n1191 = property on="10" class="Bool (strict)"("Value"=w1022) -> ()  [unwired: 2 in, 2 out]
                    n1192 = property on="12" class="Bool (strict)"("Value"=w1024) -> ()  [unwired: 2 in, 2 out]
                    n1193 = property on="14" class="Bool (strict)"("Value"=w1026) -> ()  [unwired: 2 in, 2 out]
                    n1194 = property on="16" class="Bool (strict)"("Value"=w1028) -> ()  [unwired: 2 in, 2 out]
                    n1195 = property on="18" class="Bool (strict)"("Value"=w1014) -> ()  [unwired: 2 in, 2 out]
                    n1196 = property on="20" class="Bool (strict)"("Value"=w1016) -> ()  [unwired: 2 in, 2 out]
                    n1197 = property on="22" class="Bool (strict)"("Value"=w1018) -> ()  [unwired: 2 in, 2 out]
                    n1198 = property on="24" class="Bool (strict)"("Value"=w1020) -> ()  [unwired: 2 in, 2 out]
                  }
                }
              }
              frame #2 {
                # "Step 3:\n\nTo intitialise the device we need to prepare the device with\nidentical initial concentrations of all solvents as that will be used \nduring the dilution steps. This composition is as follows:\n25% DNA or MilliQ\n75 % IVTT Reaction Solution\n\nSince the feeding buffer comprises the largest portion of the \nreaction solution this will be injected first. \n\nNote: Here, all reactors will be initialised with 75 % IVTT Reaction \nSolution and 25 % MilliQ water. DNA will be added once the \nreaction dilutions have started."
                n1199 = stacked-sequence {
                  tunnel: w1038 -> [w1041 w1057 _]
                  tunnel: w1037 -> [w1040 w1058 _]
                  tunnel: [w1039 _ _] -> _
                  tunnel: [_ w1056 _] -> _
                  frame #0 {
                    n1200 = for {
                      N: 200 -> [_]
                      tunnel: w1041 -> [w1045]
                      tunnel: w1040 -> [w1044]
                      tunnel: [w1043] -> w1039
                      n1201 = for {
                        N: 6 -> [_]
                        tunnel: w1045 -> [w1050]
                        tunnel: w1044 -> [w1049]
                        tunnel: [w1048] -> w1043
                        i -> [w1054]
                        n1202 = local read "FB"() -> (w1047:dbl)
                        n1203 = call "SequenceSelector_Flush.vi"("Inflow Channel Selector"=w1047) -> ("Array"=w1053:u8[][])
                        n1204 = Wait (ms)(milliseconds to wait=25) -> ()  [unwired: 1 out]
                        n1205 = Index Array(array=w1053, index (col)=w1054) -> (element=w1055:u8[])  [unwired: 1 in]
                        n1206 = call "StorePreviousSwitchValues.vi"("Array"=w1055) -> ()  [unwired: 3 in]
                        n1207 = Byte Array To String(unsigned byte array=w1055) -> (string=w1051:string)
                        n1208 = Enqueue Element(queue=w1049, element=w1051, error in (no error)=w1050) -> (error out=w1048:errorcluster)  [unwired: 1 in, 2 out]
                      }
                    }
                  }
                  frame #1 {
                    w1060 = u8[] [0, 0, 0, 0, 0, 11, 0, 16, 0, 0, 0, 2, 4, 255, 7, 31, 255]
                    n1209 = call "StorePreviousSwitchValues.vi"("Array"=w1060) -> ()  [unwired: 3 in]
                    n1210 = Byte Array To String(unsigned byte array=w1060) -> (string=w1059:string)
                    n1211 = Enqueue Element(queue=w1058, element=w1059, error in (no error)=w1057) -> (error out=w1056:errorcluster)  [unwired: 1 in, 2 out]
                  }
                  frame #2 {
                    n1212 = global read "CurrentSwitchValues_GlobalVariable.vi" "1"() -> (w1090:bool)
                    n1213 = global read "CurrentSwitchValues_GlobalVariable.vi" "3"() -> (w1083:bool)
                    n1214 = global read "CurrentSwitchValues_GlobalVariable.vi" "5"() -> (w1085:bool)
                    n1215 = global read "CurrentSwitchValues_GlobalVariable.vi" "7"() -> (w1087:bool)
                    n1216 = global read "CurrentSwitchValues_GlobalVariable.vi" "9"() -> (w1075:bool)
                    n1217 = global read "CurrentSwitchValues_GlobalVariable.vi" "11"() -> (w1077:bool)
                    n1218 = global read "CurrentSwitchValues_GlobalVariable.vi" "13"() -> (w1079:bool)
                    n1219 = global read "CurrentSwitchValues_GlobalVariable.vi" "15"() -> (w1081:bool)
                    n1220 = global read "CurrentSwitchValues_GlobalVariable.vi" "17"() -> (w1067:bool)
                    n1221 = global read "CurrentSwitchValues_GlobalVariable.vi" "19"() -> (w1069:bool)
                    n1222 = global read "CurrentSwitchValues_GlobalVariable.vi" "21"() -> (w1071:bool)
                    n1223 = global read "CurrentSwitchValues_GlobalVariable.vi" "23"() -> (w1073:bool)
                    n1224 = global read "CurrentSwitchValues_GlobalVariable.vi" "25"() -> (w1066:bool)
                    n1225 = global read "CurrentSwitchValues_GlobalVariable.vi" "27"() -> (w1064:bool)
                    n1226 = global read "CurrentSwitchValues_GlobalVariable.vi" "29"() -> (w1062:bool)
                    n1227 = global read "CurrentSwitchValues_GlobalVariable.vi" "10"() -> (w1076:bool)
                    n1228 = global read "CurrentSwitchValues_GlobalVariable.vi" "12"() -> (w1078:bool)
                    n1229 = global read "CurrentSwitchValues_GlobalVariable.vi" "14"() -> (w1080:bool)
                    n1230 = global read "CurrentSwitchValues_GlobalVariable.vi" "16"() -> (w1082:bool)
                    n1231 = global read "CurrentSwitchValues_GlobalVariable.vi" "2"() -> (w1089:bool)
                    n1232 = global read "CurrentSwitchValues_GlobalVariable.vi" "6"() -> (w1086:bool)
                    n1233 = global read "CurrentSwitchValues_GlobalVariable.vi" "4"() -> (w1084:bool)
                    n1234 = global read "CurrentSwitchValues_GlobalVariable.vi" "8"() -> (w1088:bool)
                    n1235 = global read "CurrentSwitchValues_GlobalVariable.vi" "18"() -> (w1068:bool)
                    n1236 = global read "CurrentSwitchValues_GlobalVariable.vi" "20"() -> (w1070:bool)
                    n1237 = global read "CurrentSwitchValues_GlobalVariable.vi" "22"() -> (w1072:bool)
                    n1238 = global read "CurrentSwitchValues_GlobalVariable.vi" "24"() -> (w1074:bool)
                    n1239 = global read "CurrentSwitchValues_GlobalVariable.vi" "26"() -> (w1065:bool)
                    n1240 = global read "CurrentSwitchValues_GlobalVariable.vi" "28"() -> (w1063:bool)
                    n1241 = global read "CurrentSwitchValues_GlobalVariable.vi" "30"() -> (w1061:bool)
                    n1242 = property on="1" class="Bool (strict)"("Value"=w1090) -> ()  [unwired: 2 in, 2 out]
                    n1243 = property on="3" class="Bool (strict)"("Value"=w1083) -> ()  [unwired: 2 in, 2 out]
                    n1244 = property on="5" class="Bool (strict)"("Value"=w1085) -> ()  [unwired: 2 in, 2 out]
                    n1245 = property on="7" class="Bool (strict)"("Value"=w1087) -> ()  [unwired: 2 in, 2 out]
                    n1246 = property on="9" class="Bool (strict)"("Value"=w1075) -> ()  [unwired: 2 in, 2 out]
                    n1247 = property on="11" class="Bool (strict)"("Value"=w1077) -> ()  [unwired: 2 in, 2 out]
                    n1248 = property on="13" class="Bool (strict)"("Value"=w1079) -> ()  [unwired: 2 in, 2 out]
                    n1249 = property on="15" class="Bool (strict)"("Value"=w1081) -> ()  [unwired: 2 in, 2 out]
                    n1250 = property on="17" class="Bool (strict)"("Value"=w1067) -> ()  [unwired: 2 in, 2 out]
                    n1251 = property on="19" class="Bool (strict)"("Value"=w1069) -> ()  [unwired: 2 in, 2 out]
                    n1252 = property on="21" class="Bool (strict)"("Value"=w1071) -> ()  [unwired: 2 in, 2 out]
                    n1253 = property on="23" class="Bool (strict)"("Value"=w1073) -> ()  [unwired: 2 in, 2 out]
                    n1254 = property on="25" class="Bool (strict)"("Value"=w1066) -> ()  [unwired: 2 in, 2 out]
                    n1255 = property on="27" class="Bool (strict)"("Value"=w1064) -> ()  [unwired: 2 in, 2 out]
                    n1256 = property on="29" class="Bool (strict)"("Value"=w1062) -> ()  [unwired: 2 in, 2 out]
                    n1257 = property on="26" class="Bool (strict)"("Value"=w1065) -> ()  [unwired: 2 in, 2 out]
                    n1258 = property on="28" class="Bool (strict)"("Value"=w1063) -> ()  [unwired: 2 in, 2 out]
                    n1259 = property on="30" class="Bool (strict)"("Value"=w1061) -> ()  [unwired: 2 in, 2 out]
                    n1260 = property on="2" class="Bool (strict)"("Value"=w1089) -> ()  [unwired: 2 in, 2 out]
                    n1261 = property on="4" class="Bool (strict)"("Value"=w1084) -> ()  [unwired: 2 in, 2 out]
                    n1262 = property on="6" class="Bool (strict)"("Value"=w1086) -> ()  [unwired: 2 in, 2 out]
                    n1263 = property on="8" class="Bool (strict)"("Value"=w1088) -> ()  [unwired: 2 in, 2 out]
                    n1264 = property on="10" class="Bool (strict)"("Value"=w1076) -> ()  [unwired: 2 in, 2 out]
                    n1265 = property on="12" class="Bool (strict)"("Value"=w1078) -> ()  [unwired: 2 in, 2 out]
                    n1266 = property on="14" class="Bool (strict)"("Value"=w1080) -> ()  [unwired: 2 in, 2 out]
                    n1267 = property on="16" class="Bool (strict)"("Value"=w1082) -> ()  [unwired: 2 in, 2 out]
                    n1268 = property on="18" class="Bool (strict)"("Value"=w1068) -> ()  [unwired: 2 in, 2 out]
                    n1269 = property on="20" class="Bool (strict)"("Value"=w1070) -> ()  [unwired: 2 in, 2 out]
                    n1270 = property on="22" class="Bool (strict)"("Value"=w1072) -> ()  [unwired: 2 in, 2 out]
                    n1271 = property on="24" class="Bool (strict)"("Value"=w1074) -> ()  [unwired: 2 in, 2 out]
                  }
                }
              }
              frame #3 {
                # "Step 4:\nStep four involves fully filling\neach of the reactors with IVTT \nreaction solution, since this forms the \ngross of the initialised volume. 25% of this volume \nwill be displaced with the milliQ at a later stage."
                n1272 = stacked-sequence {
                  tunnel: w1092 -> [w1096 w1113 _]
                  tunnel: w1091 -> [w1095 w1114 _]
                  tunnel: [w1094 _ _] -> _
                  tunnel: [_ w1112 _] -> _
                  frame #0 {
                    n1273 = for {
                      N: 200 -> [_]
                      tunnel: w1096 -> [w1101]
                      tunnel: w1095 -> [w1100]
                      tunnel: [w1099] -> w1094
                      i -> [w1097]
                      n1274 = for {
                        N: 6 -> [_]
                        tunnel: w1101 -> [w1111]
                        tunnel: w1100 -> [w1110]
                        tunnel: [w1109] -> w1099
                        tunnel: w1097 -> [w1102]
                        i -> [w1105]
                        n1275 = local read "FB"() -> (w1103:dbl)
                        n1276 = call "SequenceSelector_LoadAllChambers.vi"("Inflow Channel Selector"=w1103, "Loop Iteration"=w1102) -> ("Array"=w1104:u8[][])  [unwired: 7 in]
                        n1277 = Index Array(array=w1104, index (col)=w1105) -> (element=w1108:u8[])  [unwired: 1 in]
                        n1278 = Byte Array To String(unsigned byte array=w1108) -> (string=w1106:string)
                        n1279 = Enqueue Element(queue=w1111, element=w1106, error in (no error)=w1110) -> (error out=w1109:errorcluster)  [unwired: 1 in, 2 out]
                        n1280 = call "StorePreviousSwitchValues.vi"("Array"=w1108) -> ()  [unwired: 3 in]
                        n1281 = Wait (ms)(milliseconds to wait=15) -> ()  [unwired: 1 out]
                      }
                    }
                  }
                  frame #1 {
                    w1116 = u8[] [0, 0, 0, 0, 0, 11, 0, 16, 0, 0, 0, 2, 4, 255, 7, 31, 255]
                    n1282 = Byte Array To String(unsigned byte array=w1116) -> (string=w1115:string)
                    n1283 = call "StorePreviousSwitchValues.vi"("Array"=w1116) -> ()  [unwired: 3 in]
                    n1284 = Enqueue Element(queue=w1113, element=w1115, error in (no error)=w1114) -> (error out=w1112:errorcluster)  [unwired: 1 in, 2 out]
                  }
                  frame #2 {
                    n1285 = global read "CurrentSwitchValues_GlobalVariable.vi" "1"() -> (w1146:bool)
                    n1286 = global read "CurrentSwitchValues_GlobalVariable.vi" "3"() -> (w1139:bool)
                    n1287 = global read "CurrentSwitchValues_GlobalVariable.vi" "5"() -> (w1141:bool)
                    n1288 = global read "CurrentSwitchValues_GlobalVariable.vi" "7"() -> (w1143:bool)
                    n1289 = global read "CurrentSwitchValues_GlobalVariable.vi" "9"() -> (w1131:bool)
                    n1290 = global read "CurrentSwitchValues_GlobalVariable.vi" "11"() -> (w1133:bool)
                    n1291 = global read "CurrentSwitchValues_GlobalVariable.vi" "13"() -> (w1135:bool)
                    n1292 = global read "CurrentSwitchValues_GlobalVariable.vi" "15"() -> (w1137:bool)
                    n1293 = global read "CurrentSwitchValues_GlobalVariable.vi" "17"() -> (w1123:bool)
                    n1294 = global read "CurrentSwitchValues_GlobalVariable.vi" "19"() -> (w1125:bool)
                    n1295 = global read "CurrentSwitchValues_GlobalVariable.vi" "21"() -> (w1127:bool)
                    n1296 = global read "CurrentSwitchValues_GlobalVariable.vi" "23"() -> (w1129:bool)
                    n1297 = global read "CurrentSwitchValues_GlobalVariable.vi" "25"() -> (w1122:bool)
                    n1298 = global read "CurrentSwitchValues_GlobalVariable.vi" "27"() -> (w1120:bool)
                    n1299 = global read "CurrentSwitchValues_GlobalVariable.vi" "29"() -> (w1118:bool)
                    n1300 = global read "CurrentSwitchValues_GlobalVariable.vi" "10"() -> (w1132:bool)
                    n1301 = global read "CurrentSwitchValues_GlobalVariable.vi" "12"() -> (w1134:bool)
                    n1302 = global read "CurrentSwitchValues_GlobalVariable.vi" "14"() -> (w1136:bool)
                    n1303 = global read "CurrentSwitchValues_GlobalVariable.vi" "16"() -> (w1138:bool)
                    n1304 = global read "CurrentSwitchValues_GlobalVariable.vi" "2"() -> (w1145:bool)
                    n1305 = global read "CurrentSwitchValues_GlobalVariable.vi" "6"() -> (w1142:bool)
                    n1306 = global read "CurrentSwitchValues_GlobalVariable.vi" "4"() -> (w1140:bool)
                    n1307 = global read "CurrentSwitchValues_GlobalVariable.vi" "8"() -> (w1144:bool)
                    n1308 = global read "CurrentSwitchValues_GlobalVariable.vi" "18"() -> (w1124:bool)
                    n1309 = global read "CurrentSwitchValues_GlobalVariable.vi" "20"() -> (w1126:bool)
                    n1310 = global read "CurrentSwitchValues_GlobalVariable.vi" "22"() -> (w1128:bool)
                    n1311 = global read "CurrentSwitchValues_GlobalVariable.vi" "24"() -> (w1130:bool)
                    n1312 = global read "CurrentSwitchValues_GlobalVariable.vi" "26"() -> (w1121:bool)
                    n1313 = global read "CurrentSwitchValues_GlobalVariable.vi" "28"() -> (w1119:bool)
                    n1314 = global read "CurrentSwitchValues_GlobalVariable.vi" "30"() -> (w1117:bool)
                    n1315 = property on="3" class="Bool (strict)"("Value"=w1139) -> ()  [unwired: 2 in, 2 out]
                    n1316 = property on="5" class="Bool (strict)"("Value"=w1141) -> ()  [unwired: 2 in, 2 out]
                    n1317 = property on="7" class="Bool (strict)"("Value"=w1143) -> ()  [unwired: 2 in, 2 out]
                    n1318 = property on="9" class="Bool (strict)"("Value"=w1131) -> ()  [unwired: 2 in, 2 out]
                    n1319 = property on="11" class="Bool (strict)"("Value"=w1133) -> ()  [unwired: 2 in, 2 out]
                    n1320 = property on="13" class="Bool (strict)"("Value"=w1135) -> ()  [unwired: 2 in, 2 out]
                    n1321 = property on="15" class="Bool (strict)"("Value"=w1137) -> ()  [unwired: 2 in, 2 out]
                    n1322 = property on="17" class="Bool (strict)"("Value"=w1123) -> ()  [unwired: 2 in, 2 out]
                    n1323 = property on="19" class="Bool (strict)"("Value"=w1125) -> ()  [unwired: 2 in, 2 out]
                    n1324 = property on="21" class="Bool (strict)"("Value"=w1127) -> ()  [unwired: 2 in, 2 out]
                    n1325 = property on="23" class="Bool (strict)"("Value"=w1129) -> ()  [unwired: 2 in, 2 out]
                    n1326 = property on="25" class="Bool (strict)"("Value"=w1122) -> ()  [unwired: 2 in, 2 out]
                    n1327 = property on="27" class="Bool (strict)"("Value"=w1120) -> ()  [unwired: 2 in, 2 out]
                    n1328 = property on="29" class="Bool (strict)"("Value"=w1118) -> ()  [unwired: 2 in, 2 out]
                    n1329 = property on="1" class="Bool (strict)"("Value"=w1146) -> ()  [unwired: 2 in, 2 out]
                    n1330 = property on="26" class="Bool (strict)"("Value"=w1121) -> ()  [unwired: 2 in, 2 out]
                    n1331 = property on="28" class="Bool (strict)"("Value"=w1119) -> ()  [unwired: 2 in, 2 out]
                    n1332 = property on="30" class="Bool (strict)"("Value"=w1117) -> ()  [unwired: 2 in, 2 out]
                    n1333 = property on="2" class="Bool (strict)"("Value"=w1145) -> ()  [unwired: 2 in, 2 out]
                    n1334 = property on="4" class="Bool (strict)"("Value"=w1140) -> ()  [unwired: 2 in, 2 out]
                    n1335 = property on="6" class="Bool (strict)"("Value"=w1142) -> ()  [unwired: 2 in, 2 out]
                    n1336 = property on="8" class="Bool (strict)"("Value"=w1144) -> ()  [unwired: 2 in, 2 out]
                    n1337 = property on="10" class="Bool (strict)"("Value"=w1132) -> ()  [unwired: 2 in, 2 out]
                    n1338 = property on="12" class="Bool (strict)"("Value"=w1134) -> ()  [unwired: 2 in, 2 out]
                    n1339 = property on="14" class="Bool (strict)"("Value"=w1136) -> ()  [unwired: 2 in, 2 out]
                    n1340 = property on="16" class="Bool (strict)"("Value"=w1138) -> ()  [unwired: 2 in, 2 out]
                    n1341 = property on="18" class="Bool (strict)"("Value"=w1124) -> ()  [unwired: 2 in, 2 out]
                    n1342 = property on="20" class="Bool (strict)"("Value"=w1126) -> ()  [unwired: 2 in, 2 out]
                    n1343 = property on="22" class="Bool (strict)"("Value"=w1128) -> ()  [unwired: 2 in, 2 out]
                    n1344 = property on="24" class="Bool (strict)"("Value"=w1130) -> ()  [unwired: 2 in, 2 out]
                  }
                }
              }
              frame #4 {
                # "Step 5:\nNext in the initialisation process, the milliQ water \n(elution buffer) is added. As such the reagent is \nfirst flushed into the device."
                n1345 = stacked-sequence {
                  tunnel: w1148 -> [w1151 w1166 _]
                  tunnel: w1147 -> [w1150 w1167 _]
                  tunnel: [w1149 _ _] -> _
                  frame #0 {
                    n1346 = for {
                      N: 200 -> [_]
                      tunnel: w1151 -> [w1155]
                      tunnel: w1150 -> [w1154]
                      tunnel: [w1153] -> w1149
                      n1347 = for {
                        N: 6 -> [_]
                        tunnel: w1155 -> [w1160]
                        tunnel: w1154 -> [w1159]
                        tunnel: [w1158] -> w1153
                        i -> [w1164]
                        # "T-wait is 100 ms,\nfreq = +-1.7Hz if fast and T-wait is 556ms, freq = 0.3Hz if slow flush."
                        n1348 = local read "Elution Buffer"() -> (w1157:dbl)
                        n1349 = call "SequenceSelector_Flush.vi"("Inflow Channel Selector"=w1157) -> ("Array"=w1163:u8[][])
                        n1350 = Wait (ms)(milliseconds to wait=25) -> ()  [unwired: 1 out]
                        n1351 = Index Array(array=w1163, index (col)=w1164) -> (element=w1165:u8[])  [unwired: 1 in]
                        n1352 = call "StorePreviousSwitchValues.vi"("Array"=w1165) -> ()  [unwired: 3 in]
                        n1353 = Byte Array To String(unsigned byte array=w1165) -> (string=w1161:string)
                        n1354 = Enqueue Element(queue=w1159, element=w1161, error in (no error)=w1160) -> (error out=w1158:errorcluster)  [unwired: 1 in, 2 out]
                      }
                    }
                  }
                  frame #1 {
                    w1169 = u8[] [0, 0, 0, 0, 0, 11, 0, 16, 0, 0, 0, 2, 4, 255, 7, 31, 255]
                    n1355 = call "StorePreviousSwitchValues.vi"("Array"=w1169) -> ()  [unwired: 3 in]
                    n1356 = Byte Array To String(unsigned byte array=w1169) -> (string=w1168:string)
                    n1357 = Enqueue Element(queue=w1167, element=w1168, error in (no error)=w1166) -> ()  [unwired: 1 in, 3 out]
                  }
                  frame #2 {
                    n1358 = global read "CurrentSwitchValues_GlobalVariable.vi" "1"() -> (w1199:bool)
                    n1359 = global read "CurrentSwitchValues_GlobalVariable.vi" "3"() -> (w1192:bool)
                    n1360 = global read "CurrentSwitchValues_GlobalVariable.vi" "5"() -> (w1194:bool)
                    n1361 = global read "CurrentSwitchValues_GlobalVariable.vi" "7"() -> (w1196:bool)
                    n1362 = global read "CurrentSwitchValues_GlobalVariable.vi" "9"() -> (w1184:bool)
                    n1363 = global read "CurrentSwitchValues_GlobalVariable.vi" "11"() -> (w1186:bool)
                    n1364 = global read "CurrentSwitchValues_GlobalVariable.vi" "13"() -> (w1188:bool)
                    n1365 = global read "CurrentSwitchValues_GlobalVariable.vi" "15"() -> (w1190:bool)
                    n1366 = global read "CurrentSwitchValues_GlobalVariable.vi" "17"() -> (w1176:bool)
                    n1367 = global read "CurrentSwitchValues_GlobalVariable.vi" "19"() -> (w1178:bool)
                    n1368 = global read "CurrentSwitchValues_GlobalVariable.vi" "21"() -> (w1180:bool)
                    n1369 = global read "CurrentSwitchValues_GlobalVariable.vi" "23"() -> (w1182:bool)
                    n1370 = global read "CurrentSwitchValues_GlobalVariable.vi" "25"() -> (w1175:bool)
                    n1371 = global read "CurrentSwitchValues_GlobalVariable.vi" "27"() -> (w1173:bool)
                    n1372 = global read "CurrentSwitchValues_GlobalVariable.vi" "29"() -> (w1171:bool)
                    n1373 = global read "CurrentSwitchValues_GlobalVariable.vi" "10"() -> (w1185:bool)
                    n1374 = global read "CurrentSwitchValues_GlobalVariable.vi" "12"() -> (w1187:bool)
                    n1375 = global read "CurrentSwitchValues_GlobalVariable.vi" "14"() -> (w1189:bool)
                    n1376 = global read "CurrentSwitchValues_GlobalVariable.vi" "16"() -> (w1191:bool)
                    n1377 = global read "CurrentSwitchValues_GlobalVariable.vi" "2"() -> (w1198:bool)
                    n1378 = global read "CurrentSwitchValues_GlobalVariable.vi" "6"() -> (w1195:bool)
                    n1379 = global read "CurrentSwitchValues_GlobalVariable.vi" "4"() -> (w1193:bool)
                    n1380 = global read "CurrentSwitchValues_GlobalVariable.vi" "8"() -> (w1197:bool)
                    n1381 = global read "CurrentSwitchValues_GlobalVariable.vi" "18"() -> (w1177:bool)
                    n1382 = global read "CurrentSwitchValues_GlobalVariable.vi" "20"() -> (w1179:bool)
                    n1383 = global read "CurrentSwitchValues_GlobalVariable.vi" "22"() -> (w1181:bool)
                    n1384 = global read "CurrentSwitchValues_GlobalVariable.vi" "24"() -> (w1183:bool)
                    n1385 = global read "CurrentSwitchValues_GlobalVariable.vi" "26"() -> (w1174:bool)
                    n1386 = global read "CurrentSwitchValues_GlobalVariable.vi" "28"() -> (w1172:bool)
                    n1387 = global read "CurrentSwitchValues_GlobalVariable.vi" "30"() -> (w1170:bool)
                    n1388 = property on="1" class="Bool (strict)"("Value"=w1199) -> ()  [unwired: 2 in, 2 out]
                    n1389 = property on="3" class="Bool (strict)"("Value"=w1192) -> ()  [unwired: 2 in, 2 out]
                    n1390 = property on="5" class="Bool (strict)"("Value"=w1194) -> ()  [unwired: 2 in, 2 out]
                    n1391 = property on="7" class="Bool (strict)"("Value"=w1196) -> ()  [unwired: 2 in, 2 out]
                    n1392 = property on="9" class="Bool (strict)"("Value"=w1184) -> ()  [unwired: 2 in, 2 out]
                    n1393 = property on="11" class="Bool (strict)"("Value"=w1186) -> ()  [unwired: 2 in, 2 out]
                    n1394 = property on="13" class="Bool (strict)"("Value"=w1188) -> ()  [unwired: 2 in, 2 out]
                    n1395 = property on="15" class="Bool (strict)"("Value"=w1190) -> ()  [unwired: 2 in, 2 out]
                    n1396 = property on="17" class="Bool (strict)"("Value"=w1176) -> ()  [unwired: 2 in, 2 out]
                    n1397 = property on="19" class="Bool (strict)"("Value"=w1178) -> ()  [unwired: 2 in, 2 out]
                    n1398 = property on="21" class="Bool (strict)"("Value"=w1180) -> ()  [unwired: 2 in, 2 out]
                    n1399 = property on="23" class="Bool (strict)"("Value"=w1182) -> ()  [unwired: 2 in, 2 out]
                    n1400 = property on="25" class="Bool (strict)"("Value"=w1175) -> ()  [unwired: 2 in, 2 out]
                    n1401 = property on="27" class="Bool (strict)"("Value"=w1173) -> ()  [unwired: 2 in, 2 out]
                    n1402 = property on="29" class="Bool (strict)"("Value"=w1171) -> ()  [unwired: 2 in, 2 out]
                    n1403 = property on="26" class="Bool (strict)"("Value"=w1174) -> ()  [unwired: 2 in, 2 out]
                    n1404 = property on="28" class="Bool (strict)"("Value"=w1172) -> ()  [unwired: 2 in, 2 out]
                    n1405 = property on="30" class="Bool (strict)"("Value"=w1170) -> ()  [unwired: 2 in, 2 out]
                    n1406 = property on="2" class="Bool (strict)"("Value"=w1198) -> ()  [unwired: 2 in, 2 out]
                    n1407 = property on="4" class="Bool (strict)"("Value"=w1193) -> ()  [unwired: 2 in, 2 out]
                    n1408 = property on="6" class="Bool (strict)"("Value"=w1195) -> ()  [unwired: 2 in, 2 out]
                    n1409 = property on="8" class="Bool (strict)"("Value"=w1197) -> ()  [unwired: 2 in, 2 out]
                    n1410 = property on="10" class="Bool (strict)"("Value"=w1185) -> ()  [unwired: 2 in, 2 out]
                    n1411 = property on="12" class="Bool (strict)"("Value"=w1187) -> ()  [unwired: 2 in, 2 out]
                    n1412 = property on="14" class="Bool (strict)"("Value"=w1189) -> ()  [unwired: 2 in, 2 out]
                    n1413 = property on="16" class="Bool (strict)"("Value"=w1191) -> ()  [unwired: 2 in, 2 out]
                    n1414 = property on="18" class="Bool (strict)"("Value"=w1177) -> ()  [unwired: 2 in, 2 out]
                    n1415 = property on="20" class="Bool (strict)"("Value"=w1179) -> ()  [unwired: 2 in, 2 out]
                    n1416 = property on="22" class="Bool (strict)"("Value"=w1181) -> ()  [unwired: 2 in, 2 out]
                    n1417 = property on="24" class="Bool (strict)"("Value"=w1183) -> ()  [unwired: 2 in, 2 out]
                  }
                }
              }
              frame #5 {
                # "Step 6:\nThe sixth part of the initialisation is to fill 25% of the\nreaction chamber with milliQ Water. \nThe final composition after initialisation will \nbe as follows:\n25% MilliQ\n75% IVTT Reaction Solution"
                n1418 = stacked-sequence {
                  tunnel: w1201 -> [w1205 w1233 _]
                  tunnel: w1200 -> [w1204 w1234 _]
                  tunnel: [w1203 _ _] -> _
                  tunnel: [_ w1232 _] -> _
                  frame #0 {
                    n1419 = for {
                      N: 8 -> [_]
                      tunnel: w1205 -> [w1214]
                      shift-right: [w1212] -> w1203
                      shift-left: w1204 -> [w1213]
                      i -> [w1208]
                      n1420 = local read "Elution Buffer RR"() -> (w1211:dbl)
                      n1421 = Add(x=w1208, y=1) -> (x+y=w1210:i32)
                      n1422 = global write "CurrentSwitchValues_GlobalVariable.vi" "Current Reactor"(w1210) -> ()
                      n1423 = call "ConvertDesiredRefreshRatioPerReactor.vi"("Desired Refresh Ratio"=w1211, "Reactor"=w1208) -> ("Required Number of Pump Iterations"=w1207:dbl)
                      n1424 = Round To Nearest(number=w1207) -> (nearest integer value=w1206:dbl)
                      n1425 = for {
                        N: w1206 -> [_]
                        tunnel: w1214 -> [w1219]
                        tunnel: w1213 -> [w1218]
                        tunnel: [w1217] -> w1212
                        i -> [w1215]
                        n1426 = for {
                          N: 6 -> [_]
                          tunnel: w1219 -> [w1231]
                          tunnel: w1218 -> [w1230]
                          tunnel: [w1229] -> w1217
                          tunnel: w1215 -> [w1221]
                          i -> [w1225]
                          w1220 = TRUE
                          n1427 = global read "CurrentSwitchValues_GlobalVariable.vi" "Current Reactor"() -> (w1223:dbl)
                          n1428 = local read "Elution Buffer"() -> (w1222:dbl)
                          n1429 = call "SequenceSelector_LoadPerReactor.vi"("Reactor 6"=w1220, "Reactor 7"=w1220, "Reactor 8"=w1220, "Loop Iteration"=w1221, "Reactor 5"=w1220, "Reactor 4"=w1220, "Current Reactor"=w1223, "Reactor 3"=w1220, "Reactor 2"=w1220, "Reactor 1"=w1220, "Inflow Channel Selector"=w1222) -> ("Array"=w1224:u8[][])
                          n1430 = Index Array(array=w1224, index (col)=w1225) -> (element=w1228:u8[])  [unwired: 1 in]
                          n1431 = Byte Array To String(unsigned byte array=w1228) -> (string=w1226:string)
                          n1432 = Enqueue Element(queue=w1231, element=w1226, error in (no error)=w1230) -> (error out=w1229:errorcluster)  [unwired: 1 in, 2 out]
                          n1433 = call "StorePreviousSwitchValues.vi"("Array"=w1228) -> ()  [unwired: 3 in]
                          n1434 = Wait (ms)(milliseconds to wait=15) -> ()  [unwired: 1 out]
                        }
                      }
                    }
                  }
                  frame #1 {
                    w1236 = u8[] [0, 0, 0, 0, 0, 11, 0, 16, 0, 0, 0, 2, 4, 255, 7, 31, 255]
                    n1435 = Byte Array To String(unsigned byte array=w1236) -> (string=w1235:string)
                    n1436 = call "StorePreviousSwitchValues.vi"("Array"=w1236) -> ()  [unwired: 3 in]
                    n1437 = Enqueue Element(queue=w1233, element=w1235, error in (no error)=w1234) -> (error out=w1232:errorcluster)  [unwired: 1 in, 2 out]
                  }
                  frame #2 {
                    n1438 = global read "CurrentSwitchValues_GlobalVariable.vi" "1"() -> (w1266:bool)
                    n1439 = global read "CurrentSwitchValues_GlobalVariable.vi" "3"() -> (w1259:bool)
                    n1440 = global read "CurrentSwitchValues_GlobalVariable.vi" "5"() -> (w1261:bool)
                    n1441 = global read "CurrentSwitchValues_GlobalVariable.vi" "7"() -> (w1263:bool)
                    n1442 = global read "CurrentSwitchValues_GlobalVariable.vi" "9"() -> (w1251:bool)
                    n1443 = global read "CurrentSwitchValues_GlobalVariable.vi" "11"() -> (w1253:bool)
                    n1444 = global read "CurrentSwitchValues_GlobalVariable.vi" "13"() -> (w1255:bool)
                    n1445 = global read "CurrentSwitchValues_GlobalVariable.vi" "15"() -> (w1257:bool)
                    n1446 = global read "CurrentSwitchValues_GlobalVariable.vi" "17"() -> (w1243:bool)
                    n1447 = global read "CurrentSwitchValues_GlobalVariable.vi" "19"() -> (w1245:bool)
                    n1448 = global read "CurrentSwitchValues_GlobalVariable.vi" "21"() -> (w1247:bool)
                    n1449 = global read "CurrentSwitchValues_GlobalVariable.vi" "23"() -> (w1249:bool)
                    n1450 = global read "CurrentSwitchValues_GlobalVariable.vi" "25"() -> (w1242:bool)
                    n1451 = global read "CurrentSwitchValues_GlobalVariable.vi" "27"() -> (w1240:bool)
                    n1452 = global read "CurrentSwitchValues_GlobalVariable.vi" "29"() -> (w1238:bool)
                    n1453 = global read "CurrentSwitchValues_GlobalVariable.vi" "10"() -> (w1252:bool)
                    n1454 = global read "CurrentSwitchValues_GlobalVariable.vi" "12"() -> (w1254:bool)
                    n1455 = global read "CurrentSwitchValues_GlobalVariable.vi" "14"() -> (w1256:bool)
                    n1456 = global read "CurrentSwitchValues_GlobalVariable.vi" "16"() -> (w1258:bool)
                    n1457 = global read "CurrentSwitchValues_GlobalVariable.vi" "2"() -> (w1265:bool)
                    n1458 = global read "CurrentSwitchValues_GlobalVariable.vi" "6"() -> (w1262:bool)
                    n1459 = global read "CurrentSwitchValues_GlobalVariable.vi" "4"() -> (w1260:bool)
                    n1460 = global read "CurrentSwitchValues_GlobalVariable.vi" "8"() -> (w1264:bool)
                    n1461 = global read "CurrentSwitchValues_GlobalVariable.vi" "18"() -> (w1244:bool)
                    n1462 = global read "CurrentSwitchValues_GlobalVariable.vi" "20"() -> (w1246:bool)
                    n1463 = global read "CurrentSwitchValues_GlobalVariable.vi" "22"() -> (w1248:bool)
                    n1464 = global read "CurrentSwitchValues_GlobalVariable.vi" "24"() -> (w1250:bool)
                    n1465 = global read "CurrentSwitchValues_GlobalVariable.vi" "26"() -> (w1241:bool)
                    n1466 = global read "CurrentSwitchValues_GlobalVariable.vi" "28"() -> (w1239:bool)
                    n1467 = global read "CurrentSwitchValues_GlobalVariable.vi" "30"() -> (w1237:bool)
                    n1468 = property on="3" class="Bool (strict)"("Value"=w1259) -> ()  [unwired: 2 in, 2 out]
                    n1469 = property on="5" class="Bool (strict)"("Value"=w1261) -> ()  [unwired: 2 in, 2 out]
                    n1470 = property on="7" class="Bool (strict)"("Value"=w1263) -> ()  [unwired: 2 in, 2 out]
                    n1471 = property on="9" class="Bool (strict)"("Value"=w1251) -> ()  [unwired: 2 in, 2 out]
                    n1472 = property on="11" class="Bool (strict)"("Value"=w1253) -> ()  [unwired: 2 in, 2 out]
                    n1473 = property on="13" class="Bool (strict)"("Value"=w1255) -> ()  [unwired: 2 in, 2 out]
                    n1474 = property on="15" class="Bool (strict)"("Value"=w1257) -> ()  [unwired: 2 in, 2 out]
                    n1475 = property on="17" class="Bool (strict)"("Value"=w1243) -> ()  [unwired: 2 in, 2 out]
                    n1476 = property on="19" class="Bool (strict)"("Value"=w1245) -> ()  [unwired: 2 in, 2 out]
                    n1477 = property on="21" class="Bool (strict)"("Value"=w1247) -> ()  [unwired: 2 in, 2 out]
                    n1478 = property on="23" class="Bool (strict)"("Value"=w1249) -> ()  [unwired: 2 in, 2 out]
                    n1479 = property on="25" class="Bool (strict)"("Value"=w1242) -> ()  [unwired: 2 in, 2 out]
                    n1480 = property on="27" class="Bool (strict)"("Value"=w1240) -> ()  [unwired: 2 in, 2 out]
                    n1481 = property on="29" class="Bool (strict)"("Value"=w1238) -> ()  [unwired: 2 in, 2 out]
                    n1482 = property on="1" class="Bool (strict)"("Value"=w1266) -> ()  [unwired: 2 in, 2 out]
                    n1483 = property on="26" class="Bool (strict)"("Value"=w1241) -> ()  [unwired: 2 in, 2 out]
                    n1484 = property on="28" class="Bool (strict)"("Value"=w1239) -> ()  [unwired: 2 in, 2 out]
                    n1485 = property on="30" class="Bool (strict)"("Value"=w1237) -> ()  [unwired: 2 in, 2 out]
                    n1486 = property on="2" class="Bool (strict)"("Value"=w1265) -> ()  [unwired: 2 in, 2 out]
                    n1487 = property on="4" class="Bool (strict)"("Value"=w1260) -> ()  [unwired: 2 in, 2 out]
                    n1488 = property on="6" class="Bool (strict)"("Value"=w1262) -> ()  [unwired: 2 in, 2 out]
                    n1489 = property on="8" class="Bool (strict)"("Value"=w1264) -> ()  [unwired: 2 in, 2 out]
                    n1490 = property on="10" class="Bool (strict)"("Value"=w1252) -> ()  [unwired: 2 in, 2 out]
                    n1491 = property on="12" class="Bool (strict)"("Value"=w1254) -> ()  [unwired: 2 in, 2 out]
                    n1492 = property on="14" class="Bool (strict)"("Value"=w1256) -> ()  [unwired: 2 in, 2 out]
                    n1493 = property on="16" class="Bool (strict)"("Value"=w1258) -> ()  [unwired: 2 in, 2 out]
                    n1494 = property on="18" class="Bool (strict)"("Value"=w1244) -> ()  [unwired: 2 in, 2 out]
                    n1495 = property on="20" class="Bool (strict)"("Value"=w1246) -> ()  [unwired: 2 in, 2 out]
                    n1496 = property on="22" class="Bool (strict)"("Value"=w1248) -> ()  [unwired: 2 in, 2 out]
                    n1497 = property on="24" class="Bool (strict)"("Value"=w1250) -> ()  [unwired: 2 in, 2 out]
                  }
                }
              }
              frame #6 {
                # "Step 7: Before taking the first image of the experiment, the reaction chamber is mixed to ensure a homogeneous distribution of the reaction solvents."
                n1498 = stacked-sequence {
                  tunnel: w1267 -> [w1272 w1304 _]
                  tunnel: w1268 -> [w1271 w1303 _]
                  tunnel: [w1270 _ _] -> _
                  frame #0 {
                    n1499 = local read "Number of Mixing Cycles Initialisation"() -> (w1269:dbl)
                    n1500 = for {
                      N: w1269 -> [_]
                      tunnel: w1272 -> [w1276]
                      tunnel: w1271 -> [w1275]
                      tunnel: [w1274] -> w1270
                      i -> [w1281]
                      n1501 = local read "Number of Mixing Cycles Initialisation"() -> (w1273:dbl)
                      n1502 = for {
                        N: 500 -> [_]
                        tunnel: w1276 -> [w1293]
                        tunnel: w1275 -> [w1292]
                        tunnel: [w1291] -> w1274
                        n1503 = for {
                          N: 6 -> [_]
                          tunnel: w1293 -> [w1297]
                          tunnel: w1292 -> [w1296]
                          tunnel: [w1295] -> w1291
                          i -> [w1300]
                          # "T-wait is 20 ms\nfreq = +-8.3Hz"
                          n1504 = Wait (ms)(milliseconds to wait=20) -> ()  [unwired: 1 out]
                          n1505 = Index Array(array=u8[][] [[0, 0, 0, 0, 0, 0, 0, 0, 2, 4, 3, 3, 3, 3], [0, 0, 0, 0, 0, 0, 0, 0, 0, 0, 0, 0, 0, 0], [0, 0, 0, 0, 0, 0, 0, 0, 0, 0, 0, 0, 0, 0], [0, 0, 0, 0, 0, 0, 0, 0, 0, 0, 0, 0, 0, 0], [0, 0, 0, 0, 0, 0, 0, 0, 0, 0, 0, 0, 0, 0], [11, 11, 11, 11, 11, 11, 11, 0, 0, 0, 0, 0, 0, 0], [0, 0, 0, 0, 0, 0, 0, 0, 0, 0, 0, 0, 0, 0], [16, 16, 16, 16, 16, 16, 16, 0, 0, 0, 0, 0, 0, 0], [0, 0, 0, 0, 0, 0, 0, 0, 0, 0, 0, 0, 0, 0], [0, 0, 0, 0, 0, 0, 0, 0, 0, 0, 0, 0, 0, 0], [0, 0, 0, 0, 0, 0, 0, 0, 0, 0, 0, 0, 0, 0], [2, 2, 2, 2, 2, 2, 2, 0, 0, 0, 0, 0, 0, 0], [4, 4, 4, 4, 4, 4, 4, 0, 0, 0, 0, 0, 0, 0], [255, 255, 255, 255, 255, 255, 0, 0, 0, 0, 0, 0, 0, 0], [3, 2, 6, 4, 5, 1, 0, 0, 0, 0, 0, 0, 0, 0], [27, 27, 27, 27, 27, 27, 0, 0, 0, 0, 0, 0, 0, 0], [255, 255, 255, 255, 255, 255, 0, 0, 0, 0, 0, 0, 0, 0]], index (col)=w1300) -> (element=w1301:u8[])  [unwired: 1 in]
                          n1506 = Byte Array To String(unsigned byte array=w1301) -> (string=w1298:string)
                          n1507 = call "StorePreviousSwitchValues.vi"("Array"=w1301) -> ()  [unwired: 3 in]
                          n1508 = Enqueue Element(queue=w1296, element=w1298, error in (no error)=w1297) -> (error out=w1295:errorcluster)  [unwired: 1 in, 2 out]
                        }
                      }
                      n1509 = Add(x=1, y=w1281) -> (x+y=w1277:i32)
                      n1510 = Less?(x=w1277, y=w1273) -> (x < y?=w1278:bool)
                      n1511 = case shown="True" w1278 {
                        frame False {
                        }
                        frame True {
                          n1512 = local read "Time between Mixing Cycles Initialisation"() -> (w1289:dbl)
                          n1513 = Multiply(x=60000, y=w1289) -> (x*y=w1283:dbl)
                          n1514 = Multiply(x=20, y=500) -> (x*y=w1286:i32)
                          n1515 = Multiply(x=w1286, y=6) -> (x*y=w1285:i32)
                          n1516 = Add(x=w1283, y=w1285) -> (x+y=w1282:dbl)
                          n1517 = Wait (ms)(milliseconds to wait=w1282) -> ()  [unwired: 1 out]
                        }
                      }
                    }
                  }
                  frame #1 {
                    w1306 = u8[] [0, 0, 0, 0, 0, 11, 0, 16, 0, 0, 0, 2, 4, 255, 7, 31, 255]
                    n1518 = call "StorePreviousSwitchValues.vi"("Array"=w1306) -> ()  [unwired: 3 in]
                    n1519 = Byte Array To String(unsigned byte array=w1306) -> (string=w1305:string)
                    n1520 = Enqueue Element(queue=w1303, element=w1305, error in (no error)=w1304) -> ()  [unwired: 1 in, 3 out]
                  }
                  frame #2 {
                    n1521 = global read "CurrentSwitchValues_GlobalVariable.vi" "1"() -> (w1336:bool)
                    n1522 = global read "CurrentSwitchValues_GlobalVariable.vi" "3"() -> (w1329:bool)
                    n1523 = global read "CurrentSwitchValues_GlobalVariable.vi" "5"() -> (w1331:bool)
                    n1524 = global read "CurrentSwitchValues_GlobalVariable.vi" "7"() -> (w1333:bool)
                    n1525 = global read "CurrentSwitchValues_GlobalVariable.vi" "9"() -> (w1321:bool)
                    n1526 = global read "CurrentSwitchValues_GlobalVariable.vi" "11"() -> (w1323:bool)
                    n1527 = global read "CurrentSwitchValues_GlobalVariable.vi" "13"() -> (w1325:bool)
                    n1528 = global read "CurrentSwitchValues_GlobalVariable.vi" "15"() -> (w1327:bool)
                    n1529 = global read "CurrentSwitchValues_GlobalVariable.vi" "17"() -> (w1313:bool)
                    n1530 = global read "CurrentSwitchValues_GlobalVariable.vi" "19"() -> (w1315:bool)
                    n1531 = global read "CurrentSwitchValues_GlobalVariable.vi" "21"() -> (w1317:bool)
                    n1532 = global read "CurrentSwitchValues_GlobalVariable.vi" "23"() -> (w1319:bool)
                    n1533 = global read "CurrentSwitchValues_GlobalVariable.vi" "25"() -> (w1312:bool)
                    n1534 = global read "CurrentSwitchValues_GlobalVariable.vi" "27"() -> (w1310:bool)
                    n1535 = global read "CurrentSwitchValues_GlobalVariable.vi" "29"() -> (w1308:bool)
                    n1536 = global read "CurrentSwitchValues_GlobalVariable.vi" "10"() -> (w1322:bool)
                    n1537 = global read "CurrentSwitchValues_GlobalVariable.vi" "12"() -> (w1324:bool)
                    n1538 = global read "CurrentSwitchValues_GlobalVariable.vi" "14"() -> (w1326:bool)
                    n1539 = global read "CurrentSwitchValues_GlobalVariable.vi" "16"() -> (w1328:bool)
                    n1540 = global read "CurrentSwitchValues_GlobalVariable.vi" "2"() -> (w1335:bool)
                    n1541 = global read "CurrentSwitchValues_GlobalVariable.vi" "6"() -> (w1332:bool)
                    n1542 = global read "CurrentSwitchValues_GlobalVariable.vi" "4"() -> (w1330:bool)
                    n1543 = global read "CurrentSwitchValues_GlobalVariable.vi" "8"() -> (w1334:bool)
                    n1544 = global read "CurrentSwitchValues_GlobalVariable.vi" "18"() -> (w1314:bool)
                    n1545 = global read "CurrentSwitchValues_GlobalVariable.vi" "20"() -> (w1316:bool)
                    n1546 = global read "CurrentSwitchValues_GlobalVariable.vi" "22"() -> (w1318:bool)
                    n1547 = global read "CurrentSwitchValues_GlobalVariable.vi" "24"() -> (w1320:bool)
                    n1548 = global read "CurrentSwitchValues_GlobalVariable.vi" "26"() -> (w1311:bool)
                    n1549 = global read "CurrentSwitchValues_GlobalVariable.vi" "28"() -> (w1309:bool)
                    n1550 = global read "CurrentSwitchValues_GlobalVariable.vi" "30"() -> (w1307:bool)
                    n1551 = property on="1" class="Bool (strict)"("Value"=w1336) -> ()  [unwired: 2 in, 2 out]
                    n1552 = property on="3" class="Bool (strict)"("Value"=w1329) -> ()  [unwired: 2 in, 2 out]
                    n1553 = property on="5" class="Bool (strict)"("Value"=w1331) -> ()  [unwired: 2 in, 2 out]
                    n1554 = property on="7" class="Bool (strict)"("Value"=w1333) -> ()  [unwired: 2 in, 2 out]
                    n1555 = property on="9" class="Bool (strict)"("Value"=w1321) -> ()  [unwired: 2 in, 2 out]
                    n1556 = property on="11" class="Bool (strict)"("Value"=w1323) -> ()  [unwired: 2 in, 2 out]
                    n1557 = property on="13" class="Bool (strict)"("Value"=w1325) -> ()  [unwired: 2 in, 2 out]
                    n1558 = property on="15" class="Bool (strict)"("Value"=w1327) -> ()  [unwired: 2 in, 2 out]
                    n1559 = property on="17" class="Bool (strict)"("Value"=w1313) -> ()  [unwired: 2 in, 2 out]
                    n1560 = property on="19" class="Bool (strict)"("Value"=w1315) -> ()  [unwired: 2 in, 2 out]
                    n1561 = property on="21" class="Bool (strict)"("Value"=w1317) -> ()  [unwired: 2 in, 2 out]
                    n1562 = property on="23" class="Bool (strict)"("Value"=w1319) -> ()  [unwired: 2 in, 2 out]
                    n1563 = property on="25" class="Bool (strict)"("Value"=w1312) -> ()  [unwired: 2 in, 2 out]
                    n1564 = property on="27" class="Bool (strict)"("Value"=w1310) -> ()  [unwired: 2 in, 2 out]
                    n1565 = property on="29" class="Bool (strict)"("Value"=w1308) -> ()  [unwired: 2 in, 2 out]
                    n1566 = property on="26" class="Bool (strict)"("Value"=w1311) -> ()  [unwired: 2 in, 2 out]
                    n1567 = property on="28" class="Bool (strict)"("Value"=w1309) -> ()  [unwired: 2 in, 2 out]
                    n1568 = property on="30" class="Bool (strict)"("Value"=w1307) -> ()  [unwired: 2 in, 2 out]
                    n1569 = property on="2" class="Bool (strict)"("Value"=w1335) -> ()  [unwired: 2 in, 2 out]
                    n1570 = property on="4" class="Bool (strict)"("Value"=w1330) -> ()  [unwired: 2 in, 2 out]
                    n1571 = property on="6" class="Bool (strict)"("Value"=w1332) -> ()  [unwired: 2 in, 2 out]
                    n1572 = property on="8" class="Bool (strict)"("Value"=w1334) -> ()  [unwired: 2 in, 2 out]
                    n1573 = property on="10" class="Bool (strict)"("Value"=w1322) -> ()  [unwired: 2 in, 2 out]
                    n1574 = property on="12" class="Bool (strict)"("Value"=w1324) -> ()  [unwired: 2 in, 2 out]
                    n1575 = property on="14" class="Bool (strict)"("Value"=w1326) -> ()  [unwired: 2 in, 2 out]
                    n1576 = property on="16" class="Bool (strict)"("Value"=w1328) -> ()  [unwired: 2 in, 2 out]
                    n1577 = property on="18" class="Bool (strict)"("Value"=w1314) -> ()  [unwired: 2 in, 2 out]
                    n1578 = property on="20" class="Bool (strict)"("Value"=w1316) -> ()  [unwired: 2 in, 2 out]
                    n1579 = property on="22" class="Bool (strict)"("Value"=w1318) -> ()  [unwired: 2 in, 2 out]
                    n1580 = property on="24" class="Bool (strict)"("Value"=w1320) -> ()  [unwired: 2 in, 2 out]
                  }
                }
              }
              frame #7 {
                # "Here we begin with the actual experiment, performing periodic dilutions \n(ever 15 minutes) and imaging the increase in the protein concentration \nusing the fluorescence measurements. \n\nWithin this portion of the process the following steps will be performed:\n8.1 - Image\n8.2 - Flush FB\n8.3 - Load FB (All reactors)\n8.4 - Flush DNA\n8.5 - Load DNA (Reactors 2-7)\n8.6 - Flush EB\n8.7 - Load EB (Reactors 1 and 8)\n8.8 - Mix ( min)"
                n1581 = for {
                  N: "Number of Dilution Cycles" -> [_]
                  tunnel: w1338 -> [w1341]
                  tunnel: w1337 -> [w1340]
                  n1582 = stacked-sequence {
                    tunnel: w1341 -> [_ w1348 w1375 w1406 w1437 w1468 w1499 w1530 w1561 w1592 w1613 w1639 w1670 w1701 w1732 w1763 w1794 w1814 w1841 w1872 w1893 w1924 _]
                    tunnel: w1340 -> [_ w1347 w1374 w1405 w1436 w1467 w1498 w1529 w1560 w1591 w1612 w1638 w1669 w1700 w1731 w1762 w1793 w1813 w1840 w1871 w1892 w1925 _]
                    tunnel: [_ w1346 _ _ _ _ _ _ _ _ _ _ _ _ _ _ _ _ _ _ _ _ _] -> _
                    frame #0 {
                      # "Step 1: Imaging. Occurs directly after mixing."
                      n1583 = flat-sequence {
                        frame #0 {
                          n1584 = call <vilib>:"System Exec.vi"("command line"="C:\\Users\\avdlinde\\Desktop\\Labview Interface for Jove Paper\\dummy_sender.exe") -> ()  [unwired: 7 in, 4 out]
                        }
                        frame #1 {
                          n1585 = call <vilib>:"System Exec.vi"("wait until completion? (T)"=TRUE, "command line"="Replace with Checking Executable") -> ()  [unwired: 6 in, 4 out]
                        }
                        frame #2 {
                          # "Waiting step will ensure that \nthe program does not record \ntwo sets of images at one time\npoint due errors regarding the \nsending of messages."
                          n1586 = Wait (ms)(milliseconds to wait=30000) -> ()  [unwired: 1 out]
                        }
                      }
                    }
                    frame #1 {
                      # "Step 8.2: \nFlush FB"
                      n1587 = for {
                        N: 100 -> [_]
                        tunnel: w1348 -> [w1352]
                        tunnel: w1347 -> [w1351]
                        tunnel: [w1350] -> w1346
                        n1588 = for {
                          N: 6 -> [_]
                          tunnel: w1352 -> [w1357]
                          tunnel: w1351 -> [w1356]
                          tunnel: [w1355] -> w1350
                          i -> [w1361]
                          # "T-wait is 100 ms,\nfreq = +-1.7Hz if fast and T-wait is 556ms, freq = 0.3Hz if slow flush."
                          n1589 = local read "FB"() -> (w1354:dbl)
                          n1590 = call "SequenceSelector_Flush.vi"("Inflow Channel Selector"=w1354) -> ("Array"=w1360:u8[][])
                          n1591 = Wait (ms)(milliseconds to wait=50) -> ()  [unwired: 1 out]
                          n1592 = Index Array(array=w1360, index (col)=w1361) -> (element=w1362:u8[])  [unwired: 1 in]
                          n1593 = call "StorePreviousSwitchValues.vi"("Array"=w1362) -> ()  [unwired: 3 in]
                          n1594 = Byte Array To String(unsigned byte array=w1362) -> (string=w1358:string)
                          n1595 = Enqueue Element(queue=w1356, element=w1358, error in (no error)=w1357) -> (error out=w1355:errorcluster)  [unwired: 1 in, 2 out]
                        }
                      }
                    }
                    frame #2 {
                      w1366 = 1
                      # "Step 8.3:\nLoad FB"
                      n1596 = local read "Refresh Fraction [%]"() -> (w1363:dbl)
                      n1597 = local read "FB RR"() -> (w1371:dbl)
                      n1598 = Subtract(x=w1366, y=1) -> (x-y=w1364:i32)
                      n1599 = global write "CurrentSwitchValues_GlobalVariable.vi" "Current Reactor"(w1366) -> ()
                      n1600 = Divide(x=100, y=w1363) -> (x/y=w1368:dbl)
                      n1601 = call "ConvertDesiredRefreshRatioPerReactor.vi"("Desired Refresh Ratio"=w1371, "Reactor"=w1364) -> ("Required Number of Pump Iterations"=w1372:dbl)
                      n1602 = Round To Nearest(number=w1368) -> (nearest integer value=w1367:dbl)
                      n1603 = Divide(x=w1372, y=w1367) -> (x/y=w1373:dbl)
                      n1604 = Round To Nearest(number=w1373) -> (nearest integer value=w1370:dbl)
                      n1605 = for {
                        N: w1370 -> [_]
                        tunnel: [w1380] -> _
                        tunnel: w1375 -> [w1377]
                        tunnel: w1374 -> [w1376]
                        i -> [w1378]
                        n1606 = for {
                          N: 6 -> [_]
                          tunnel: [w1393] -> w1380
                          tunnel: w1378 -> [w1386]
                          tunnel: w1377 -> [w1389]
                          tunnel: w1376 -> [w1388]
                          i -> [w1390]
                          w1381 = TRUE
                          w1382 = TRUE
                          n1607 = global read "CurrentSwitchValues_GlobalVariable.vi" "Current Reactor"() -> (w1384:dbl)
                          n1608 = local read "FB"() -> (w1383:dbl)
                          n1609 = call "SequenceSelector_LoadPerReactor.vi"("Reactor 6"=w1381, "Reactor 7"=w1381, "Reactor 8"=w1382, "Loop Iteration"=w1386, "Reactor 5"=w1381, "Reactor 4"=w1381, "Current Reactor"=w1384, "Reactor 3"=w1381, "Reactor 2"=w1381, "Reactor 1"=w1382, "Inflow Channel Selector"=w1383) -> ("Array"=w1387:u8[][])
                          n1610 = Index Array(array=w1387, index (col)=w1390) -> (element=w1385:u8[])  [unwired: 1 in]
                          n1611 = Byte Array To String(unsigned byte array=w1385) -> (string=w1391:string)
                          n1612 = Enqueue Element(queue=w1388, element=w1391, error in (no error)=w1389) -> (error out=w1393:errorcluster)  [unwired: 1 in, 2 out]
                          n1613 = call "StorePreviousSwitchValues.vi"("Array"=w1385) -> ()  [unwired: 3 in]
                          n1614 = Wait (ms)(milliseconds to wait=15) -> ()  [unwired: 1 out]
                        }
                      }
                    }
                    frame #3 {
                      w1397 = 2
                      # "Step 8.3:\nLoad FB"
                      n1615 = local read "Refresh Fraction [%]"() -> (w1394:dbl)
                      n1616 = local read "FB RR"() -> (w1402:dbl)
                      n1617 = Subtract(x=w1397, y=1) -> (x-y=w1395:i32)
                      n1618 = global write "CurrentSwitchValues_GlobalVariable.vi" "Current Reactor"(w1397) -> ()
                      n1619 = Divide(x=100, y=w1394) -> (x/y=w1399:dbl)
                      n1620 = call "ConvertDesiredRefreshRatioPerReactor.vi"("Desired Refresh Ratio"=w1402, "Reactor"=w1395) -> ("Required Number of Pump Iterations"=w1403:dbl)
                      n1621 = Round To Nearest(number=w1399) -> (nearest integer value=w1398:dbl)
                      n1622 = Divide(x=w1403, y=w1398) -> (x/y=w1404:dbl)
                      n1623 = Round To Nearest(number=w1404) -> (nearest integer value=w1401:dbl)
                      n1624 = for {
                        N: w1401 -> [_]
                        tunnel: [w1411] -> _
                        tunnel: w1406 -> [w1408]
                        tunnel: w1405 -> [w1407]
                        i -> [w1409]
                        n1625 = for {
                          N: 6 -> [_]
                          tunnel: [w1424] -> w1411
                          tunnel: w1409 -> [w1417]
                          tunnel: w1408 -> [w1420]
                          tunnel: w1407 -> [w1419]
                          i -> [w1421]
                          w1412 = TRUE
                          w1413 = TRUE
                          n1626 = global read "CurrentSwitchValues_GlobalVariable.vi" "Current Reactor"() -> (w1415:dbl)
                          n1627 = local read "FB"() -> (w1414:dbl)
                          n1628 = call "SequenceSelector_LoadPerReactor.vi"("Reactor 6"=w1412, "Reactor 7"=w1412, "Reactor 8"=w1413, "Loop Iteration"=w1417, "Reactor 5"=w1412, "Reactor 4"=w1412, "Current Reactor"=w1415, "Reactor 3"=w1412, "Reactor 2"=w1412, "Reactor 1"=w1413, "Inflow Channel Selector"=w1414) -> ("Array"=w1418:u8[][])
                          n1629 = Index Array(array=w1418, index (col)=w1421) -> (element=w1416:u8[])  [unwired: 1 in]
                          n1630 = Byte Array To String(unsigned byte array=w1416) -> (string=w1422:string)
                          n1631 = Enqueue Element(queue=w1419, element=w1422, error in (no error)=w1420) -> (error out=w1424:errorcluster)  [unwired: 1 in, 2 out]
                          n1632 = call "StorePreviousSwitchValues.vi"("Array"=w1416) -> ()  [unwired: 3 in]
                          n1633 = Wait (ms)(milliseconds to wait=15) -> ()  [unwired: 1 out]
                        }
                      }
                    }
                    frame #4 {
                      w1428 = 3
                      # "Step 8.3:\nLoad FB"
                      n1634 = local read "Refresh Fraction [%]"() -> (w1425:dbl)
                      n1635 = local read "FB RR"() -> (w1433:dbl)
                      n1636 = Subtract(x=w1428, y=1) -> (x-y=w1426:i32)
                      n1637 = global write "CurrentSwitchValues_GlobalVariable.vi" "Current Reactor"(w1428) -> ()
                      n1638 = Divide(x=100, y=w1425) -> (x/y=w1430:dbl)
                      n1639 = call "ConvertDesiredRefreshRatioPerReactor.vi"("Desired Refresh Ratio"=w1433, "Reactor"=w1426) -> ("Required Number of Pump Iterations"=w1434:dbl)
                      n1640 = Round To Nearest(number=w1430) -> (nearest integer value=w1429:dbl)
                      n1641 = Divide(x=w1434, y=w1429) -> (x/y=w1435:dbl)
                      n1642 = Round To Nearest(number=w1435) -> (nearest integer value=w1432:dbl)
                      n1643 = for {
                        N: w1432 -> [_]
                        tunnel: [w1442] -> _
                        tunnel: w1437 -> [w1439]
                        tunnel: w1436 -> [w1438]
                        i -> [w1440]
                        n1644 = for {
                          N: 6 -> [_]
                          tunnel: [w1455] -> w1442
                          tunnel: w1440 -> [w1448]
                          tunnel: w1439 -> [w1451]
                          tunnel: w1438 -> [w1450]
                          i -> [w1452]
                          w1443 = TRUE
                          w1444 = TRUE
                          n1645 = global read "CurrentSwitchValues_GlobalVariable.vi" "Current Reactor"() -> (w1446:dbl)
                          n1646 = local read "FB"() -> (w1445:dbl)
                          n1647 = call "SequenceSelector_LoadPerReactor.vi"("Reactor 6"=w1443, "Reactor 7"=w1443, "Reactor 8"=w1444, "Loop Iteration"=w1448, "Reactor 5"=w1443, "Reactor 4"=w1443, "Current Reactor"=w1446, "Reactor 3"=w1443, "Reactor 2"=w1443, "Reactor 1"=w1444, "Inflow Channel Selector"=w1445) -> ("Array"=w1449:u8[][])
                          n1648 = Index Array(array=w1449, index (col)=w1452) -> (element=w1447:u8[])  [unwired: 1 in]
                          n1649 = Byte Array To String(unsigned byte array=w1447) -> (string=w1453:string)
                          n1650 = Enqueue Element(queue=w1450, element=w1453, error in (no error)=w1451) -> (error out=w1455:errorcluster)  [unwired: 1 in, 2 out]
                          n1651 = call "StorePreviousSwitchValues.vi"("Array"=w1447) -> ()  [unwired: 3 in]
                          n1652 = Wait (ms)(milliseconds to wait=15) -> ()  [unwired: 1 out]
                        }
                      }
                    }
                    frame #5 {
                      w1459 = 4
                      # "Step 8.3:\nLoad FB"
                      n1653 = local read "Refresh Fraction [%]"() -> (w1456:dbl)
                      n1654 = local read "FB RR"() -> (w1464:dbl)
                      n1655 = Subtract(x=w1459, y=1) -> (x-y=w1457:i32)
                      n1656 = global write "CurrentSwitchValues_GlobalVariable.vi" "Current Reactor"(w1459) -> ()
                      n1657 = Divide(x=100, y=w1456) -> (x/y=w1461:dbl)
                      n1658 = call "ConvertDesiredRefreshRatioPerReactor.vi"("Desired Refresh Ratio"=w1464, "Reactor"=w1457) -> ("Required Number of Pump Iterations"=w1465:dbl)
                      n1659 = Round To Nearest(number=w1461) -> (nearest integer value=w1460:dbl)
                      n1660 = Divide(x=w1465, y=w1460) -> (x/y=w1466:dbl)
                      n1661 = Round To Nearest(number=w1466) -> (nearest integer value=w1463:dbl)
                      n1662 = for {
                        N: w1463 -> [_]
                        tunnel: [w1473] -> _
                        tunnel: w1468 -> [w1470]
                        tunnel: w1467 -> [w1469]
                        i -> [w1471]
                        n1663 = for {
                          N: 6 -> [_]
                          tunnel: [w1486] -> w1473
                          tunnel: w1471 -> [w1479]
                          tunnel: w1470 -> [w1482]
                          tunnel: w1469 -> [w1481]
                          i -> [w1483]
                          w1474 = TRUE
                          w1475 = TRUE
                          n1664 = global read "CurrentSwitchValues_GlobalVariable.vi" "Current Reactor"() -> (w1477:dbl)
                          n1665 = local read "FB"() -> (w1476:dbl)
                          n1666 = call "SequenceSelector_LoadPerReactor.vi"("Reactor 6"=w1474, "Reactor 7"=w1474, "Reactor 8"=w1475, "Loop Iteration"=w1479, "Reactor 5"=w1474, "Reactor 4"=w1474, "Current Reactor"=w1477, "Reactor 3"=w1474, "Reactor 2"=w1474, "Reactor 1"=w1475, "Inflow Channel Selector"=w1476) -> ("Array"=w1480:u8[][])
                          n1667 = Index Array(array=w1480, index (col)=w1483) -> (element=w1478:u8[])  [unwired: 1 in]
                          n1668 = Byte Array To String(unsigned byte array=w1478) -> (string=w1484:string)
                          n1669 = Enqueue Element(queue=w1481, element=w1484, error in (no error)=w1482) -> (error out=w1486:errorcluster)  [unwired: 1 in, 2 out]
                          n1670 = call "StorePreviousSwitchValues.vi"("Array"=w1478) -> ()  [unwired: 3 in]
                          n1671 = Wait (ms)(milliseconds to wait=15) -> ()  [unwired: 1 out]
                        }
                      }
                    }
                    frame #6 {
                      w1490 = 5
                      # "Step 8.3:\nLoad FB"
                      n1672 = local read "Refresh Fraction [%]"() -> (w1487:dbl)
                      n1673 = local read "FB RR"() -> (w1495:dbl)
                      n1674 = Subtract(x=w1490, y=1) -> (x-y=w1488:i32)
                      n1675 = global write "CurrentSwitchValues_GlobalVariable.vi" "Current Reactor"(w1490) -> ()
                      n1676 = Divide(x=100, y=w1487) -> (x/y=w1492:dbl)
                      n1677 = call "ConvertDesiredRefreshRatioPerReactor.vi"("Desired Refresh Ratio"=w1495, "Reactor"=w1488) -> ("Required Number of Pump Iterations"=w1496:dbl)
                      n1678 = Round To Nearest(number=w1492) -> (nearest integer value=w1491:dbl)
                      n1679 = Divide(x=w1496, y=w1491) -> (x/y=w1497:dbl)
                      n1680 = Round To Nearest(number=w1497) -> (nearest integer value=w1494:dbl)
                      n1681 = for {
                        N: w1494 -> [_]
                        tunnel: [w1504] -> _
                        tunnel: w1499 -> [w1501]
                        tunnel: w1498 -> [w1500]
                        i -> [w1502]
                        n1682 = for {
                          N: 6 -> [_]
                          tunnel: [w1517] -> w1504
                          tunnel: w1502 -> [w1510]
                          tunnel: w1501 -> [w1513]
                          tunnel: w1500 -> [w1512]
                          i -> [w1514]
                          w1505 = TRUE
                          w1506 = TRUE
                          n1683 = global read "CurrentSwitchValues_GlobalVariable.vi" "Current Reactor"() -> (w1508:dbl)
                          n1684 = local read "FB"() -> (w1507:dbl)
                          n1685 = call "SequenceSelector_LoadPerReactor.vi"("Reactor 6"=w1505, "Reactor 7"=w1505, "Reactor 8"=w1506, "Loop Iteration"=w1510, "Reactor 5"=w1505, "Reactor 4"=w1505, "Current Reactor"=w1508, "Reactor 3"=w1505, "Reactor 2"=w1505, "Reactor 1"=w1506, "Inflow Channel Selector"=w1507) -> ("Array"=w1511:u8[][])
                          n1686 = Index Array(array=w1511, index (col)=w1514) -> (element=w1509:u8[])  [unwired: 1 in]
                          n1687 = Byte Array To String(unsigned byte array=w1509) -> (string=w1515:string)
                          n1688 = Enqueue Element(queue=w1512, element=w1515, error in (no error)=w1513) -> (error out=w1517:errorcluster)  [unwired: 1 in, 2 out]
                          n1689 = call "StorePreviousSwitchValues.vi"("Array"=w1509) -> ()  [unwired: 3 in]
                          n1690 = Wait (ms)(milliseconds to wait=15) -> ()  [unwired: 1 out]
                        }
                      }
                    }
                    frame #7 {
                      w1521 = 6
                      # "Step 8.3:\nLoad FB"
                      n1691 = local read "Refresh Fraction [%]"() -> (w1518:dbl)
                      n1692 = local read "FB RR"() -> (w1526:dbl)
                      n1693 = Subtract(x=w1521, y=1) -> (x-y=w1519:i32)
                      n1694 = global write "CurrentSwitchValues_GlobalVariable.vi" "Current Reactor"(w1521) -> ()
                      n1695 = Divide(x=100, y=w1518) -> (x/y=w1523:dbl)
                      n1696 = call "ConvertDesiredRefreshRatioPerReactor.vi"("Desired Refresh Ratio"=w1526, "Reactor"=w1519) -> ("Required Number of Pump Iterations"=w1527:dbl)
                      n1697 = Round To Nearest(number=w1523) -> (nearest integer value=w1522:dbl)
                      n1698 = Divide(x=w1527, y=w1522) -> (x/y=w1528:dbl)
                      n1699 = Round To Nearest(number=w1528) -> (nearest integer value=w1525:dbl)
                      n1700 = for {
                        N: w1525 -> [_]
                        tunnel: [w1535] -> _
                        tunnel: w1530 -> [w1532]
                        tunnel: w1529 -> [w1531]
                        i -> [w1533]
                        n1701 = for {
                          N: 6 -> [_]
                          tunnel: [w1548] -> w1535
                          tunnel: w1533 -> [w1541]
                          tunnel: w1532 -> [w1544]
                          tunnel: w1531 -> [w1543]
                          i -> [w1545]
                          w1536 = TRUE
                          w1537 = TRUE
                          n1702 = global read "CurrentSwitchValues_GlobalVariable.vi" "Current Reactor"() -> (w1539:dbl)
                          n1703 = local read "FB"() -> (w1538:dbl)
                          n1704 = call "SequenceSelector_LoadPerReactor.vi"("Reactor 6"=w1536, "Reactor 7"=w1536, "Reactor 8"=w1537, "Loop Iteration"=w1541, "Reactor 5"=w1536, "Reactor 4"=w1536, "Current Reactor"=w1539, "Reactor 3"=w1536, "Reactor 2"=w1536, "Reactor 1"=w1537, "Inflow Channel Selector"=w1538) -> ("Array"=w1542:u8[][])
                          n1705 = Index Array(array=w1542, index (col)=w1545) -> (element=w1540:u8[])  [unwired: 1 in]
                          n1706 = Byte Array To String(unsigned byte array=w1540) -> (string=w1546:string)
                          n1707 = Enqueue Element(queue=w1543, element=w1546, error in (no error)=w1544) -> (error out=w1548:errorcluster)  [unwired: 1 in, 2 out]
                          n1708 = call "StorePreviousSwitchValues.vi"("Array"=w1540) -> ()  [unwired: 3 in]
                          n1709 = Wait (ms)(milliseconds to wait=15) -> ()  [unwired: 1 out]
                        }
                      }
                    }
                    frame #8 {
                      w1552 = 7
                      # "Step 8.3:\nLoad FB"
                      n1710 = local read "Refresh Fraction [%]"() -> (w1549:dbl)
                      n1711 = local read "FB RR"() -> (w1557:dbl)
                      n1712 = Subtract(x=w1552, y=1) -> (x-y=w1550:i32)
                      n1713 = global write "CurrentSwitchValues_GlobalVariable.vi" "Current Reactor"(w1552) -> ()
                      n1714 = Divide(x=100, y=w1549) -> (x/y=w1554:dbl)
                      n1715 = call "ConvertDesiredRefreshRatioPerReactor.vi"("Desired Refresh Ratio"=w1557, "Reactor"=w1550) -> ("Required Number of Pump Iterations"=w1558:dbl)
                      n1716 = Round To Nearest(number=w1554) -> (nearest integer value=w1553:dbl)
                      n1717 = Divide(x=w1558, y=w1553) -> (x/y=w1559:dbl)
                      n1718 = Round To Nearest(number=w1559) -> (nearest integer value=w1556:dbl)
                      n1719 = for {
                        N: w1556 -> [_]
                        tunnel: [w1566] -> _
                        tunnel: w1561 -> [w1563]
                        tunnel: w1560 -> [w1562]
                        i -> [w1564]
                        n1720 = for {
                          N: 6 -> [_]
                          tunnel: [w1579] -> w1566
                          tunnel: w1564 -> [w1572]
                          tunnel: w1563 -> [w1575]
                          tunnel: w1562 -> [w1574]
                          i -> [w1576]
                          w1567 = TRUE
                          w1568 = TRUE
                          n1721 = global read "CurrentSwitchValues_GlobalVariable.vi" "Current Reactor"() -> (w1570:dbl)
                          n1722 = local read "FB"() -> (w1569:dbl)
                          n1723 = call "SequenceSelector_LoadPerReactor.vi"("Reactor 6"=w1567, "Reactor 7"=w1567, "Reactor 8"=w1568, "Loop Iteration"=w1572, "Reactor 5"=w1567, "Reactor 4"=w1567, "Current Reactor"=w1570, "Reactor 3"=w1567, "Reactor 2"=w1567, "Reactor 1"=w1568, "Inflow Channel Selector"=w1569) -> ("Array"=w1573:u8[][])
                          n1724 = Index Array(array=w1573, index (col)=w1576) -> (element=w1571:u8[])  [unwired: 1 in]
                          n1725 = Byte Array To String(unsigned byte array=w1571) -> (string=w1577:string)
                          n1726 = Enqueue Element(queue=w1574, element=w1577, error in (no error)=w1575) -> (error out=w1579:errorcluster)  [unwired: 1 in, 2 out]
                          n1727 = call "StorePreviousSwitchValues.vi"("Array"=w1571) -> ()  [unwired: 3 in]
                          n1728 = Wait (ms)(milliseconds to wait=15) -> ()  [unwired: 1 out]
                        }
                      }
                    }
                    frame #9 {
                      w1583 = 8
                      # "Step 8.3:\nLoad FB"
                      n1729 = local read "Refresh Fraction [%]"() -> (w1580:dbl)
                      n1730 = local read "FB RR"() -> (w1588:dbl)
                      n1731 = Subtract(x=w1583, y=1) -> (x-y=w1581:i32)
                      n1732 = global write "CurrentSwitchValues_GlobalVariable.vi" "Current Reactor"(w1583) -> ()
                      n1733 = Divide(x=100, y=w1580) -> (x/y=w1585:dbl)
                      n1734 = call "ConvertDesiredRefreshRatioPerReactor.vi"("Desired Refresh Ratio"=w1588, "Reactor"=w1581) -> ("Required Number of Pump Iterations"=w1589:dbl)
                      n1735 = Round To Nearest(number=w1585) -> (nearest integer value=w1584:dbl)
                      n1736 = Divide(x=w1589, y=w1584) -> (x/y=w1590:dbl)
                      n1737 = Round To Nearest(number=w1590) -> (nearest integer value=w1587:dbl)
                      n1738 = for {
                        N: w1587 -> [_]
                        tunnel: [w1597] -> _
                        tunnel: w1592 -> [w1594]
                        tunnel: w1591 -> [w1593]
                        i -> [w1595]
                        n1739 = for {
                          N: 6 -> [_]
                          tunnel: [w1610] -> w1597
                          tunnel: w1595 -> [w1603]
                          tunnel: w1594 -> [w1606]
                          tunnel: w1593 -> [w1605]
                          i -> [w1607]
                          w1598 = TRUE
                          w1599 = TRUE
                          n1740 = global read "CurrentSwitchValues_GlobalVariable.vi" "Current Reactor"() -> (w1601:dbl)
                          n1741 = local read "FB"() -> (w1600:dbl)
                          n1742 = call "SequenceSelector_LoadPerReactor.vi"("Reactor 6"=w1598, "Reactor 7"=w1598, "Reactor 8"=w1599, "Loop Iteration"=w1603, "Reactor 5"=w1598, "Reactor 4"=w1598, "Current Reactor"=w1601, "Reactor 3"=w1598, "Reactor 2"=w1598, "Reactor 1"=w1599, "Inflow Channel Selector"=w1600) -> ("Array"=w1604:u8[][])
                          n1743 = Index Array(array=w1604, index (col)=w1607) -> (element=w1602:u8[])  [unwired: 1 in]
                          n1744 = Byte Array To String(unsigned byte array=w1602) -> (string=w1608:string)
                          n1745 = Enqueue Element(queue=w1605, element=w1608, error in (no error)=w1606) -> (error out=w1610:errorcluster)  [unwired: 1 in, 2 out]
                          n1746 = call "StorePreviousSwitchValues.vi"("Array"=w1602) -> ()  [unwired: 3 in]
                          n1747 = Wait (ms)(milliseconds to wait=15) -> ()  [unwired: 1 out]
                        }
                      }
                    }
                    frame #10 {
                      # "Step 8.4: \nFlush DNA"
                      n1748 = for {
                        N: 100 -> [_]
                        tunnel: w1613 -> [w1616]
                        tunnel: w1612 -> [w1615]
                        tunnel: [w1614] -> _
                        n1749 = for {
                          N: 6 -> [_]
                          tunnel: w1616 -> [w1621]
                          tunnel: w1615 -> [w1620]
                          tunnel: [w1619] -> w1614
                          i -> [w1625]
                          # "T-wait is 100 ms,\nfreq = +-1.7Hz if fast and T-wait is 556ms, freq = 0.3Hz if slow flush."
                          n1750 = local read "DNA Channel"() -> (w1618:dbl)
                          n1751 = call "SequenceSelector_Flush.vi"("Inflow Channel Selector"=w1618) -> ("Array"=w1624:u8[][])
                          n1752 = Wait (ms)(milliseconds to wait=50) -> ()  [unwired: 1 out]
                          n1753 = Index Array(array=w1624, index (col)=w1625) -> (element=w1626:u8[])  [unwired: 1 in]
                          n1754 = call "StorePreviousSwitchValues.vi"("Array"=w1626) -> ()  [unwired: 3 in]
                          n1755 = Byte Array To String(unsigned byte array=w1626) -> (string=w1622:string)
                          n1756 = Enqueue Element(queue=w1620, element=w1622, error in (no error)=w1621) -> (error out=w1619:errorcluster)  [unwired: 1 in, 2 out]
                        }
                      }
                    }
                    frame #11 {
                      w1630 = 2
                      # "Step 8.5:\nLoad DNA"
                      n1757 = local read "Refresh Fraction [%]"() -> (w1627:dbl)
                      n1758 = local read "DNA  High RR"() -> (w1635:dbl)
                      n1759 = Subtract(x=w1630, y=1) -> (x-y=w1628:i32)
                      n1760 = global write "CurrentSwitchValues_GlobalVariable.vi" "Current Reactor"(w1630) -> ()
                      n1761 = Divide(x=100, y=w1627) -> (x/y=w1632:dbl)
                      n1762 = call "ConvertDesiredRefreshRatioPerReactor.vi"("Desired Refresh Ratio"=w1635, "Reactor"=w1628) -> ("Required Number of Pump Iterations"=w1636:dbl)
                      n1763 = Round To Nearest(number=w1632) -> (nearest integer value=w1631:dbl)
                      n1764 = Divide(x=w1636, y=w1631) -> (x/y=w1637:dbl)
                      n1765 = Round To Nearest(number=w1637) -> (nearest integer value=w1634:dbl)
                      n1766 = for {
                        N: w1634 -> [_]
                        tunnel: [w1644] -> _
                        tunnel: w1639 -> [w1641]
                        tunnel: w1638 -> [w1640]
                        i -> [w1642]
                        n1767 = for {
                          N: 6 -> [_]
                          tunnel: [w1657] -> w1644
                          tunnel: w1642 -> [w1650]
                          tunnel: w1641 -> [w1653]
                          tunnel: w1640 -> [w1652]
                          i -> [w1654]
                          w1645 = TRUE
                          w1646 = TRUE
                          n1768 = global read "CurrentSwitchValues_GlobalVariable.vi" "Current Reactor"() -> (w1648:dbl)
                          n1769 = local read "DNA Channel"() -> (w1647:dbl)
                          n1770 = call "SequenceSelector_LoadPerReactor.vi"("Reactor 6"=w1645, "Reactor 7"=w1645, "Reactor 8"=w1646, "Loop Iteration"=w1650, "Reactor 5"=w1645, "Reactor 4"=w1645, "Current Reactor"=w1648, "Reactor 3"=w1645, "Reactor 2"=w1645, "Reactor 1"=w1646, "Inflow Channel Selector"=w1647) -> ("Array"=w1651:u8[][])
                          n1771 = Index Array(array=w1651, index (col)=w1654) -> (element=w1649:u8[])  [unwired: 1 in]
                          n1772 = Byte Array To String(unsigned byte array=w1649) -> (string=w1655:string)
                          n1773 = Enqueue Element(queue=w1652, element=w1655, error in (no error)=w1653) -> (error out=w1657:errorcluster)  [unwired: 1 in, 2 out]
                          n1774 = call "StorePreviousSwitchValues.vi"("Array"=w1649) -> ()  [unwired: 3 in]
                          n1775 = Wait (ms)(milliseconds to wait=15) -> ()  [unwired: 1 out]
                        }
                      }
                    }
                    frame #12 {
                      w1661 = 3
                      # "Step 8.5:\nLoad DNA"
                      n1776 = local read "Refresh Fraction [%]"() -> (w1658:dbl)
                      n1777 = local read "DNA  High RR"() -> (w1666:dbl)
                      n1778 = Subtract(x=w1661, y=1) -> (x-y=w1659:i32)
                      n1779 = global write "CurrentSwitchValues_GlobalVariable.vi" "Current Reactor"(w1661) -> ()
                      n1780 = Divide(x=100, y=w1658) -> (x/y=w1663:dbl)
                      n1781 = call "ConvertDesiredRefreshRatioPerReactor.vi"("Desired Refresh Ratio"=w1666, "Reactor"=w1659) -> ("Required Number of Pump Iterations"=w1667:dbl)
                      n1782 = Round To Nearest(number=w1663) -> (nearest integer value=w1662:dbl)
                      n1783 = Divide(x=w1667, y=w1662) -> (x/y=w1668:dbl)
                      n1784 = Round To Nearest(number=w1668) -> (nearest integer value=w1665:dbl)
                      n1785 = for {
                        N: w1665 -> [_]
                        tunnel: [w1675] -> _
                        tunnel: w1670 -> [w1672]
                        tunnel: w1669 -> [w1671]
                        i -> [w1673]
                        n1786 = for {
                          N: 6 -> [_]
                          tunnel: [w1688] -> w1675
                          tunnel: w1673 -> [w1681]
                          tunnel: w1672 -> [w1684]
                          tunnel: w1671 -> [w1683]
                          i -> [w1685]
                          w1676 = TRUE
                          w1677 = TRUE
                          n1787 = global read "CurrentSwitchValues_GlobalVariable.vi" "Current Reactor"() -> (w1679:dbl)
                          n1788 = local read "DNA Channel"() -> (w1678:dbl)
                          n1789 = call "SequenceSelector_LoadPerReactor.vi"("Reactor 6"=w1676, "Reactor 7"=w1676, "Reactor 8"=w1677, "Loop Iteration"=w1681, "Reactor 5"=w1676, "Reactor 4"=w1676, "Current Reactor"=w1679, "Reactor 3"=w1676, "Reactor 2"=w1676, "Reactor 1"=w1677, "Inflow Channel Selector"=w1678) -> ("Array"=w1682:u8[][])
                          n1790 = Index Array(array=w1682, index (col)=w1685) -> (element=w1680:u8[])  [unwired: 1 in]
                          n1791 = Byte Array To String(unsigned byte array=w1680) -> (string=w1686:string)
                          n1792 = Enqueue Element(queue=w1683, element=w1686, error in (no error)=w1684) -> (error out=w1688:errorcluster)  [unwired: 1 in, 2 out]
                          n1793 = call "StorePreviousSwitchValues.vi"("Array"=w1680) -> ()  [unwired: 3 in]
                          n1794 = Wait (ms)(milliseconds to wait=15) -> ()  [unwired: 1 out]
                        }
                      }
                    }
                    frame #13 {
                      w1692 = 4
                      # "Step 8.5:\nLoad DNA"
                      n1795 = local read "Refresh Fraction [%]"() -> (w1689:dbl)
                      n1796 = local read "DNA  High RR"() -> (w1697:dbl)
                      n1797 = Subtract(x=w1692, y=1) -> (x-y=w1690:i32)
                      n1798 = global write "CurrentSwitchValues_GlobalVariable.vi" "Current Reactor"(w1692) -> ()
                      n1799 = Divide(x=100, y=w1689) -> (x/y=w1694:dbl)
                      n1800 = call "ConvertDesiredRefreshRatioPerReactor.vi"("Desired Refresh Ratio"=w1697, "Reactor"=w1690) -> ("Required Number of Pump Iterations"=w1698:dbl)
                      n1801 = Round To Nearest(number=w1694) -> (nearest integer value=w1693:dbl)
                      n1802 = Divide(x=w1698, y=w1693) -> (x/y=w1699:dbl)
                      n1803 = Round To Nearest(number=w1699) -> (nearest integer value=w1696:dbl)
                      n1804 = for {
                        N: w1696 -> [_]
                        tunnel: [w1706] -> _
                        tunnel: w1701 -> [w1703]
                        tunnel: w1700 -> [w1702]
                        i -> [w1704]
                        n1805 = for {
                          N: 6 -> [_]
                          tunnel: [w1719] -> w1706
                          tunnel: w1704 -> [w1712]
                          tunnel: w1703 -> [w1715]
                          tunnel: w1702 -> [w1714]
                          i -> [w1716]
                          w1707 = TRUE
                          w1708 = TRUE
                          n1806 = global read "CurrentSwitchValues_GlobalVariable.vi" "Current Reactor"() -> (w1710:dbl)
                          n1807 = local read "DNA Channel"() -> (w1709:dbl)
                          n1808 = call "SequenceSelector_LoadPerReactor.vi"("Reactor 6"=w1707, "Reactor 7"=w1707, "Reactor 8"=w1708, "Loop Iteration"=w1712, "Reactor 5"=w1707, "Reactor 4"=w1707, "Current Reactor"=w1710, "Reactor 3"=w1707, "Reactor 2"=w1707, "Reactor 1"=w1708, "Inflow Channel Selector"=w1709) -> ("Array"=w1713:u8[][])
                          n1809 = Index Array(array=w1713, index (col)=w1716) -> (element=w1711:u8[])  [unwired: 1 in]
                          n1810 = Byte Array To String(unsigned byte array=w1711) -> (string=w1717:string)
                          n1811 = Enqueue Element(queue=w1714, element=w1717, error in (no error)=w1715) -> (error out=w1719:errorcluster)  [unwired: 1 in, 2 out]
                          n1812 = call "StorePreviousSwitchValues.vi"("Array"=w1711) -> ()  [unwired: 3 in]
                          n1813 = Wait (ms)(milliseconds to wait=15) -> ()  [unwired: 1 out]
                        }
                      }
                    }
                    frame #14 {
                      w1723 = 5
                      # "Step 8.5:\nLoad DNA"
                      n1814 = local read "Refresh Fraction [%]"() -> (w1720:dbl)
                      n1815 = local read "DNA  High RR"() -> (w1728:dbl)
                      n1816 = Subtract(x=w1723, y=1) -> (x-y=w1721:i32)
                      n1817 = global write "CurrentSwitchValues_GlobalVariable.vi" "Current Reactor"(w1723) -> ()
                      n1818 = Divide(x=100, y=w1720) -> (x/y=w1725:dbl)
                      n1819 = call "ConvertDesiredRefreshRatioPerReactor.vi"("Desired Refresh Ratio"=w1728, "Reactor"=w1721) -> ("Required Number of Pump Iterations"=w1729:dbl)
                      n1820 = Round To Nearest(number=w1725) -> (nearest integer value=w1724:dbl)
                      n1821 = Divide(x=w1729, y=w1724) -> (x/y=w1730:dbl)
                      n1822 = Round To Nearest(number=w1730) -> (nearest integer value=w1727:dbl)
                      n1823 = for {
                        N: w1727 -> [_]
                        tunnel: [w1737] -> _
                        tunnel: w1732 -> [w1734]
                        tunnel: w1731 -> [w1733]
                        i -> [w1735]
                        n1824 = for {
                          N: 6 -> [_]
                          tunnel: [w1750] -> w1737
                          tunnel: w1735 -> [w1743]
                          tunnel: w1734 -> [w1746]
                          tunnel: w1733 -> [w1745]
                          i -> [w1747]
                          w1738 = TRUE
                          w1739 = TRUE
                          n1825 = global read "CurrentSwitchValues_GlobalVariable.vi" "Current Reactor"() -> (w1741:dbl)
                          n1826 = local read "DNA Channel"() -> (w1740:dbl)
                          n1827 = call "SequenceSelector_LoadPerReactor.vi"("Reactor 6"=w1738, "Reactor 7"=w1738, "Reactor 8"=w1739, "Loop Iteration"=w1743, "Reactor 5"=w1738, "Reactor 4"=w1738, "Current Reactor"=w1741, "Reactor 3"=w1738, "Reactor 2"=w1738, "Reactor 1"=w1739, "Inflow Channel Selector"=w1740) -> ("Array"=w1744:u8[][])
                          n1828 = Index Array(array=w1744, index (col)=w1747) -> (element=w1742:u8[])  [unwired: 1 in]
                          n1829 = Byte Array To String(unsigned byte array=w1742) -> (string=w1748:string)
                          n1830 = Enqueue Element(queue=w1745, element=w1748, error in (no error)=w1746) -> (error out=w1750:errorcluster)  [unwired: 1 in, 2 out]
                          n1831 = call "StorePreviousSwitchValues.vi"("Array"=w1742) -> ()  [unwired: 3 in]
                          n1832 = Wait (ms)(milliseconds to wait=15) -> ()  [unwired: 1 out]
                        }
                      }
                    }
                    frame #15 {
                      w1754 = 6
                      # "Step 8.5:\nLoad DNA"
                      n1833 = local read "Refresh Fraction [%]"() -> (w1751:dbl)
                      n1834 = local read "DNA  High RR"() -> (w1759:dbl)
                      n1835 = Subtract(x=w1754, y=1) -> (x-y=w1752:i32)
                      n1836 = global write "CurrentSwitchValues_GlobalVariable.vi" "Current Reactor"(w1754) -> ()
                      n1837 = Divide(x=100, y=w1751) -> (x/y=w1756:dbl)
                      n1838 = call "ConvertDesiredRefreshRatioPerReactor.vi"("Desired Refresh Ratio"=w1759, "Reactor"=w1752) -> ("Required Number of Pump Iterations"=w1760:dbl)
                      n1839 = Round To Nearest(number=w1756) -> (nearest integer value=w1755:dbl)
                      n1840 = Divide(x=w1760, y=w1755) -> (x/y=w1761:dbl)
                      n1841 = Round To Nearest(number=w1761) -> (nearest integer value=w1758:dbl)
                      n1842 = for {
                        N: w1758 -> [_]
                        tunnel: [w1768] -> _
                        tunnel: w1763 -> [w1765]
                        tunnel: w1762 -> [w1764]
                        i -> [w1766]
                        n1843 = for {
                          N: 6 -> [_]
                          tunnel: [w1781] -> w1768
                          tunnel: w1766 -> [w1774]
                          tunnel: w1765 -> [w1777]
                          tunnel: w1764 -> [w1776]
                          i -> [w1778]
                          w1769 = TRUE
                          w1770 = TRUE
                          n1844 = global read "CurrentSwitchValues_GlobalVariable.vi" "Current Reactor"() -> (w1772:dbl)
                          n1845 = local read "DNA Channel"() -> (w1771:dbl)
                          n1846 = call "SequenceSelector_LoadPerReactor.vi"("Reactor 6"=w1769, "Reactor 7"=w1769, "Reactor 8"=w1770, "Loop Iteration"=w1774, "Reactor 5"=w1769, "Reactor 4"=w1769, "Current Reactor"=w1772, "Reactor 3"=w1769, "Reactor 2"=w1769, "Reactor 1"=w1770, "Inflow Channel Selector"=w1771) -> ("Array"=w1775:u8[][])
                          n1847 = Index Array(array=w1775, index (col)=w1778) -> (element=w1773:u8[])  [unwired: 1 in]
                          n1848 = Byte Array To String(unsigned byte array=w1773) -> (string=w1779:string)
                          n1849 = Enqueue Element(queue=w1776, element=w1779, error in (no error)=w1777) -> (error out=w1781:errorcluster)  [unwired: 1 in, 2 out]
                          n1850 = call "StorePreviousSwitchValues.vi"("Array"=w1773) -> ()  [unwired: 3 in]
                          n1851 = Wait (ms)(milliseconds to wait=15) -> ()  [unwired: 1 out]
                        }
                      }
                    }
                    frame #16 {
                      w1785 = 7
                      # "Step 8.5:\nLoad DNA"
                      n1852 = local read "Refresh Fraction [%]"() -> (w1782:dbl)
                      n1853 = local read "DNA  High RR"() -> (w1790:dbl)
                      n1854 = Subtract(x=w1785, y=1) -> (x-y=w1783:i32)
                      n1855 = global write "CurrentSwitchValues_GlobalVariable.vi" "Current Reactor"(w1785) -> ()
                      n1856 = Divide(x=100, y=w1782) -> (x/y=w1787:dbl)
                      n1857 = call "ConvertDesiredRefreshRatioPerReactor.vi"("Desired Refresh Ratio"=w1790, "Reactor"=w1783) -> ("Required Number of Pump Iterations"=w1791:dbl)
                      n1858 = Round To Nearest(number=w1787) -> (nearest integer value=w1786:dbl)
                      n1859 = Divide(x=w1791, y=w1786) -> (x/y=w1792:dbl)
                      n1860 = Round To Nearest(number=w1792) -> (nearest integer value=w1789:dbl)
                      n1861 = for {
                        N: w1789 -> [_]
                        tunnel: [w1799] -> _
                        tunnel: w1794 -> [w1796]
                        tunnel: w1793 -> [w1795]
                        i -> [w1797]
                        n1862 = for {
                          N: 6 -> [_]
                          tunnel: [w1812] -> w1799
                          tunnel: w1797 -> [w1805]
                          tunnel: w1796 -> [w1808]
                          tunnel: w1795 -> [w1807]
                          i -> [w1809]
                          w1800 = TRUE
                          w1801 = TRUE
                          n1863 = global read "CurrentSwitchValues_GlobalVariable.vi" "Current Reactor"() -> (w1803:dbl)
                          n1864 = local read "DNA Channel"() -> (w1802:dbl)
                          n1865 = call "SequenceSelector_LoadPerReactor.vi"("Reactor 6"=w1800, "Reactor 7"=w1800, "Reactor 8"=w1801, "Loop Iteration"=w1805, "Reactor 5"=w1800, "Reactor 4"=w1800, "Current Reactor"=w1803, "Reactor 3"=w1800, "Reactor 2"=w1800, "Reactor 1"=w1801, "Inflow Channel Selector"=w1802) -> ("Array"=w1806:u8[][])
                          n1866 = Index Array(array=w1806, index (col)=w1809) -> (element=w1804:u8[])  [unwired: 1 in]
                          n1867 = Byte Array To String(unsigned byte array=w1804) -> (string=w1810:string)
                          n1868 = Enqueue Element(queue=w1807, element=w1810, error in (no error)=w1808) -> (error out=w1812:errorcluster)  [unwired: 1 in, 2 out]
                          n1869 = call "StorePreviousSwitchValues.vi"("Array"=w1804) -> ()  [unwired: 3 in]
                          n1870 = Wait (ms)(milliseconds to wait=15) -> ()  [unwired: 1 out]
                        }
                      }
                    }
                    frame #17 {
                      # "Step 8.6: \nFlush Elution Buffer"
                      n1871 = for {
                        N: 150 -> [_]
                        tunnel: w1814 -> [w1818]
                        tunnel: w1813 -> [w1817]
                        tunnel: [w1816] -> _
                        n1872 = for {
                          N: 6 -> [_]
                          tunnel: w1818 -> [w1823]
                          tunnel: w1817 -> [w1822]
                          tunnel: [w1821] -> w1816
                          i -> [w1827]
                          # "T-wait is 100 ms,\nfreq = +-1.7Hz if fast and T-wait is 556ms, freq = 0.3Hz if slow flush."
                          n1873 = local read "Elution Buffer"() -> (w1820:dbl)
                          n1874 = call "SequenceSelector_Flush.vi"("Inflow Channel Selector"=w1820) -> ("Array"=w1826:u8[][])
                          n1875 = Wait (ms)(milliseconds to wait=50) -> ()  [unwired: 1 out]
                          n1876 = Index Array(array=w1826, index (col)=w1827) -> (element=w1828:u8[])  [unwired: 1 in]
                          n1877 = call "StorePreviousSwitchValues.vi"("Array"=w1828) -> ()  [unwired: 3 in]
                          n1878 = Byte Array To String(unsigned byte array=w1828) -> (string=w1824:string)
                          n1879 = Enqueue Element(queue=w1822, element=w1824, error in (no error)=w1823) -> (error out=w1821:errorcluster)  [unwired: 1 in, 2 out]
                        }
                      }
                    }
                    frame #18 {
                      w1832 = 1
                      # "Step 8.7:\nLoad H20 into control channels"
                      n1880 = local read "Refresh Fraction [%]"() -> (w1829:dbl)
                      n1881 = local read "Elution Buffer RR"() -> (w1837:dbl)
                      n1882 = Subtract(x=w1832, y=1) -> (x-y=w1830:i32)
                      n1883 = global write "CurrentSwitchValues_GlobalVariable.vi" "Current Reactor"(w1832) -> ()
                      n1884 = Divide(x=100, y=w1829) -> (x/y=w1834:dbl)
                      n1885 = call "ConvertDesiredRefreshRatioPerReactor.vi"("Desired Refresh Ratio"=w1837, "Reactor"=w1830) -> ("Required Number of Pump Iterations"=w1838:dbl)
                      n1886 = Round To Nearest(number=w1834) -> (nearest integer value=w1833:dbl)
                      n1887 = Divide(x=w1838, y=w1833) -> (x/y=w1839:dbl)
                      n1888 = Round To Nearest(number=w1839) -> (nearest integer value=w1836:dbl)
                      n1889 = for {
                        N: w1836 -> [_]
                        tunnel: [w1846] -> _
                        tunnel: w1841 -> [w1843]
                        tunnel: w1840 -> [w1842]
                        i -> [w1844]
                        n1890 = for {
                          N: 6 -> [_]
                          tunnel: [w1859] -> w1846
                          tunnel: w1844 -> [w1852]
                          tunnel: w1843 -> [w1855]
                          tunnel: w1842 -> [w1854]
                          i -> [w1856]
                          w1847 = TRUE
                          w1848 = TRUE
                          n1891 = global read "CurrentSwitchValues_GlobalVariable.vi" "Current Reactor"() -> (w1850:dbl)
                          n1892 = local read "Elution Buffer"() -> (w1849:dbl)
                          n1893 = call "SequenceSelector_LoadPerReactor.vi"("Reactor 6"=w1847, "Reactor 7"=w1847, "Reactor 8"=w1848, "Loop Iteration"=w1852, "Reactor 5"=w1847, "Reactor 4"=w1847, "Current Reactor"=w1850, "Reactor 3"=w1847, "Reactor 2"=w1847, "Reactor 1"=w1848, "Inflow Channel Selector"=w1849) -> ("Array"=w1853:u8[][])
                          n1894 = Index Array(array=w1853, index (col)=w1856) -> (element=w1851:u8[])  [unwired: 1 in]
                          n1895 = Byte Array To String(unsigned byte array=w1851) -> (string=w1857:string)
                          n1896 = Enqueue Element(queue=w1854, element=w1857, error in (no error)=w1855) -> (error out=w1859:errorcluster)  [unwired: 1 in, 2 out]
                          n1897 = call "StorePreviousSwitchValues.vi"("Array"=w1851) -> ()  [unwired: 3 in]
                          n1898 = Wait (ms)(milliseconds to wait=15) -> ()  [unwired: 1 out]
                        }
                      }
                    }
                    frame #19 {
                      w1863 = 8
                      # "Step 8.7:\nLoad H20 into control channels"
                      n1899 = local read "Refresh Fraction [%]"() -> (w1860:dbl)
                      n1900 = local read "Elution Buffer RR"() -> (w1868:dbl)
                      n1901 = Subtract(x=w1863, y=1) -> (x-y=w1861:i32)
                      n1902 = global write "CurrentSwitchValues_GlobalVariable.vi" "Current Reactor"(w1863) -> ()
                      n1903 = Divide(x=100, y=w1860) -> (x/y=w1865:dbl)
                      n1904 = call "ConvertDesiredRefreshRatioPerReactor.vi"("Desired Refresh Ratio"=w1868, "Reactor"=w1861) -> ("Required Number of Pump Iterations"=w1869:dbl)
                      n1905 = Round To Nearest(number=w1865) -> (nearest integer value=w1864:dbl)
                      n1906 = Divide(x=w1869, y=w1864) -> (x/y=w1870:dbl)
                      n1907 = Round To Nearest(number=w1870) -> (nearest integer value=w1867:dbl)
                      n1908 = for {
                        N: w1867 -> [_]
                        tunnel: [w1877] -> _
                        tunnel: w1872 -> [w1874]
                        tunnel: w1871 -> [w1873]
                        i -> [w1875]
                        n1909 = for {
                          N: 6 -> [_]
                          tunnel: [w1890] -> w1877
                          tunnel: w1875 -> [w1883]
                          tunnel: w1874 -> [w1886]
                          tunnel: w1873 -> [w1885]
                          i -> [w1887]
                          w1878 = TRUE
                          w1879 = TRUE
                          n1910 = global read "CurrentSwitchValues_GlobalVariable.vi" "Current Reactor"() -> (w1881:dbl)
                          n1911 = local read "Elution Buffer"() -> (w1880:dbl)
                          n1912 = call "SequenceSelector_LoadPerReactor.vi"("Reactor 6"=w1878, "Reactor 7"=w1878, "Reactor 8"=w1879, "Loop Iteration"=w1883, "Reactor 5"=w1878, "Reactor 4"=w1878, "Current Reactor"=w1881, "Reactor 3"=w1878, "Reactor 2"=w1878, "Reactor 1"=w1879, "Inflow Channel Selector"=w1880) -> ("Array"=w1884:u8[][])
                          n1913 = Index Array(array=w1884, index (col)=w1887) -> (element=w1882:u8[])  [unwired: 1 in]
                          n1914 = Byte Array To String(unsigned byte array=w1882) -> (string=w1888:string)
                          n1915 = Enqueue Element(queue=w1885, element=w1888, error in (no error)=w1886) -> (error out=w1890:errorcluster)  [unwired: 1 in, 2 out]
                          n1916 = call "StorePreviousSwitchValues.vi"("Array"=w1882) -> ()  [unwired: 3 in]
                          n1917 = Wait (ms)(milliseconds to wait=15) -> ()  [unwired: 1 out]
                        }
                      }
                    }
                    frame #20 {
                      # "Step 8.8:\nMixing"
                      # "For the time between dilutions to take 12 minutes, the mixing sequence will be executed 12 times. (Each mixing cycle takes exactly 1 minute)"
                      n1918 = for {
                        N: 13 -> [_]
                        tunnel: w1893 -> [w1897]
                        tunnel: w1892 -> [w1896]
                        tunnel: [w1895] -> _
                        i -> [w1902]
                        # "Number of mix cycles = 12"
                        n1919 = for {
                          N: 500 -> [_]
                          tunnel: w1897 -> [w1914]
                          tunnel: w1896 -> [w1913]
                          tunnel: [w1912] -> w1895
                          n1920 = for {
                            N: 6 -> [_]
                            tunnel: w1914 -> [w1918]
                            tunnel: w1913 -> [w1917]
                            tunnel: [w1916] -> w1912
                            i -> [w1921]
                            # "T-wait is 20 ms\nfreq = +-8.3Hz"
                            n1921 = Wait (ms)(milliseconds to wait=20) -> ()  [unwired: 1 out]
                            n1922 = Index Array(array=u8[][] [[0, 0, 0, 0, 0, 0, 0, 0, 2, 4, 3, 3, 3, 3], [0, 0, 0, 0, 0, 0, 0, 0, 0, 0, 0, 0, 0, 0], [0, 0, 0, 0, 0, 0, 0, 0, 0, 0, 0, 0, 0, 0], [0, 0, 0, 0, 0, 0, 0, 0, 0, 0, 0, 0, 0, 0], [0, 0, 0, 0, 0, 0, 0, 0, 0, 0, 0, 0, 0, 0], [11, 11, 11, 11, 11, 11, 11, 0, 0, 0, 0, 0, 0, 0], [0, 0, 0, 0, 0, 0, 0, 0, 0, 0, 0, 0, 0, 0], [16, 16, 16, 16, 16, 16, 16, 0, 0, 0, 0, 0, 0, 0], [0, 0, 0, 0, 0, 0, 0, 0, 0, 0, 0, 0, 0, 0], [0, 0, 0, 0, 0, 0, 0, 0, 0, 0, 0, 0, 0, 0], [0, 0, 0, 0, 0, 0, 0, 0, 0, 0, 0, 0, 0, 0], [2, 2, 2, 2, 2, 2, 2, 0, 0, 0, 0, 0, 0, 0], [4, 4, 4, 4, 4, 4, 4, 0, 0, 0, 0, 0, 0, 0], [255, 255, 255, 255, 255, 255, 0, 0, 0, 0, 0, 0, 0, 0], [3, 2, 6, 4, 5, 1, 0, 0, 0, 0, 0, 0, 0, 0], [27, 27, 27, 27, 27, 27, 0, 0, 0, 0, 0, 0, 0, 0], [255, 255, 255, 255, 255, 255, 0, 0, 0, 0, 0, 0, 0, 0]], index (col)=w1921) -> (element=w1922:u8[])  [unwired: 1 in]
                            n1923 = Byte Array To String(unsigned byte array=w1922) -> (string=w1919:string)
                            n1924 = call "StorePreviousSwitchValues.vi"("Array"=w1922) -> ()  [unwired: 3 in]
                            n1925 = Enqueue Element(queue=w1917, element=w1919, error in (no error)=w1918) -> (error out=w1916:errorcluster)  [unwired: 1 in, 2 out]
                          }
                        }
                        n1926 = Add(x=1, y=w1902) -> (x+y=w1898:i32)
                        n1927 = Less?(x=w1898, y=10) -> (x < y?=w1899:bool)
                        n1928 = case shown="True" w1899 {
                          frame False {
                          }
                          frame True {
                            n1929 = local read "Time between Mixing Cycles Initialisation"() -> (w1910:dbl)
                            n1930 = Multiply(x=60000, y=w1910) -> (x*y=w1904:dbl)
                            n1931 = Multiply(x=20, y=500) -> (x*y=w1907:i32)
                            n1932 = Multiply(x=w1907, y=6) -> (x*y=w1906:i32)
                            n1933 = Add(x=w1904, y=w1906) -> (x+y=w1903:dbl)
                            n1934 = Wait (ms)(milliseconds to wait=w1903) -> ()  [unwired: 1 out]
                          }
                        }
                      }
                    }
                    frame #21 {
                      w1927 = u8[] [0, 0, 0, 0, 0, 11, 0, 16, 0, 0, 0, 2, 4, 255, 7, 31, 255]
                      # "Step 12.12:\nClose all channels to halt flow"
                      n1935 = Byte Array To String(unsigned byte array=w1927) -> (string=w1926:string)
                      n1936 = call "StorePreviousSwitchValues.vi"("Array"=w1927) -> ()  [unwired: 3 in]
                      n1937 = Enqueue Element(queue=w1925, element=w1926, error in (no error)=w1924) -> ()  [unwired: 1 in, 3 out]
                    }
                    frame #22 {
                      # "STEP 12.13: \n\nSave the current switch states to the global variables."
                      n1938 = global read "CurrentSwitchValues_GlobalVariable.vi" "1"() -> (w1957:bool)
                      n1939 = global read "CurrentSwitchValues_GlobalVariable.vi" "3"() -> (w1950:bool)
                      n1940 = global read "CurrentSwitchValues_GlobalVariable.vi" "5"() -> (w1952:bool)
                      n1941 = global read "CurrentSwitchValues_GlobalVariable.vi" "7"() -> (w1954:bool)
                      n1942 = global read "CurrentSwitchValues_GlobalVariable.vi" "9"() -> (w1942:bool)
                      n1943 = global read "CurrentSwitchValues_GlobalVariable.vi" "11"() -> (w1944:bool)
                      n1944 = global read "CurrentSwitchValues_GlobalVariable.vi" "13"() -> (w1946:bool)
                      n1945 = global read "CurrentSwitchValues_GlobalVariable.vi" "15"() -> (w1948:bool)
                      n1946 = global read "CurrentSwitchValues_GlobalVariable.vi" "17"() -> (w1934:bool)
                      n1947 = global read "CurrentSwitchValues_GlobalVariable.vi" "19"() -> (w1936:bool)
                      n1948 = global read "CurrentSwitchValues_GlobalVariable.vi" "21"() -> (w1938:bool)
                      n1949 = global read "CurrentSwitchValues_GlobalVariable.vi" "23"() -> (w1940:bool)
                      n1950 = global read "CurrentSwitchValues_GlobalVariable.vi" "25"() -> (w1933:bool)
                      n1951 = global read "CurrentSwitchValues_GlobalVariable.vi" "27"() -> (w1931:bool)
                      n1952 = global read "CurrentSwitchValues_GlobalVariable.vi" "29"() -> (w1929:bool)
                      n1953 = global read "CurrentSwitchValues_GlobalVariable.vi" "10"() -> (w1943:bool)
                      n1954 = global read "CurrentSwitchValues_GlobalVariable.vi" "12"() -> (w1945:bool)
                      n1955 = global read "CurrentSwitchValues_GlobalVariable.vi" "14"() -> (w1947:bool)
                      n1956 = global read "CurrentSwitchValues_GlobalVariable.vi" "16"() -> (w1949:bool)
                      n1957 = global read "CurrentSwitchValues_GlobalVariable.vi" "2"() -> (w1956:bool)
                      n1958 = global read "CurrentSwitchValues_GlobalVariable.vi" "6"() -> (w1953:bool)
                      n1959 = global read "CurrentSwitchValues_GlobalVariable.vi" "4"() -> (w1951:bool)
                      n1960 = global read "CurrentSwitchValues_GlobalVariable.vi" "8"() -> (w1955:bool)
                      n1961 = global read "CurrentSwitchValues_GlobalVariable.vi" "18"() -> (w1935:bool)
                      n1962 = global read "CurrentSwitchValues_GlobalVariable.vi" "20"() -> (w1937:bool)
                      n1963 = global read "CurrentSwitchValues_GlobalVariable.vi" "22"() -> (w1939:bool)
                      n1964 = global read "CurrentSwitchValues_GlobalVariable.vi" "24"() -> (w1941:bool)
                      n1965 = global read "CurrentSwitchValues_GlobalVariable.vi" "26"() -> (w1932:bool)
                      n1966 = global read "CurrentSwitchValues_GlobalVariable.vi" "28"() -> (w1930:bool)
                      n1967 = global read "CurrentSwitchValues_GlobalVariable.vi" "30"() -> (w1928:bool)
                      n1968 = property on="3" class="Bool (strict)"("Value"=w1950) -> ()  [unwired: 2 in, 2 out]
                      n1969 = property on="5" class="Bool (strict)"("Value"=w1952) -> ()  [unwired: 2 in, 2 out]
                      n1970 = property on="7" class="Bool (strict)"("Value"=w1954) -> ()  [unwired: 2 in, 2 out]
                      n1971 = property on="9" class="Bool (strict)"("Value"=w1942) -> ()  [unwired: 2 in, 2 out]
                      n1972 = property on="11" class="Bool (strict)"("Value"=w1944) -> ()  [unwired: 2 in, 2 out]
                      n1973 = property on="13" class="Bool (strict)"("Value"=w1946) -> ()  [unwired: 2 in, 2 out]
                      n1974 = property on="15" class="Bool (strict)"("Value"=w1948) -> ()  [unwired: 2 in, 2 out]
                      n1975 = property on="17" class="Bool (strict)"("Value"=w1934) -> ()  [unwired: 2 in, 2 out]
                      n1976 = property on="19" class="Bool (strict)"("Value"=w1936) -> ()  [unwired: 2 in, 2 out]
                      n1977 = property on="21" class="Bool (strict)"("Value"=w1938) -> ()  [unwired: 2 in, 2 out]
                      n1978 = property on="23" class="Bool (strict)"("Value"=w1940) -> ()  [unwired: 2 in, 2 out]
                      n1979 = property on="25" class="Bool (strict)"("Value"=w1933) -> ()  [unwired: 2 in, 2 out]
                      n1980 = property on="27" class="Bool (strict)"("Value"=w1931) -> ()  [unwired: 2 in, 2 out]
                      n1981 = property on="29" class="Bool (strict)"("Value"=w1929) -> ()  [unwired: 2 in, 2 out]
                      n1982 = property on="1" class="Bool (strict)"("Value"=w1957) -> ()  [unwired: 2 in, 2 out]
                      n1983 = property on="26" class="Bool (strict)"("Value"=w1932) -> ()  [unwired: 2 in, 2 out]
                      n1984 = property on="28" class="Bool (strict)"("Value"=w1930) -> ()  [unwired: 2 in, 2 out]
                      n1985 = property on="30" class="Bool (strict)"("Value"=w1928) -> ()  [unwired: 2 in, 2 out]
                      n1986 = property on="2" class="Bool (strict)"("Value"=w1956) -> ()  [unwired: 2 in, 2 out]
                      n1987 = property on="4" class="Bool (strict)"("Value"=w1951) -> ()  [unwired: 2 in, 2 out]
                      n1988 = property on="6" class="Bool (strict)"("Value"=w1953) -> ()  [unwired: 2 in, 2 out]
                      n1989 = property on="8" class="Bool (strict)"("Value"=w1955) -> ()  [unwired: 2 in, 2 out]
                      n1990 = property on="10" class="Bool (strict)"("Value"=w1943) -> ()  [unwired: 2 in, 2 out]
                      n1991 = property on="12" class="Bool (strict)"("Value"=w1945) -> ()  [unwired: 2 in, 2 out]
                      n1992 = property on="14" class="Bool (strict)"("Value"=w1947) -> ()  [unwired: 2 in, 2 out]
                      n1993 = property on="16" class="Bool (strict)"("Value"=w1949) -> ()  [unwired: 2 in, 2 out]
                      n1994 = property on="18" class="Bool (strict)"("Value"=w1935) -> ()  [unwired: 2 in, 2 out]
                      n1995 = property on="20" class="Bool (strict)"("Value"=w1937) -> ()  [unwired: 2 in, 2 out]
                      n1996 = property on="22" class="Bool (strict)"("Value"=w1939) -> ()  [unwired: 2 in, 2 out]
                      n1997 = property on="24" class="Bool (strict)"("Value"=w1941) -> ()  [unwired: 2 in, 2 out]
                    }
                  }
                }
              }
              frame #8 {
                # "Step 1:\nThe primary step in this simple expression\nprotocol is to flush the device with elution \nbuffer to ensure the removal of any residual\nsolutes from the calibration protocol."
                n1998 = stacked-sequence {
                  tunnel: w1959 -> [w1962 w1977 _]
                  tunnel: w1958 -> [w1961 w1978 _]
                  tunnel: [w1960 _ _] -> _
                  frame #0 {
                    n1999 = for {
                      N: 500 -> [_]
                      tunnel: w1962 -> [w1966]
                      tunnel: w1961 -> [w1965]
                      tunnel: [w1964] -> w1960
                      n2000 = for {
                        N: 6 -> [_]
                        tunnel: w1966 -> [w1971]
                        tunnel: w1965 -> [w1970]
                        tunnel: [w1969] -> w1964
                        i -> [w1975]
                        # "T-wait is 100 ms,\nfreq = +-1.7Hz if fast and T-wait is 556ms, freq = 0.3Hz if slow flush."
                        n2001 = local read "Elution Buffer"() -> (w1968:dbl)
                        n2002 = call "SequenceSelector_Flush.vi"("Inflow Channel Selector"=w1968) -> ("Array"=w1974:u8[][])
                        n2003 = Wait (ms)(milliseconds to wait=25) -> ()  [unwired: 1 out]
                        n2004 = Index Array(array=w1974, index (col)=w1975) -> (element=w1976:u8[])  [unwired: 1 in]
                        n2005 = call "StorePreviousSwitchValues.vi"("Array"=w1976) -> ()  [unwired: 3 in]
                        n2006 = Byte Array To String(unsigned byte array=w1976) -> (string=w1972:string)
                        n2007 = Enqueue Element(queue=w1970, element=w1972, error in (no error)=w1971) -> (error out=w1969:errorcluster)  [unwired: 1 in, 2 out]
                      }
                    }
                  }
                  frame #1 {
                    w1980 = u8[] [0, 0, 0, 0, 0, 11, 0, 16, 0, 0, 0, 2, 4, 255, 7, 31, 255]
                    n2008 = call "StorePreviousSwitchValues.vi"("Array"=w1980) -> ()  [unwired: 3 in]
                    n2009 = Byte Array To String(unsigned byte array=w1980) -> (string=w1979:string)
                    n2010 = Enqueue Element(queue=w1978, element=w1979, error in (no error)=w1977) -> ()  [unwired: 1 in, 3 out]
                  }
                  frame #2 {
                    n2011 = global read "CurrentSwitchValues_GlobalVariable.vi" "1"() -> (w2010:bool)
                    n2012 = global read "CurrentSwitchValues_GlobalVariable.vi" "3"() -> (w2003:bool)
                    n2013 = global read "CurrentSwitchValues_GlobalVariable.vi" "5"() -> (w2005:bool)
                    n2014 = global read "CurrentSwitchValues_GlobalVariable.vi" "7"() -> (w2007:bool)
                    n2015 = global read "CurrentSwitchValues_GlobalVariable.vi" "9"() -> (w1995:bool)
                    n2016 = global read "CurrentSwitchValues_GlobalVariable.vi" "11"() -> (w1997:bool)
                    n2017 = global read "CurrentSwitchValues_GlobalVariable.vi" "13"() -> (w1999:bool)
                    n2018 = global read "CurrentSwitchValues_GlobalVariable.vi" "15"() -> (w2001:bool)
                    n2019 = global read "CurrentSwitchValues_GlobalVariable.vi" "17"() -> (w1987:bool)
                    n2020 = global read "CurrentSwitchValues_GlobalVariable.vi" "19"() -> (w1989:bool)
                    n2021 = global read "CurrentSwitchValues_GlobalVariable.vi" "21"() -> (w1991:bool)
                    n2022 = global read "CurrentSwitchValues_GlobalVariable.vi" "23"() -> (w1993:bool)
                    n2023 = global read "CurrentSwitchValues_GlobalVariable.vi" "25"() -> (w1986:bool)
                    n2024 = global read "CurrentSwitchValues_GlobalVariable.vi" "27"() -> (w1984:bool)
                    n2025 = global read "CurrentSwitchValues_GlobalVariable.vi" "29"() -> (w1982:bool)
                    n2026 = global read "CurrentSwitchValues_GlobalVariable.vi" "10"() -> (w1996:bool)
                    n2027 = global read "CurrentSwitchValues_GlobalVariable.vi" "12"() -> (w1998:bool)
                    n2028 = global read "CurrentSwitchValues_GlobalVariable.vi" "14"() -> (w2000:bool)
                    n2029 = global read "CurrentSwitchValues_GlobalVariable.vi" "16"() -> (w2002:bool)
                    n2030 = global read "CurrentSwitchValues_GlobalVariable.vi" "2"() -> (w2009:bool)
                    n2031 = global read "CurrentSwitchValues_GlobalVariable.vi" "6"() -> (w2006:bool)
                    n2032 = global read "CurrentSwitchValues_GlobalVariable.vi" "4"() -> (w2004:bool)
                    n2033 = global read "CurrentSwitchValues_GlobalVariable.vi" "8"() -> (w2008:bool)
                    n2034 = global read "CurrentSwitchValues_GlobalVariable.vi" "18"() -> (w1988:bool)
                    n2035 = global read "CurrentSwitchValues_GlobalVariable.vi" "20"() -> (w1990:bool)
                    n2036 = global read "CurrentSwitchValues_GlobalVariable.vi" "22"() -> (w1992:bool)
                    n2037 = global read "CurrentSwitchValues_GlobalVariable.vi" "24"() -> (w1994:bool)
                    n2038 = global read "CurrentSwitchValues_GlobalVariable.vi" "26"() -> (w1985:bool)
                    n2039 = global read "CurrentSwitchValues_GlobalVariable.vi" "28"() -> (w1983:bool)
                    n2040 = global read "CurrentSwitchValues_GlobalVariable.vi" "30"() -> (w1981:bool)
                    n2041 = property on="1" class="Bool (strict)"("Value"=w2010) -> ()  [unwired: 2 in, 2 out]
                    n2042 = property on="3" class="Bool (strict)"("Value"=w2003) -> ()  [unwired: 2 in, 2 out]
                    n2043 = property on="5" class="Bool (strict)"("Value"=w2005) -> ()  [unwired: 2 in, 2 out]
                    n2044 = property on="7" class="Bool (strict)"("Value"=w2007) -> ()  [unwired: 2 in, 2 out]
                    n2045 = property on="9" class="Bool (strict)"("Value"=w1995) -> ()  [unwired: 2 in, 2 out]
                    n2046 = property on="11" class="Bool (strict)"("Value"=w1997) -> ()  [unwired: 2 in, 2 out]
                    n2047 = property on="13" class="Bool (strict)"("Value"=w1999) -> ()  [unwired: 2 in, 2 out]
                    n2048 = property on="15" class="Bool (strict)"("Value"=w2001) -> ()  [unwired: 2 in, 2 out]
                    n2049 = property on="17" class="Bool (strict)"("Value"=w1987) -> ()  [unwired: 2 in, 2 out]
                    n2050 = property on="19" class="Bool (strict)"("Value"=w1989) -> ()  [unwired: 2 in, 2 out]
                    n2051 = property on="21" class="Bool (strict)"("Value"=w1991) -> ()  [unwired: 2 in, 2 out]
                    n2052 = property on="23" class="Bool (strict)"("Value"=w1993) -> ()  [unwired: 2 in, 2 out]
                    n2053 = property on="25" class="Bool (strict)"("Value"=w1986) -> ()  [unwired: 2 in, 2 out]
                    n2054 = property on="27" class="Bool (strict)"("Value"=w1984) -> ()  [unwired: 2 in, 2 out]
                    n2055 = property on="29" class="Bool (strict)"("Value"=w1982) -> ()  [unwired: 2 in, 2 out]
                    n2056 = property on="26" class="Bool (strict)"("Value"=w1985) -> ()  [unwired: 2 in, 2 out]
                    n2057 = property on="28" class="Bool (strict)"("Value"=w1983) -> ()  [unwired: 2 in, 2 out]
                    n2058 = property on="30" class="Bool (strict)"("Value"=w1981) -> ()  [unwired: 2 in, 2 out]
                    n2059 = property on="2" class="Bool (strict)"("Value"=w2009) -> ()  [unwired: 2 in, 2 out]
                    n2060 = property on="4" class="Bool (strict)"("Value"=w2004) -> ()  [unwired: 2 in, 2 out]
                    n2061 = property on="6" class="Bool (strict)"("Value"=w2006) -> ()  [unwired: 2 in, 2 out]
                    n2062 = property on="8" class="Bool (strict)"("Value"=w2008) -> ()  [unwired: 2 in, 2 out]
                    n2063 = property on="10" class="Bool (strict)"("Value"=w1996) -> ()  [unwired: 2 in, 2 out]
                    n2064 = property on="12" class="Bool (strict)"("Value"=w1998) -> ()  [unwired: 2 in, 2 out]
                    n2065 = property on="14" class="Bool (strict)"("Value"=w2000) -> ()  [unwired: 2 in, 2 out]
                    n2066 = property on="16" class="Bool (strict)"("Value"=w2002) -> ()  [unwired: 2 in, 2 out]
                    n2067 = property on="18" class="Bool (strict)"("Value"=w1988) -> ()  [unwired: 2 in, 2 out]
                    n2068 = property on="20" class="Bool (strict)"("Value"=w1990) -> ()  [unwired: 2 in, 2 out]
                    n2069 = property on="22" class="Bool (strict)"("Value"=w1992) -> ()  [unwired: 2 in, 2 out]
                    n2070 = property on="24" class="Bool (strict)"("Value"=w1994) -> ()  [unwired: 2 in, 2 out]
                  }
                }
              }
              frame #9 {
                # "Step 2:\nThe second part of the initialisation is to fill all of\nthe reaction chambers with the elution buffer."
                n2071 = stacked-sequence {
                  tunnel: w2012 -> [w2016 w2033 _]
                  tunnel: w2011 -> [w2015 w2034 _]
                  tunnel: [w2013 _ _] -> _
                  tunnel: [_ w2032 _] -> _
                  frame #0 {
                    # "The number of cycle repeats is set to 500 to completly fill the chambers"
                    n2072 = for {
                      N: 600 -> [_]
                      tunnel: w2016 -> [w2021]
                      tunnel: w2015 -> [w2020]
                      tunnel: [w2019] -> w2013
                      i -> [w2017]
                      n2073 = for {
                        N: 6 -> [_]
                        tunnel: w2021 -> [w2031]
                        tunnel: w2020 -> [w2030]
                        tunnel: [w2029] -> w2019
                        tunnel: w2017 -> [w2022]
                        i -> [w2025]
                        n2074 = local read "Elution Buffer"() -> (w2023:dbl)
                        n2075 = call "SequenceSelector_LoadAllChambers.vi"("Inflow Channel Selector"=w2023, "Loop Iteration"=w2022) -> ("Array"=w2024:u8[][])  [unwired: 7 in]
                        n2076 = Index Array(array=w2024, index (col)=w2025) -> (element=w2028:u8[])  [unwired: 1 in]
                        n2077 = Byte Array To String(unsigned byte array=w2028) -> (string=w2026:string)
                        n2078 = Enqueue Element(queue=w2031, element=w2026, error in (no error)=w2030) -> (error out=w2029:errorcluster)  [unwired: 1 in, 2 out]
                        n2079 = call "StorePreviousSwitchValues.vi"("Array"=w2028) -> ()  [unwired: 3 in]
                        n2080 = Wait (ms)(milliseconds to wait=25) -> ()  [unwired: 1 out]
                      }
                    }
                  }
                  frame #1 {
                    w2036 = u8[] [0, 0, 0, 0, 0, 11, 0, 16, 0, 0, 0, 2, 4, 255, 7, 31, 255]
                    n2081 = Byte Array To String(unsigned byte array=w2036) -> (string=w2035:string)
                    n2082 = call "StorePreviousSwitchValues.vi"("Array"=w2036) -> ()  [unwired: 3 in]
                    n2083 = Enqueue Element(queue=w2033, element=w2035, error in (no error)=w2034) -> (error out=w2032:errorcluster)  [unwired: 1 in, 2 out]
                  }
                  frame #2 {
                    n2084 = global read "CurrentSwitchValues_GlobalVariable.vi" "1"() -> (w2066:bool)
                    n2085 = global read "CurrentSwitchValues_GlobalVariable.vi" "3"() -> (w2059:bool)
                    n2086 = global read "CurrentSwitchValues_GlobalVariable.vi" "5"() -> (w2061:bool)
                    n2087 = global read "CurrentSwitchValues_GlobalVariable.vi" "7"() -> (w2063:bool)
                    n2088 = global read "CurrentSwitchValues_GlobalVariable.vi" "9"() -> (w2051:bool)
                    n2089 = global read "CurrentSwitchValues_GlobalVariable.vi" "11"() -> (w2053:bool)
                    n2090 = global read "CurrentSwitchValues_GlobalVariable.vi" "13"() -> (w2055:bool)
                    n2091 = global read "CurrentSwitchValues_GlobalVariable.vi" "15"() -> (w2057:bool)
                    n2092 = global read "CurrentSwitchValues_GlobalVariable.vi" "17"() -> (w2043:bool)
                    n2093 = global read "CurrentSwitchValues_GlobalVariable.vi" "19"() -> (w2045:bool)
                    n2094 = global read "CurrentSwitchValues_GlobalVariable.vi" "21"() -> (w2047:bool)
                    n2095 = global read "CurrentSwitchValues_GlobalVariable.vi" "23"() -> (w2049:bool)
                    n2096 = global read "CurrentSwitchValues_GlobalVariable.vi" "25"() -> (w2042:bool)
                    n2097 = global read "CurrentSwitchValues_GlobalVariable.vi" "27"() -> (w2040:bool)
                    n2098 = global read "CurrentSwitchValues_GlobalVariable.vi" "29"() -> (w2038:bool)
                    n2099 = global read "CurrentSwitchValues_GlobalVariable.vi" "10"() -> (w2052:bool)
                    n2100 = global read "CurrentSwitchValues_GlobalVariable.vi" "12"() -> (w2054:bool)
                    n2101 = global read "CurrentSwitchValues_GlobalVariable.vi" "14"() -> (w2056:bool)
                    n2102 = global read "CurrentSwitchValues_GlobalVariable.vi" "16"() -> (w2058:bool)
                    n2103 = global read "CurrentSwitchValues_GlobalVariable.vi" "2"() -> (w2065:bool)
                    n2104 = global read "CurrentSwitchValues_GlobalVariable.vi" "6"() -> (w2062:bool)
                    n2105 = global read "CurrentSwitchValues_GlobalVariable.vi" "4"() -> (w2060:bool)
                    n2106 = global read "CurrentSwitchValues_GlobalVariable.vi" "8"() -> (w2064:bool)
                    n2107 = global read "CurrentSwitchValues_GlobalVariable.vi" "18"() -> (w2044:bool)
                    n2108 = global read "CurrentSwitchValues_GlobalVariable.vi" "20"() -> (w2046:bool)
                    n2109 = global read "CurrentSwitchValues_GlobalVariable.vi" "22"() -> (w2048:bool)
                    n2110 = global read "CurrentSwitchValues_GlobalVariable.vi" "24"() -> (w2050:bool)
                    n2111 = global read "CurrentSwitchValues_GlobalVariable.vi" "26"() -> (w2041:bool)
                    n2112 = global read "CurrentSwitchValues_GlobalVariable.vi" "28"() -> (w2039:bool)
                    n2113 = global read "CurrentSwitchValues_GlobalVariable.vi" "30"() -> (w2037:bool)
                    n2114 = property on="3" class="Bool (strict)"("Value"=w2059) -> ()  [unwired: 2 in, 2 out]
                    n2115 = property on="5" class="Bool (strict)"("Value"=w2061) -> ()  [unwired: 2 in, 2 out]
                    n2116 = property on="7" class="Bool (strict)"("Value"=w2063) -> ()  [unwired: 2 in, 2 out]
                    n2117 = property on="9" class="Bool (strict)"("Value"=w2051) -> ()  [unwired: 2 in, 2 out]
                    n2118 = property on="11" class="Bool (strict)"("Value"=w2053) -> ()  [unwired: 2 in, 2 out]
                    n2119 = property on="13" class="Bool (strict)"("Value"=w2055) -> ()  [unwired: 2 in, 2 out]
                    n2120 = property on="15" class="Bool (strict)"("Value"=w2057) -> ()  [unwired: 2 in, 2 out]
                    n2121 = property on="17" class="Bool (strict)"("Value"=w2043) -> ()  [unwired: 2 in, 2 out]
                    n2122 = property on="19" class="Bool (strict)"("Value"=w2045) -> ()  [unwired: 2 in, 2 out]
                    n2123 = property on="21" class="Bool (strict)"("Value"=w2047) -> ()  [unwired: 2 in, 2 out]
                    n2124 = property on="23" class="Bool (strict)"("Value"=w2049) -> ()  [unwired: 2 in, 2 out]
                    n2125 = property on="25" class="Bool (strict)"("Value"=w2042) -> ()  [unwired: 2 in, 2 out]
                    n2126 = property on="27" class="Bool (strict)"("Value"=w2040) -> ()  [unwired: 2 in, 2 out]
                    n2127 = property on="29" class="Bool (strict)"("Value"=w2038) -> ()  [unwired: 2 in, 2 out]
                    n2128 = property on="1" class="Bool (strict)"("Value"=w2066) -> ()  [unwired: 2 in, 2 out]
                    n2129 = property on="26" class="Bool (strict)"("Value"=w2041) -> ()  [unwired: 2 in, 2 out]
                    n2130 = property on="28" class="Bool (strict)"("Value"=w2039) -> ()  [unwired: 2 in, 2 out]
                    n2131 = property on="30" class="Bool (strict)"("Value"=w2037) -> ()  [unwired: 2 in, 2 out]
                    n2132 = property on="2" class="Bool (strict)"("Value"=w2065) -> ()  [unwired: 2 in, 2 out]
                    n2133 = property on="4" class="Bool (strict)"("Value"=w2060) -> ()  [unwired: 2 in, 2 out]
                    n2134 = property on="6" class="Bool (strict)"("Value"=w2062) -> ()  [unwired: 2 in, 2 out]
                    n2135 = property on="8" class="Bool (strict)"("Value"=w2064) -> ()  [unwired: 2 in, 2 out]
                    n2136 = property on="10" class="Bool (strict)"("Value"=w2052) -> ()  [unwired: 2 in, 2 out]
                    n2137 = property on="12" class="Bool (strict)"("Value"=w2054) -> ()  [unwired: 2 in, 2 out]
                    n2138 = property on="14" class="Bool (strict)"("Value"=w2056) -> ()  [unwired: 2 in, 2 out]
                    n2139 = property on="16" class="Bool (strict)"("Value"=w2058) -> ()  [unwired: 2 in, 2 out]
                    n2140 = property on="18" class="Bool (strict)"("Value"=w2044) -> ()  [unwired: 2 in, 2 out]
                    n2141 = property on="20" class="Bool (strict)"("Value"=w2046) -> ()  [unwired: 2 in, 2 out]
                    n2142 = property on="22" class="Bool (strict)"("Value"=w2048) -> ()  [unwired: 2 in, 2 out]
                    n2143 = property on="24" class="Bool (strict)"("Value"=w2050) -> ()  [unwired: 2 in, 2 out]
                  }
                }
              }
              frame #10 {
                # "Step 13: Before taking the first image of the experiment, the reaction chamber is mixed to ensure a homogeneous distribution of the reaction solvents."
                n2144 = stacked-sequence {
                  tunnel: w2067 -> [w2072 w2104 _]
                  tunnel: w2068 -> [w2071 w2103 _]
                  tunnel: [w2070 _ _] -> _
                  frame #0 {
                    n2145 = for {
                      N: 6 -> [_]
                      tunnel: w2072 -> [w2076]
                      tunnel: w2071 -> [w2075]
                      tunnel: [w2074] -> w2070
                      i -> [w2081]
                      n2146 = for {
                        N: 250 -> [_]
                        tunnel: w2076 -> [w2093]
                        tunnel: w2075 -> [w2092]
                        tunnel: [w2091] -> w2074
                        n2147 = for {
                          N: 6 -> [_]
                          tunnel: w2093 -> [w2097]
                          tunnel: w2092 -> [w2096]
                          tunnel: [w2095] -> w2091
                          i -> [w2100]
                          # "T-wait is 20 ms\nfreq = +-8.3Hz"
                          n2148 = Wait (ms)(milliseconds to wait=40) -> ()  [unwired: 1 out]
                          n2149 = Index Array(array=u8[][] [[0, 0, 0, 0, 0, 0, 0, 0, 2, 4, 3, 3, 3, 3], [0, 0, 0, 0, 0, 0, 0, 0, 0, 0, 0, 0, 0, 0], [0, 0, 0, 0, 0, 0, 0, 0, 0, 0, 0, 0, 0, 0], [0, 0, 0, 0, 0, 0, 0, 0, 0, 0, 0, 0, 0, 0], [0, 0, 0, 0, 0, 0, 0, 0, 0, 0, 0, 0, 0, 0], [11, 11, 11, 11, 11, 11, 11, 0, 0, 0, 0, 0, 0, 0], [0, 0, 0, 0, 0, 0, 0, 0, 0, 0, 0, 0, 0, 0], [16, 16, 16, 16, 16, 16, 16, 0, 0, 0, 0, 0, 0, 0], [0, 0, 0, 0, 0, 0, 0, 0, 0, 0, 0, 0, 0, 0], [0, 0, 0, 0, 0, 0, 0, 0, 0, 0, 0, 0, 0, 0], [0, 0, 0, 0, 0, 0, 0, 0, 0, 0, 0, 0, 0, 0], [2, 2, 2, 2, 2, 2, 2, 0, 0, 0, 0, 0, 0, 0], [4, 4, 4, 4, 4, 4, 4, 0, 0, 0, 0, 0, 0, 0], [255, 255, 255, 255, 255, 255, 0, 0, 0, 0, 0, 0, 0, 0], [3, 2, 6, 4, 5, 1, 0, 0, 0, 0, 0, 0, 0, 0], [27, 27, 27, 27, 27, 27, 0, 0, 0, 0, 0, 0, 0, 0], [255, 255, 255, 255, 255, 255, 0, 0, 0, 0, 0, 0, 0, 0]], index (col)=w2100) -> (element=w2101:u8[])  [unwired: 1 in]
                          n2150 = Byte Array To String(unsigned byte array=w2101) -> (string=w2098:string)
                          n2151 = call "StorePreviousSwitchValues.vi"("Array"=w2101) -> ()  [unwired: 3 in]
                          n2152 = Enqueue Element(queue=w2096, element=w2098, error in (no error)=w2097) -> (error out=w2095:errorcluster)  [unwired: 1 in, 2 out]
                        }
                      }
                      n2153 = Add(x=1, y=w2081) -> (x+y=w2077:i32)
                      n2154 = Less?(x=w2077, y=15) -> (x < y?=w2078:bool)
                      n2155 = case shown="True" w2078 {
                        frame False {
                        }
                        frame True {
                          n2156 = local read "Time between Mixing Cycles Initialisation"() -> (w2089:dbl)
                          n2157 = Multiply(x=60000, y=w2089) -> (x*y=w2083:dbl)
                          n2158 = Multiply(x=20, y=500) -> (x*y=w2086:i32)
                          n2159 = Multiply(x=w2086, y=6) -> (x*y=w2085:i32)
                          n2160 = Add(x=w2083, y=w2085) -> (x+y=w2082:dbl)
                          n2161 = Wait (ms)(milliseconds to wait=w2082) -> ()  [unwired: 1 out]
                        }
                      }
                    }
                  }
                  frame #1 {
                    w2106 = u8[] [0, 0, 0, 0, 0, 11, 0, 16, 0, 0, 0, 2, 4, 255, 7, 31, 255]
                    n2162 = call "StorePreviousSwitchValues.vi"("Array"=w2106) -> ()  [unwired: 3 in]
                    n2163 = Byte Array To String(unsigned byte array=w2106) -> (string=w2105:string)
                    n2164 = Enqueue Element(queue=w2103, element=w2105, error in (no error)=w2104) -> ()  [unwired: 1 in, 3 out]
                  }
                  frame #2 {
                    n2165 = global read "CurrentSwitchValues_GlobalVariable.vi" "1"() -> (w2136:bool)
                    n2166 = global read "CurrentSwitchValues_GlobalVariable.vi" "3"() -> (w2129:bool)
                    n2167 = global read "CurrentSwitchValues_GlobalVariable.vi" "5"() -> (w2131:bool)
                    n2168 = global read "CurrentSwitchValues_GlobalVariable.vi" "7"() -> (w2133:bool)
                    n2169 = global read "CurrentSwitchValues_GlobalVariable.vi" "9"() -> (w2121:bool)
                    n2170 = global read "CurrentSwitchValues_GlobalVariable.vi" "11"() -> (w2123:bool)
                    n2171 = global read "CurrentSwitchValues_GlobalVariable.vi" "13"() -> (w2125:bool)
                    n2172 = global read "CurrentSwitchValues_GlobalVariable.vi" "15"() -> (w2127:bool)
                    n2173 = global read "CurrentSwitchValues_GlobalVariable.vi" "17"() -> (w2113:bool)
                    n2174 = global read "CurrentSwitchValues_GlobalVariable.vi" "19"() -> (w2115:bool)
                    n2175 = global read "CurrentSwitchValues_GlobalVariable.vi" "21"() -> (w2117:bool)
                    n2176 = global read "CurrentSwitchValues_GlobalVariable.vi" "23"() -> (w2119:bool)
                    n2177 = global read "CurrentSwitchValues_GlobalVariable.vi" "25"() -> (w2112:bool)
                    n2178 = global read "CurrentSwitchValues_GlobalVariable.vi" "27"() -> (w2110:bool)
                    n2179 = global read "CurrentSwitchValues_GlobalVariable.vi" "29"() -> (w2108:bool)
                    n2180 = global read "CurrentSwitchValues_GlobalVariable.vi" "10"() -> (w2122:bool)
                    n2181 = global read "CurrentSwitchValues_GlobalVariable.vi" "12"() -> (w2124:bool)
                    n2182 = global read "CurrentSwitchValues_GlobalVariable.vi" "14"() -> (w2126:bool)
                    n2183 = global read "CurrentSwitchValues_GlobalVariable.vi" "16"() -> (w2128:bool)
                    n2184 = global read "CurrentSwitchValues_GlobalVariable.vi" "2"() -> (w2135:bool)
                    n2185 = global read "CurrentSwitchValues_GlobalVariable.vi" "6"() -> (w2132:bool)
                    n2186 = global read "CurrentSwitchValues_GlobalVariable.vi" "4"() -> (w2130:bool)
                    n2187 = global read "CurrentSwitchValues_GlobalVariable.vi" "8"() -> (w2134:bool)
                    n2188 = global read "CurrentSwitchValues_GlobalVariable.vi" "18"() -> (w2114:bool)
                    n2189 = global read "CurrentSwitchValues_GlobalVariable.vi" "20"() -> (w2116:bool)
                    n2190 = global read "CurrentSwitchValues_GlobalVariable.vi" "22"() -> (w2118:bool)
                    n2191 = global read "CurrentSwitchValues_GlobalVariable.vi" "24"() -> (w2120:bool)
                    n2192 = global read "CurrentSwitchValues_GlobalVariable.vi" "26"() -> (w2111:bool)
                    n2193 = global read "CurrentSwitchValues_GlobalVariable.vi" "28"() -> (w2109:bool)
                    n2194 = global read "CurrentSwitchValues_GlobalVariable.vi" "30"() -> (w2107:bool)
                    n2195 = property on="1" class="Bool (strict)"("Value"=w2136) -> ()  [unwired: 2 in, 2 out]
                    n2196 = property on="3" class="Bool (strict)"("Value"=w2129) -> ()  [unwired: 2 in, 2 out]
                    n2197 = property on="5" class="Bool (strict)"("Value"=w2131) -> ()  [unwired: 2 in, 2 out]
                    n2198 = property on="7" class="Bool (strict)"("Value"=w2133) -> ()  [unwired: 2 in, 2 out]
                    n2199 = property on="9" class="Bool (strict)"("Value"=w2121) -> ()  [unwired: 2 in, 2 out]
                    n2200 = property on="11" class="Bool (strict)"("Value"=w2123) -> ()  [unwired: 2 in, 2 out]
                    n2201 = property on="13" class="Bool (strict)"("Value"=w2125) -> ()  [unwired: 2 in, 2 out]
                    n2202 = property on="15" class="Bool (strict)"("Value"=w2127) -> ()  [unwired: 2 in, 2 out]
                    n2203 = property on="17" class="Bool (strict)"("Value"=w2113) -> ()  [unwired: 2 in, 2 out]
                    n2204 = property on="19" class="Bool (strict)"("Value"=w2115) -> ()  [unwired: 2 in, 2 out]
                    n2205 = property on="21" class="Bool (strict)"("Value"=w2117) -> ()  [unwired: 2 in, 2 out]
                    n2206 = property on="23" class="Bool (strict)"("Value"=w2119) -> ()  [unwired: 2 in, 2 out]
                    n2207 = property on="25" class="Bool (strict)"("Value"=w2112) -> ()  [unwired: 2 in, 2 out]
                    n2208 = property on="27" class="Bool (strict)"("Value"=w2110) -> ()  [unwired: 2 in, 2 out]
                    n2209 = property on="29" class="Bool (strict)"("Value"=w2108) -> ()  [unwired: 2 in, 2 out]
                    n2210 = property on="26" class="Bool (strict)"("Value"=w2111) -> ()  [unwired: 2 in, 2 out]
                    n2211 = property on="28" class="Bool (strict)"("Value"=w2109) -> ()  [unwired: 2 in, 2 out]
                    n2212 = property on="30" class="Bool (strict)"("Value"=w2107) -> ()  [unwired: 2 in, 2 out]
                    n2213 = property on="2" class="Bool (strict)"("Value"=w2135) -> ()  [unwired: 2 in, 2 out]
                    n2214 = property on="4" class="Bool (strict)"("Value"=w2130) -> ()  [unwired: 2 in, 2 out]
                    n2215 = property on="6" class="Bool (strict)"("Value"=w2132) -> ()  [unwired: 2 in, 2 out]
                    n2216 = property on="8" class="Bool (strict)"("Value"=w2134) -> ()  [unwired: 2 in, 2 out]
                    n2217 = property on="10" class="Bool (strict)"("Value"=w2122) -> ()  [unwired: 2 in, 2 out]
                    n2218 = property on="12" class="Bool (strict)"("Value"=w2124) -> ()  [unwired: 2 in, 2 out]
                    n2219 = property on="14" class="Bool (strict)"("Value"=w2126) -> ()  [unwired: 2 in, 2 out]
                    n2220 = property on="16" class="Bool (strict)"("Value"=w2128) -> ()  [unwired: 2 in, 2 out]
                    n2221 = property on="18" class="Bool (strict)"("Value"=w2114) -> ()  [unwired: 2 in, 2 out]
                    n2222 = property on="20" class="Bool (strict)"("Value"=w2116) -> ()  [unwired: 2 in, 2 out]
                    n2223 = property on="22" class="Bool (strict)"("Value"=w2118) -> ()  [unwired: 2 in, 2 out]
                    n2224 = property on="24" class="Bool (strict)"("Value"=w2120) -> ()  [unwired: 2 in, 2 out]
                  }
                }
              }
              frame #11 {
                # "Step 1:\nThe primary step in this simple expression\nprotocol is to flush the device with elution \nbuffer to ensure the removal of any residual\nsolutes from the calibration protocol."
                n2225 = stacked-sequence {
                  tunnel: w2138 -> [w2141 w2156 _]
                  tunnel: w2137 -> [w2140 w2157 _]
                  tunnel: [w2139 _ _] -> _
                  frame #0 {
                    n2226 = for {
                      N: 500 -> [_]
                      tunnel: w2141 -> [w2145]
                      tunnel: w2140 -> [w2144]
                      tunnel: [w2143] -> w2139
                      n2227 = for {
                        N: 6 -> [_]
                        tunnel: w2145 -> [w2150]
                        tunnel: w2144 -> [w2149]
                        tunnel: [w2148] -> w2143
                        i -> [w2154]
                        # "T-wait is 100 ms,\nfreq = +-1.7Hz if fast and T-wait is 556ms, freq = 0.3Hz if slow flush."
                        n2228 = local read "Elution Buffer"() -> (w2147:dbl)
                        n2229 = call "SequenceSelector_Flush.vi"("Inflow Channel Selector"=w2147) -> ("Array"=w2153:u8[][])
                        n2230 = Wait (ms)(milliseconds to wait=25) -> ()  [unwired: 1 out]
                        n2231 = Index Array(array=w2153, index (col)=w2154) -> (element=w2155:u8[])  [unwired: 1 in]
                        n2232 = call "StorePreviousSwitchValues.vi"("Array"=w2155) -> ()  [unwired: 3 in]
                        n2233 = Byte Array To String(unsigned byte array=w2155) -> (string=w2151:string)
                        n2234 = Enqueue Element(queue=w2149, element=w2151, error in (no error)=w2150) -> (error out=w2148:errorcluster)  [unwired: 1 in, 2 out]
                      }
                    }
                  }
                  frame #1 {
                    w2159 = u8[] [0, 0, 0, 0, 0, 11, 0, 16, 0, 0, 0, 2, 4, 255, 7, 31, 255]
                    n2235 = call "StorePreviousSwitchValues.vi"("Array"=w2159) -> ()  [unwired: 3 in]
                    n2236 = Byte Array To String(unsigned byte array=w2159) -> (string=w2158:string)
                    n2237 = Enqueue Element(queue=w2157, element=w2158, error in (no error)=w2156) -> ()  [unwired: 1 in, 3 out]
                  }
                  frame #2 {
                    n2238 = global read "CurrentSwitchValues_GlobalVariable.vi" "1"() -> (w2189:bool)
                    n2239 = global read "CurrentSwitchValues_GlobalVariable.vi" "3"() -> (w2182:bool)
                    n2240 = global read "CurrentSwitchValues_GlobalVariable.vi" "5"() -> (w2184:bool)
                    n2241 = global read "CurrentSwitchValues_GlobalVariable.vi" "7"() -> (w2186:bool)
                    n2242 = global read "CurrentSwitchValues_GlobalVariable.vi" "9"() -> (w2174:bool)
                    n2243 = global read "CurrentSwitchValues_GlobalVariable.vi" "11"() -> (w2176:bool)
                    n2244 = global read "CurrentSwitchValues_GlobalVariable.vi" "13"() -> (w2178:bool)
                    n2245 = global read "CurrentSwitchValues_GlobalVariable.vi" "15"() -> (w2180:bool)
                    n2246 = global read "CurrentSwitchValues_GlobalVariable.vi" "17"() -> (w2166:bool)
                    n2247 = global read "CurrentSwitchValues_GlobalVariable.vi" "19"() -> (w2168:bool)
                    n2248 = global read "CurrentSwitchValues_GlobalVariable.vi" "21"() -> (w2170:bool)
                    n2249 = global read "CurrentSwitchValues_GlobalVariable.vi" "23"() -> (w2172:bool)
                    n2250 = global read "CurrentSwitchValues_GlobalVariable.vi" "25"() -> (w2165:bool)
                    n2251 = global read "CurrentSwitchValues_GlobalVariable.vi" "27"() -> (w2163:bool)
                    n2252 = global read "CurrentSwitchValues_GlobalVariable.vi" "29"() -> (w2161:bool)
                    n2253 = global read "CurrentSwitchValues_GlobalVariable.vi" "10"() -> (w2175:bool)
                    n2254 = global read "CurrentSwitchValues_GlobalVariable.vi" "12"() -> (w2177:bool)
                    n2255 = global read "CurrentSwitchValues_GlobalVariable.vi" "14"() -> (w2179:bool)
                    n2256 = global read "CurrentSwitchValues_GlobalVariable.vi" "16"() -> (w2181:bool)
                    n2257 = global read "CurrentSwitchValues_GlobalVariable.vi" "2"() -> (w2188:bool)
                    n2258 = global read "CurrentSwitchValues_GlobalVariable.vi" "6"() -> (w2185:bool)
                    n2259 = global read "CurrentSwitchValues_GlobalVariable.vi" "4"() -> (w2183:bool)
                    n2260 = global read "CurrentSwitchValues_GlobalVariable.vi" "8"() -> (w2187:bool)
                    n2261 = global read "CurrentSwitchValues_GlobalVariable.vi" "18"() -> (w2167:bool)
                    n2262 = global read "CurrentSwitchValues_GlobalVariable.vi" "20"() -> (w2169:bool)
                    n2263 = global read "CurrentSwitchValues_GlobalVariable.vi" "22"() -> (w2171:bool)
                    n2264 = global read "CurrentSwitchValues_GlobalVariable.vi" "24"() -> (w2173:bool)
                    n2265 = global read "CurrentSwitchValues_GlobalVariable.vi" "26"() -> (w2164:bool)
                    n2266 = global read "CurrentSwitchValues_GlobalVariable.vi" "28"() -> (w2162:bool)
                    n2267 = global read "CurrentSwitchValues_GlobalVariable.vi" "30"() -> (w2160:bool)
                    n2268 = property on="1" class="Bool (strict)"("Value"=w2189) -> ()  [unwired: 2 in, 2 out]
                    n2269 = property on="3" class="Bool (strict)"("Value"=w2182) -> ()  [unwired: 2 in, 2 out]
                    n2270 = property on="5" class="Bool (strict)"("Value"=w2184) -> ()  [unwired: 2 in, 2 out]
                    n2271 = property on="7" class="Bool (strict)"("Value"=w2186) -> ()  [unwired: 2 in, 2 out]
                    n2272 = property on="9" class="Bool (strict)"("Value"=w2174) -> ()  [unwired: 2 in, 2 out]
                    n2273 = property on="11" class="Bool (strict)"("Value"=w2176) -> ()  [unwired: 2 in, 2 out]
                    n2274 = property on="13" class="Bool (strict)"("Value"=w2178) -> ()  [unwired: 2 in, 2 out]
                    n2275 = property on="15" class="Bool (strict)"("Value"=w2180) -> ()  [unwired: 2 in, 2 out]
                    n2276 = property on="17" class="Bool (strict)"("Value"=w2166) -> ()  [unwired: 2 in, 2 out]
                    n2277 = property on="19" class="Bool (strict)"("Value"=w2168) -> ()  [unwired: 2 in, 2 out]
                    n2278 = property on="21" class="Bool (strict)"("Value"=w2170) -> ()  [unwired: 2 in, 2 out]
                    n2279 = property on="23" class="Bool (strict)"("Value"=w2172) -> ()  [unwired: 2 in, 2 out]
                    n2280 = property on="25" class="Bool (strict)"("Value"=w2165) -> ()  [unwired: 2 in, 2 out]
                    n2281 = property on="27" class="Bool (strict)"("Value"=w2163) -> ()  [unwired: 2 in, 2 out]
                    n2282 = property on="29" class="Bool (strict)"("Value"=w2161) -> ()  [unwired: 2 in, 2 out]
                    n2283 = property on="26" class="Bool (strict)"("Value"=w2164) -> ()  [unwired: 2 in, 2 out]
                    n2284 = property on="28" class="Bool (strict)"("Value"=w2162) -> ()  [unwired: 2 in, 2 out]
                    n2285 = property on="30" class="Bool (strict)"("Value"=w2160) -> ()  [unwired: 2 in, 2 out]
                    n2286 = property on="2" class="Bool (strict)"("Value"=w2188) -> ()  [unwired: 2 in, 2 out]
                    n2287 = property on="4" class="Bool (strict)"("Value"=w2183) -> ()  [unwired: 2 in, 2 out]
                    n2288 = property on="6" class="Bool (strict)"("Value"=w2185) -> ()  [unwired: 2 in, 2 out]
                    n2289 = property on="8" class="Bool (strict)"("Value"=w2187) -> ()  [unwired: 2 in, 2 out]
                    n2290 = property on="10" class="Bool (strict)"("Value"=w2175) -> ()  [unwired: 2 in, 2 out]
                    n2291 = property on="12" class="Bool (strict)"("Value"=w2177) -> ()  [unwired: 2 in, 2 out]
                    n2292 = property on="14" class="Bool (strict)"("Value"=w2179) -> ()  [unwired: 2 in, 2 out]
                    n2293 = property on="16" class="Bool (strict)"("Value"=w2181) -> ()  [unwired: 2 in, 2 out]
                    n2294 = property on="18" class="Bool (strict)"("Value"=w2167) -> ()  [unwired: 2 in, 2 out]
                    n2295 = property on="20" class="Bool (strict)"("Value"=w2169) -> ()  [unwired: 2 in, 2 out]
                    n2296 = property on="22" class="Bool (strict)"("Value"=w2171) -> ()  [unwired: 2 in, 2 out]
                    n2297 = property on="24" class="Bool (strict)"("Value"=w2173) -> ()  [unwired: 2 in, 2 out]
                  }
                }
              }
              frame #12 {
                # "Let the Microscope know that the sequence has ended and\nstop waiting for new commands."
                # "Before finishing the experiment, the reactors are mixed a final time (previous step) and an image is taken of the current conditions in the reactor."
                n2298 = call <vilib>:"System Exec.vi"("command line"="C:\\Users\\avdlinde\\Desktop\\Labview Interface for Jove Paper\\dummy_stopper.exe") -> ()  [unwired: 7 in, 4 out]
              }
            }
            "Running Experiments" <- TRUE
          }
          event "stop": Value Change {
            w2195 = FALSE
            w2196 = u8[] [0, 0, 0, 0, 0, 11, 0, 16, 0, 0, 0, 2, 4, 0, 0, 0, 0]
            n2299 = event-data() -> ()  [unwired: 1 in, 6 out]
            n2300 = property on="1" class="Bool (strict)"("Value"=w2195) -> ()  [unwired: 2 in, 2 out]
            n2301 = property on="2" class="Bool (strict)"("Value"=w2195) -> ()  [unwired: 2 in, 2 out]
            n2302 = property on="3" class="Bool (strict)"("Value"=w2195) -> ()  [unwired: 2 in, 2 out]
            n2303 = property on="4" class="Bool (strict)"("Value"=w2195) -> ()  [unwired: 2 in, 2 out]
            n2304 = property on="5" class="Bool (strict)"("Value"=w2195) -> ()  [unwired: 2 in, 2 out]
            n2305 = property on="6" class="Bool (strict)"("Value"=w2195) -> ()  [unwired: 2 in, 2 out]
            n2306 = property on="7" class="Bool (strict)"("Value"=w2195) -> ()  [unwired: 2 in, 2 out]
            n2307 = property on="8" class="Bool (strict)"("Value"=w2195) -> ()  [unwired: 2 in, 2 out]
            n2308 = property on="9" class="Bool (strict)"("Value"=w2195) -> ()  [unwired: 2 in, 2 out]
            n2309 = property on="11" class="Bool (strict)"("Value"=w2195) -> ()  [unwired: 2 in, 2 out]
            n2310 = property on="10" class="Bool (strict)"("Value"=w2195) -> ()  [unwired: 2 in, 2 out]
            n2311 = property on="12" class="Bool (strict)"("Value"=w2195) -> ()  [unwired: 2 in, 2 out]
            n2312 = property on="13" class="Bool (strict)"("Value"=w2195) -> ()  [unwired: 2 in, 2 out]
            n2313 = property on="15" class="Bool (strict)"("Value"=w2195) -> ()  [unwired: 2 in, 2 out]
            n2314 = property on="14" class="Bool (strict)"("Value"=w2195) -> ()  [unwired: 2 in, 2 out]
            n2315 = property on="16" class="Bool (strict)"("Value"=w2195) -> ()  [unwired: 2 in, 2 out]
            n2316 = property on="17" class="Bool (strict)"("Value"=w2195) -> ()  [unwired: 2 in, 2 out]
            n2317 = property on="18" class="Bool (strict)"("Value"=w2195) -> ()  [unwired: 2 in, 2 out]
            n2318 = property on="19" class="Bool (strict)"("Value"=w2195) -> ()  [unwired: 2 in, 2 out]
            n2319 = property on="20" class="Bool (strict)"("Value"=w2195) -> ()  [unwired: 2 in, 2 out]
            n2320 = property on="21" class="Bool (strict)"("Value"=w2195) -> ()  [unwired: 2 in, 2 out]
            n2321 = property on="22" class="Bool (strict)"("Value"=w2195) -> ()  [unwired: 2 in, 2 out]
            n2322 = property on="23" class="Bool (strict)"("Value"=w2195) -> ()  [unwired: 2 in, 2 out]
            n2323 = property on="24" class="Bool (strict)"("Value"=w2195) -> ()  [unwired: 2 in, 2 out]
            n2324 = property on="25" class="Bool (strict)"("Value"=w2195) -> ()  [unwired: 2 in, 2 out]
            n2325 = property on="27" class="Bool (strict)"("Value"=w2195) -> ()  [unwired: 2 in, 2 out]
            n2326 = property on="26" class="Bool (strict)"("Value"=w2195) -> ()  [unwired: 2 in, 2 out]
            n2327 = property on="28" class="Bool (strict)"("Value"=w2195) -> ()  [unwired: 2 in, 2 out]
            n2328 = property on="29" class="Bool (strict)"("Value"=w2195) -> ()  [unwired: 2 in, 2 out]
            n2329 = property on="30" class="Bool (strict)"("Value"=w2195) -> ()  [unwired: 2 in, 2 out]
            n2330 = Byte Array To String(unsigned byte array=w2196) -> (string=w2193:string)
            n2331 = call "StorePreviousSwitchValues.vi"("Array"=w2196) -> ()  [unwired: 3 in]
            n2332 = Enqueue Element(queue=w2194, element=w2193, error in (no error)=w2192) -> (error out=w2191:errorcluster)  [unwired: 1 in, 2 out]
          }
        }
        n2333 = Wait Until Next ms Multiple(millisecond multiple=10) -> ()  [unwired: 1 out]
      }
      n2334 = while {
        tunnel: w10 -> [w39]
        tunnel: w9 -> [w38]
        tunnel: [w37] -> w8
        tunnel: [w36] -> w7
        tunnel: w4 -> [w35]
        tunnel: w3 -> [w34]
        tunnel: [w33] -> w6
        tunnel: [w32] -> w5
        stop <- w31 stop-if-true
        n2335 = Dequeue Element(queue=w35, error in (no error)=w34) -> (queue out=w32:refnum<queue>, element=w30:string, error out=w33:errorcluster)  [unwired: 1 in, 1 out]
        n2336 = global read "TCPRead_Write_GlobalVariables.vi" "Bytes Written"() -> (w40:dbl)
        "Bytes Written (Per Command)" <- w40
        n2337 = property on="Bytes Written (Total)" class="DigNum (strict)"() -> ("Value"=w41:i32)  [unwired: 2 in, 2 out]
        n2338 = Add(x=w41, y=w40) -> (x+y=→"Bytes Written (Total)":dbl)
        n2339 = global read "TCPRead_Write_GlobalVariables.vi" "TCP Output"() -> (→"TCP Output":string)
        n2340 = local read "stop"() -> (w31:bool)
        n2341 = call "TCPRead_Write.vi"("String"=w30, "error out 2"=w38, "connection ID 2"=w39) -> ("error out"=w36:errorcluster, "connection ID"=w37:refnum<k5>)  [unwired: 7 in]
        "TCP Error Out" <- w36
      }
      n2342 = TCP Close Connection(connection ID=w8, error in (no error)=w7) -> (error out=w14:errorcluster)  [unwired: 1 in, 1 out]
      n2343 = call <vilib>:"Simple Error Handler.vi"("error in (no error)"=w14) -> ()  [unwired: 4 in, 5 out]
      n2344 = Merge Errors(w6, w13) -> (w12:errorcluster)
      n2345 = Release Queue(queue=w5, error in (no error)=w12) -> ()  [unwired: 1 in, 3 out]
    }
  }
